vi "TrapControllers.vi"() -> ()   [LabVIEW 2017]
doc: "I. Description:\nThis example demonstrates how to continuously output a waveform using an internal sample clock. The automatic regeneration of data has been disabled, so new data has to be provided throughout the duration of the continuous Analog Output operation. This allows the generation of any arbitrary frequency as this VI computes new data for each iteration of the loop, maintaining phase continuity of the signal. The regeneration of data has also been adjusted so that the newest data is output as quickly as possible; thus reducing the lag between the changing of the data and the output of that data.\n\nII. Instructions for Running:\n1. Select the Physical Channel to correspond to where your signal is output on the DAQ device.\n2. Enter the Minimum and Maximum Voltage range.\n3. Specify the desired Sample Clock Rate of the output Waveform. Higher sample clock rates will produce a smoother waveform.\n4. Manually specify the Analog Output buffer size, in number of samples. A larger buffer would help non-regenerative operations avoid errors due to occasional high CPU load. \nNote: \nThe Analog Output buffer has to be at least as big as the amount of data being written to the board per iteration. The recommended buffer size would be at least twice the amount of data being written to the board per iteration.\n5. Enter the Waveform Information. See the documentation of the Basic Function Generator SubVI for information on each parameter.\n\nIII. Block Diagram Steps:\n1. Create an Analog Output Voltage channel.\n2. Configure the task to prohibit the automatic regeneration of data.\n2a. Set the transfer condition to Less than Full. Allows for more rapid updates of Output Buffer.\n3. Call the DAQmx (Sample Clock) VI to set the sample clock rate. Additionally, set the sample mode to Continuous.\n4. Read the actual sample clock rate (eventually coerced depending on the hardware used). \n5. Compute the desired waveform, using the buffer size and the actual update rate. This VI keeps track of the phase of the waveform to ensure that the generated signal is continuous.\n6. Write the waveform to the output buffer. \n7a. Call the Start VI. This is only needed when the loop is executed for the first time.\n7b. Do nothing.\n8. Loop continuously until user presses the Stop button. Every iteration computes and writes a new waveform to the buffer.\n9. Call the Clear Task VI to clear the Task.\n10. Use the popup dialog box to display an error or warning if any.\n\nIV. I/O Connections Overview:\nMake sure your signal output terminal matches the Physical Channel I/O Control. For further connection information, refer to your hardware reference manual."
uses:
  <vilib>/event_ctls.llb/eventvkey.ctl
  C:/Program Files/National Instruments/LabVIEW 2017/user.lib/Picomotor_8742/CmdLib.dll
  Program Files/National Instruments/LabVIEW 2017/user.lib/Picomotor_8742/CmdLib.dll
  <vilib>/DAQmx/write.llb/DAQmx Write (Analog DBL 1Chan 1Samp).vi
  <vilib>/DAQmx/write.llb/DAQmx Write (Digital 1D Bool NChan 1Samp 1Line).vi
  <vilib>/DAQmx/write.llb/DAQmx Write (Analog 1D DBL NChan 1Samp).vi
  <vilib>/DAQmx/create/channels.llb/DAQmx Create Channel (AO-Voltage-Basic).vi
  <vilib>/DAQmx/miscellaneous.llb/DAQmx Fill In Error Info.vi
  <vilib>/DAQmx/create/channels.llb/DAQmx Create Channel (DO-Digital Output).vi
  TrapSignal/Feedback.vi
  <vilib>/addons/control/pid/pid.llb/PID (DBL).vi
  PZT_PI/PZT_oscillation.vi
  <vilib>/addons/control/pid/NI_PID_pid.lvlib
  <vilib>/measure/NI_MABase.lvlib
panel:
  in  "Flu_Red_Run 2":bool caption="ON/OFF"
  out "LED_Power":dbl=3.0 caption="P (%)" min=0.0 max=100.0 step=1.0
  in  "LED_Power2":dbl=100.0 caption="P (%)" min=0.0 max=100.0 step=1.0
  in  "Trap_Power_Run 3":bool caption="Feedback"
  in  "MTAx_Feedback_dt 2":dbl=1.0 caption="Time (s)" format="%.1f"
  in  "?":cluster{dbl, dbl, dbl}={1.0, 0.01, 0.0} {"?" format="%.3f"; "?" format="%.3f"; "?" format="%.3f"}
  in  "Trap_Power_Run 2":bool caption="ON/Reset"
  in  "MTAy_Feedback_Reset":bool caption="Reset"
  in  "MTAy_Feedback_ON":bool caption="ON/Reset"
  in  "MTAy_Feedback_Min":dbl min=0.0 max=10.0 step=0.1 format="%#_2g"
  in  "MTAx_Feedback_Min":dbl caption="Min (pN)" min=0.0 max=10.0 step=0.1 format="%#_2g"
  in  "MTAy_Feedback_Max":dbl=0.01 min=0.0 max=10.0 step=0.1 format="%#_2g"
  in  "MTAx_Feedback_Reset":bool caption="Reset"
  in  "MTAx_Feedback_ON":bool caption="ON/Reset"
  in  "MTAy_Feedback_Force":dbl caption="Y" min=-10.0 max=10.0 step=0.1 format="%.1f"
  in  "?":cluster{dbl, dbl, dbl}={1.0, 5.0, 0.0} {"?" format="%.3f"; "?" format="%.3f"; "?" format="%.3f"}
  in  "MTAy_Feedback_dt":dbl=1.0 caption="Time (s)" format="%.1f"
  in  "MTAx_Feedback_Force":dbl caption="X" min=-10.0 max=10.0 step=0.1 format="%.1f"
  in  "?":cluster{dbl, dbl, dbl}={1.0, 5.0, 0.0} {"?" format="%.3f"; "?" format="%.3f"; "?" format="%.3f"}
  in  "MTAx_Feedback_dt":dbl=1.0 caption="Time (s)" format="%.1f"
  in  "MTAx_Feedback_Max":dbl=0.01 caption="Max (um)" min=0.0 max=10.0 step=0.1 format="%#_2g"
  in  "PM_Feedback":bool caption="ON/OFF"
  out "MTA_Limit":bool caption="Limit"
  out "MTA_Os_Num":i32
  in  "PZT_Speed 2":dbl=100.0 caption="Vel (%)" min=0.0 max=100.0 step=1.0
  in  "MTA_Select":bool caption="MTA1"
  out "MTA_Step":dbl=10.0 caption="Step (V)" min=0.0 max=1000.0 step=0.1 format="%.3f"
  in  "MTA_Step2":dbl=0.01 caption="Step2" min=0.0 max=1.0 step=0.001 format="%.3f"
  in  "MTA_Step_Select":bool=TRUE caption="(Y)"
  in  "MTA_Step1":dbl=0.1 caption="Step1" min=0.0 max=1.0 step=0.001 format="%.3f"
  in  "MTAY-":bool
  in  "MTAY+":bool
  in  "MTAX+":bool
  in  "MTAX-":bool
  out "MTA2Y":dbl caption="Pos (um)" format="%.3f"
  out "MTA2X":dbl caption="Pos (um)" format="%.3f"
  out "MTA1Y":dbl caption="Y" format="%.3f"
  out "MTA1X":dbl caption="X" format="%.3f"
  out "MTA_Manual_ON":bool caption="Manual"
  in  "MTA_Zero":bool
  in  "MTA_Home":bool
  in  "MTA_STOP":bool
  out "MTA_Man_Num":i32
  out "MTA_ON":bool
  in  "MTA_START":bool
  in  "STOP 2":bool
  in  "PZT_Zero":bool
  in  "LED_Power 2":dbl=10.0 caption="TIRF angle" min=0.0 max=100.0 step=1.0
  in  "LED_STOP":bool
  out "LED_Num":i32
  in  "LED_Run":bool caption="P (%)"
  out "LED_ON":bool
  in  "LED_Power1":dbl=10.0 caption="P (%)" min=0.0 max=100.0 step=1.0
  in  "LED_START":bool
  out "PZT_Manual_ON":bool caption="Manual"
  out "PZTZ_Step":dbl=10.0 caption="Step (nm)" min=0.0 max=1000.0 step=1.0
  in  "PZTZ_Step2":dbl=20.0 caption="Step (nm)" min=0.0 max=1000.0 step=1.0
  in  "PZTZ_Step1":dbl=100.0 caption="Step (nm)" min=0.0 max=1000.0 step=1.0
  out "PZTY_Step":dbl=10.0 caption="Step (nm)" min=0.0 max=1000.0 step=1.0
  in  "PZTY_Step2":dbl=20.0 caption="Step (nm)" min=0.0 max=1000.0 step=1.0
  in  "PZTY_Step1":dbl=100.0 caption="Step (nm)" min=0.0 max=1000.0 step=1.0
  out "PZTZ_Limit":bool caption="Limit"
  out "PZTY_Limit":bool caption="Limit"
  out "PZTX_Step":dbl=10.0 caption="Step (nm)" min=0.0 max=1000.0 step=1.0
  in  "PZTX_Step2":dbl=20.0 caption="Step (nm)" min=0.0 max=1000.0 step=1.0
  in  "PZT_Step_Select":bool=TRUE caption="(Del)"
  in  "Det_Select":bool caption="Det 1"
  out "Det_Step":dbl=10.0 caption="Step (um)" min=0.0 max=1000.0 step=0.1
  in  "Det2_Offset":bool
  in  "Det1_Offset":bool
  in  "Det2_Home":bool
  out "Detection2Y_Position":dbl caption="Pos (um)"
  out "Detection2X_Position":dbl caption="Pos (um)"
  out "Detection1Y_Position":dbl caption="Y"
  in  "Det_Step2":dbl=1.0 caption="Step2" min=0.0 max=100.0 step=1.0
  in  "Detection_Step_Select":bool=TRUE caption="(O)"
  in  "Det_Step1":dbl=10.0 caption="Step1" min=0.0 max=100.0 step=1.0
  in  "Det1_Home":bool
  out "Detection1X_Position":dbl caption="X"
  in  "Det_Position_STOP":bool
  out "Det_Position_Num":i32
  in  "Det_Position_START":bool
  out "Detection_Position_ON":bool caption="Picomotor"
  in  "DetY-":bool
  in  "DetY+":bool
  in  "DetX+":bool
  in  "DetX-":bool
  in  "Detection_Power":dbl=50.0 caption="Power (%)" min=0.0 max=100.0 step=1.0
  out "Controllers_ON":bool
  in  "Trap_Select":bool caption="Trap1"
  out "Trap_Step":dbl=10.0 caption="Step (um)" min=0.0 max=1000.0 step=0.1
  in  "Trap2_Offset":bool
  in  "Trap1_Offset":bool
  in  "Trap2_Home":bool
  out "PicomotorError":errorcluster
  out "PicomotorDevice2":string
  out "PicomotorCmdLib":refnum<k24>
  out "PicomotorDevice1":string
  out "Trap2Y_Position":dbl caption="Pos (um)"
  out "Trap2X_Position":dbl caption="Pos (um)"
  out "Trap1Y_Position":dbl caption="Y"
  in  "Trap_Step2":dbl=1.0 caption="Step2" min=0.0 max=100.0 step=1.0
  in  "Trap_Step_Select":bool=TRUE caption="(E)"
  in  "Trap_Step1":dbl=10.0 caption="Step1" min=0.0 max=100.0 step=1.0
  in  "Trap1_Home":bool
  out "Trap1X_Position":dbl caption="X"
  in  "Trap_Position_STOP":bool
  out "Trap_Position_Num":i32
  in  "Trap_Position_START":bool
  out "PZT_Man_Num":i32
  in  "PZTX_Step1":dbl=100.0 caption="Step (nm)" min=0.0 max=1000.0 step=1.0
  out "PZTZ_Position":dbl caption="Z"
  out "PZTY_Position":dbl caption="Y"
  out "PZTX_Position":dbl caption="X"
  out "PZTX_Limit":bool caption="Limit"
  in  "PZT_Speed":dbl=100.0 caption="Vel (%)" min=0.0 max=100.0 step=1.0
  in  "PZT_Home":bool
  in  "PZT_Z-":bool
  in  "PZT_Z+":bool
  in  "PZT_Y-":bool
  in  "PZT_Y+":bool
  in  "PZT_X+":bool
  in  "PZT_X-":bool
  in  "PZT_oscillation_Run":bool caption="Start (Shift)"
  out "PZT_Os_Num":i32
  in  "PZT_Amplitude":dbl=50.0 caption="Amp (nm)" min=0.0 max=100.0 step=1.0
  in  "PZT_Frequency":dbl=100.0 caption="Freq (Hz)" min=0.0 max=100.0 step=1.0
  in  "PZT_Waveform":enum16{"Sine", "Triangle", "Square", "Sawtooth"}(ring) caption="Waveform"
  in  "PZT_Axis":enum16{"X", "Y", "Z"}(ring) caption="Axis"
  out "PZT_ON":bool
  in  "PZT_START":bool
  in  "PZT_STOP":bool
  out "Trap_Position_ON":bool caption="Picomotor"
  in  "TrapY-":bool
  in  "TrapY+":bool
  in  "TrapX+":bool
  in  "TrapX-":bool
  in  "Trap_Power_Run":bool caption="ON/OFF"
  in  "Trap_Power_Input":dbl=20.0 caption="%" min=0.0 max=100.0 step=1.0
  in  "Trap_Power_STOP":bool
  out "Trap_Power_Num":i32
  in  "Trap_Power_START":bool
  out "Trap_Power_ON":bool caption="Power"
  in  "StageY_Home 2":bool
  in  "VISA_Close":bool caption="Close"
  in  "StageZ_Step2":dbl=1.0 caption="Step2" min=0.0 max=10.0 step=0.01 format="%.2f"
  in  "StageZ_Step1":dbl=2.0 caption="Step1" min=0.0 max=10.0 step=0.01 format="%.2f"
  out "StageZ_Step":dbl=10.0 caption="Step (um)" min=0.0 max=1000.0 step=0.1 format="%.2f"
  out "StageZ_ON":bool caption="Z"
  out "StageZ_Position":dbl caption="Position" format="%.2f"
  in  "VISA_Selection":refnum<visa-resource-name> caption="VISA"
  in  "StageZ_Start":bool
  in  "StageY_Start":bool
  out "StageY_ON":bool caption="Y"
  in  "StageY_Home":bool
  out "StageY_Position":dbl caption="Pos (um)" format="%.1f"
  in  "StageY_Step2":dbl=5.0 caption="Step2" min=0.0 max=1000.0 step=0.1 format="%.1f"
  in  "StageY_Step1":dbl=10.0 caption="Step1" min=0.0 max=1000.0 step=0.1 format="%.1f"
  out "StageY_Step":dbl=10.0 caption="Step (um)" min=0.0 max=1000.0 step=0.1 format="%.1f"
  out "StageX_Step":dbl=10.0 caption="Step (um)" min=0.0 max=1000.0 step=0.1 format="%.1f"
  in  "StageX_Step2":dbl=5.0 caption="Step2" min=0.0 max=1000.0 step=0.1 format="%.1f"
  in  "Stage_Step_Select":bool=TRUE caption="(5)"
  out "Numeric":i32
  out "StageX_ON":bool caption="X"
  in  "StageZ_Stop":bool
  in  "StageY_Stop":bool
  in  "StageX_Stop":bool
  in  "StageZ-":bool
  in  "StageZ+":bool
  in  "StageY-":bool
  in  "StageY+":bool
  in  "StageX+":bool
  in  "StageX-":bool
  out "StageY_Limit 2":bool caption="Limit"
  out "StageY_Limit":bool caption="Limit"
  out "StageX_Limit":bool caption="Limit"
  in  "StageX_Step1":dbl=10.0 caption="Step1" min=0.0 max=1000.0 step=0.1 format="%.1f"
  in  "StageX_Home":bool
  out "?":i32
  out "?":i32
  out "StageX_Position":dbl caption="Pos (um)" format="%.1f"
  in  "StageX_Start":bool
  out "VKey":T1
  out "Char":i16
  out "ScanCode":i16
  in  "Flu_Red_Run":bool caption="640"
  in  "Flu_Green_Run":bool caption="561"
  in  "Flu_Blue_Run":bool caption="488"
  in  "stop 6":bool
  out "Numeric 9":i32
  out "FluorescenceLaser_ON":bool
  in  "OK Button 6":bool
  in  "Detection_Power_Run":bool caption="ON/OFF"
  in  "Detection_Power_STOP":bool
  out "Det_Power_Num":i32
  in  "Detection_Power_START":bool
  out "Detection_Power_ON":bool caption="Power"
  in  "stop 5":bool
  out "Numeric 8":i32
  in  "OK Button 5":bool
  out "OK Button 9":bool
  in  "STOP":bool
  # "Trap"
  # "Trap Laser"
  # "Sample Stage"
  # "PM"
  # "Num Lock should be ON (default)"
  # "Force clamp"
  # "Trap1"
  # "Trap2"
  # "F (pN)"
  # "MTA1"
  # "Feedback"
  # "MTA2"
  # "Trap2"
  # "Range\nX/Y = +/- 2.5 mm\nZ = +/- 10 um"
  # "Kc"
  # "Kc"
  # "Ti (s)"
  # "MTA2"
  # "Ti (m)"
  # "Detection Laser"
  # "Piezo Stage"
  # "Illumination Light"
  # "Template"
  # "LED"
  # "RGB Lasers"
  # "Det 1"
  # "Oscillation"
  # "Feedback"
  # "Det 2"
  # "Pos (nm)"
  # "Position feedback"
  # "Force feedback"
  # "Det 2"
  # "P max = 200 mW"
  # "X/Y = +/- 5 um\nZ = +/- 3 um"
  # "Imax = 350 mA (5 V)"
  # "* Program START >> Wait for a few sec until ON >> Start sub-programs \n* Stop sub-programs first >> STOP PROGRAM\n* Serial ports: StageX (COM3), StageY (COM7), StageZ (COM8), OBIS (COM11)\n* If StageXY are reconnected (orange light), then run CONEX-CC to reinitialize. \n* Piezo Stage , MTA: Home (after start), Zero (before end)"
  # "Picomotors"
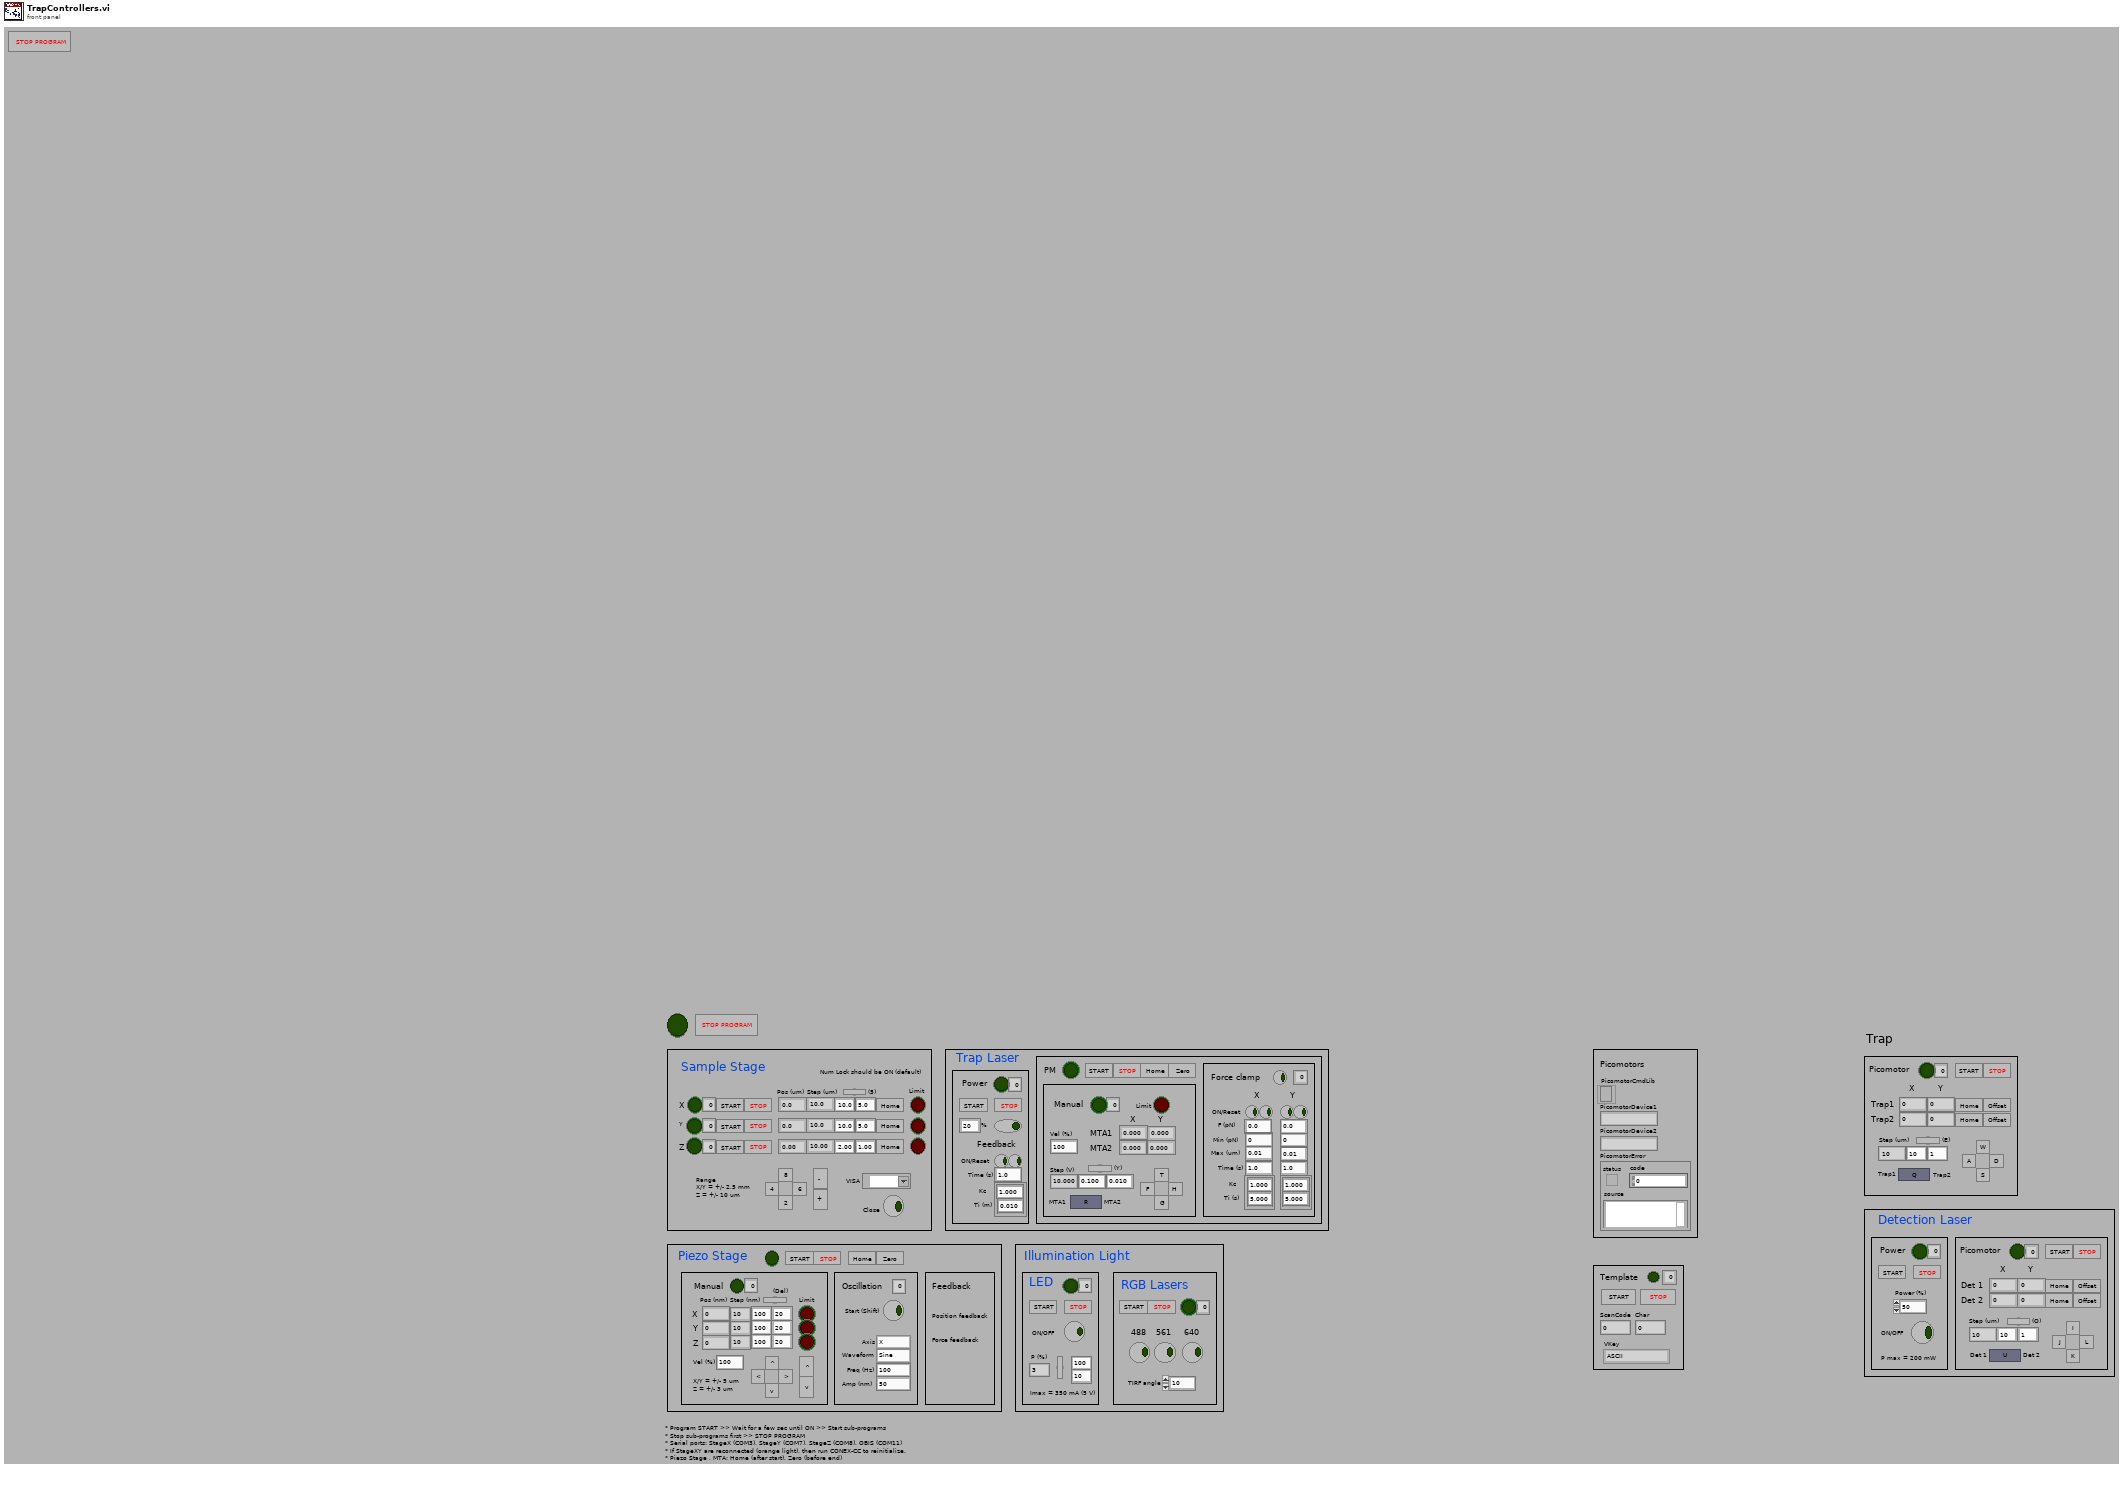
[diagram p1: front panel]
types:
  T1 = typedef "eventvkey.ctl" = enum16{"ASCII", "Enter", "Return", "Shift", "Ctrl", "Alt", "Cmd", "Opt", "Caps", "NumLock", "Clear", "Break", "Up", "Down", "Left", "Right", "Insert", "Delete", "Home", "End", "PageUp", "PageDown", "Escape", "Help", "Pause", "ScrollLock", "F1", "F2", "F3", "F4", "F5", "F6", "F7", "F8", "F9", "F10", "F11", "F12", "F13", "F14", "F15", "F16", "F17", "F18", "F19", "F20", "F21", "F22", "F23", "F24", "Play", "VolumeUp", "VolumeDown", "Mute", "Two Byte Char"}
  T2 = cluster{"MTA1X":dbl, "MTA1Y":dbl, "MTA2X":dbl, "MTA2Y":dbl}
  T3 = cluster{"VISA resource name":refnum<visa-resource-name>, "Device name":string, "Controller address":i32, "error":errorcluster}
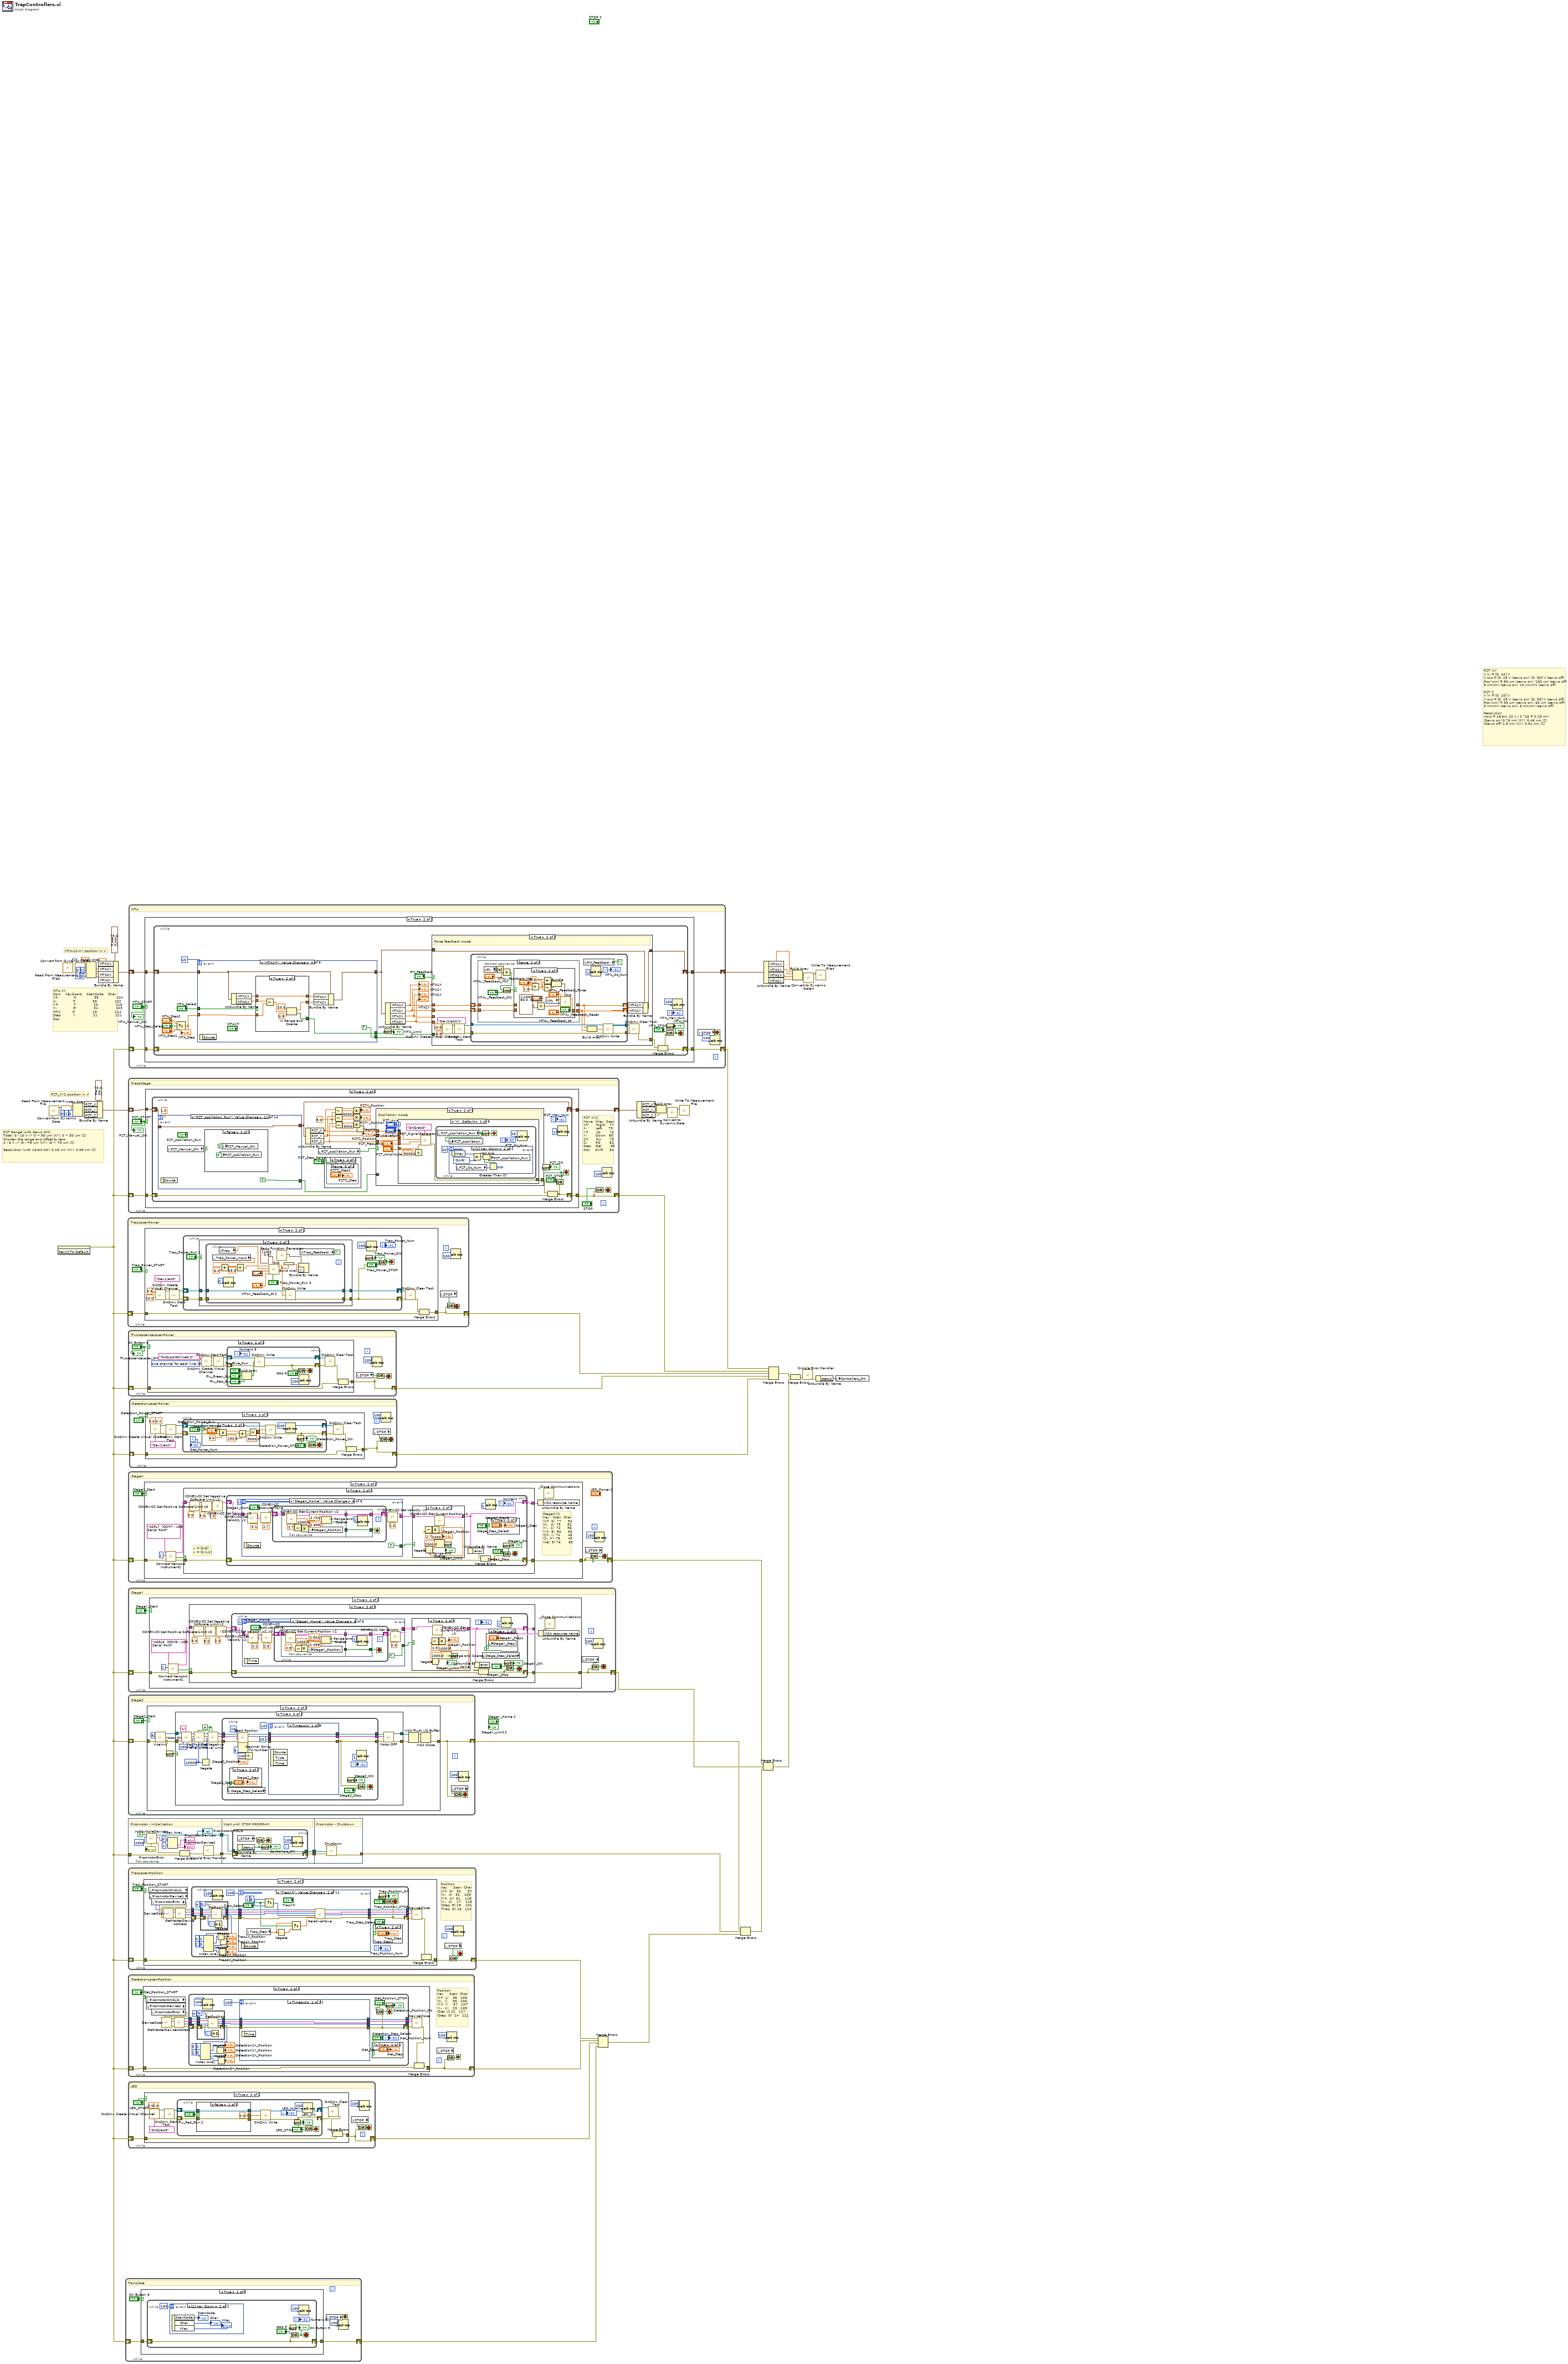
[diagram p0: block diagram]
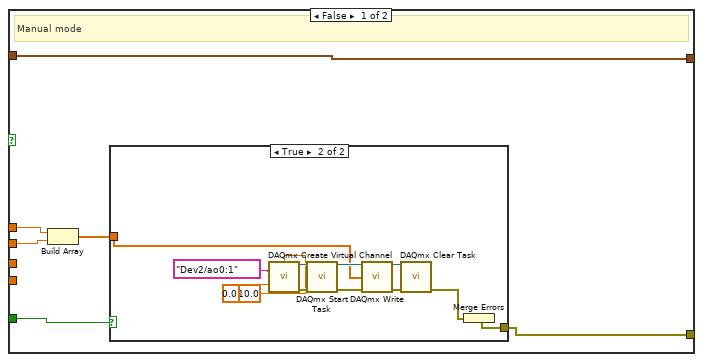
[diagram p3: hidden frame]
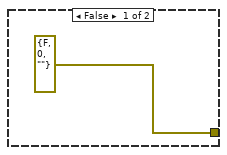
[diagram p4: hidden frame]
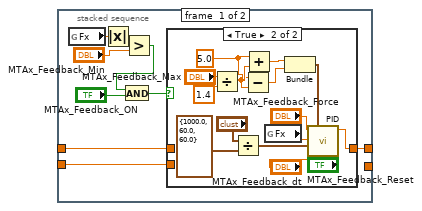
[diagram p5: hidden frame]
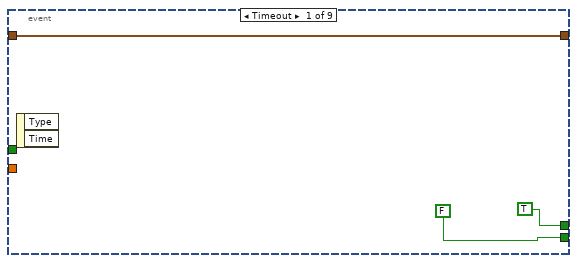
[diagram p8: hidden frame]
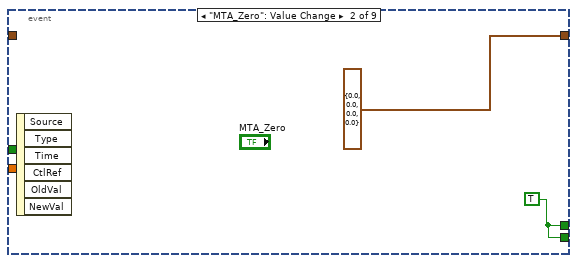
[diagram p9: hidden frame]
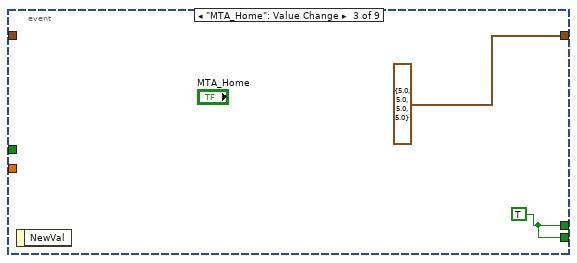
[diagram p10: hidden frame]
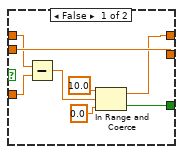
[diagram p11: hidden frame]
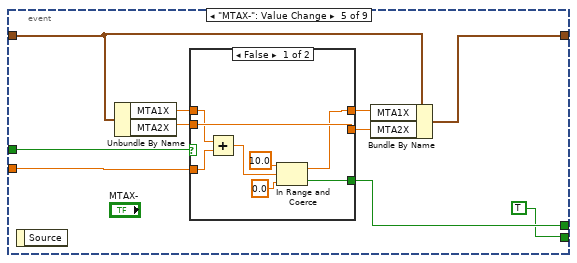
[diagram p12: hidden frame]
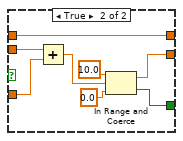
[diagram p13: hidden frame]
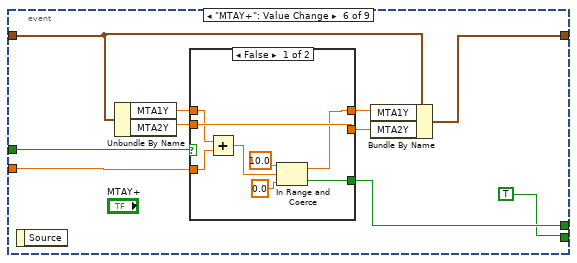
[diagram p14: hidden frame]
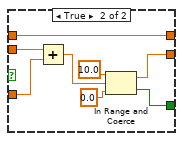
[diagram p15: hidden frame]
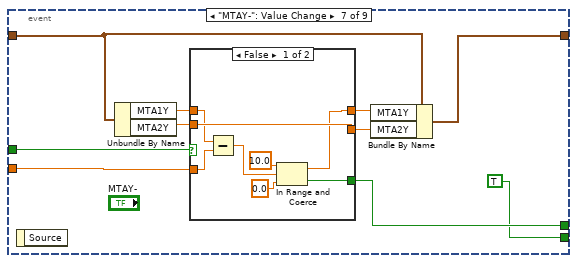
[diagram p16: hidden frame]
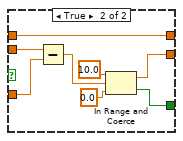
[diagram p17: hidden frame]
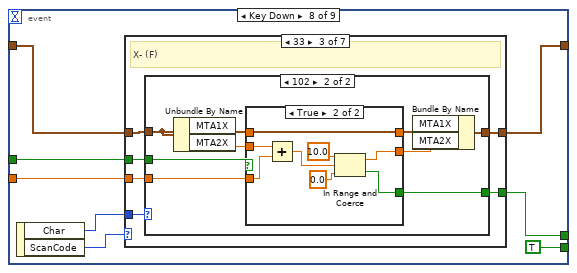
[diagram p18: hidden frame]
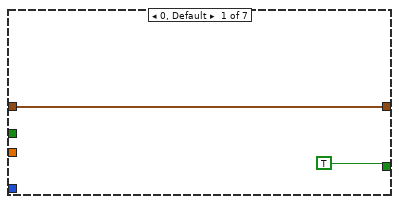
[diagram p19: hidden frame]
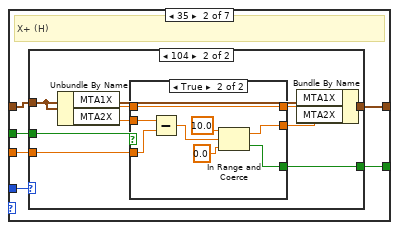
[diagram p20: hidden frame]
diagram:
  # "MTA XY\nCom    Keyboard    ScanCode    Char\nX+              H                35                104\nX-               F                33                102\nY+              T                20                116\nY-               G                34                103        \nMTA           R                19                114\nStep           Y                21                121\nOsc"
  # "MTA-12-XY position in V"
  # "PZT_XYZ position in V"
  # "PZT Range (with Servo ON):\nTotal: 0 - 10 V -> 0 ~ 50 um (XY), 0 ~ 30 um (Z)\nShorten the range and offset to zero: \n4 - 6 V -> -5 - +5 um (XY), -3 ~ +3 um (Z)\n\nResolution (with 16-bit AO): 0.15 nm (XY), 0.09 nm (Z)"
  # "PZT X/Y\nV in = [0, 10] V\nV out = [0, 25 V (servo on), [0, 50] V (servo off)\nPos (um) = 50 um (servo on), 100 um (servo off)\n5 nm/mV (servo on), 10 nm/mV (servo off)\n\nPZT Z\nV in = [0, 10] V\nV out = [0, 25 V (servo on), [0, 50] V (servo off)\nPos (um) = 30 um (servo on), 60 um (servo off)\n3 nm/mV (servo on), 6 nm/mV (servo off)\n\nResolution\nVout = 16-bit, 10 V / 2^16 = 0.15 mV\n(Servo on) 0.76 nm (XY), 0.46 nm (Z)\n(Servo off) 1.5 nm (XY), 0.91 nm (Z)"
  n1 = call "Read From Measurement File"() -> ("Signals"=w57:dynamicdata)  [unwired: 6 in, 5 out]
  n2 = invoke on="STOP" class="Bool (strict)" method="Reinit To Default"() -> (error out=w2:errorcluster)  [unwired: 3 in, 2 out]
  n3 = call "Convert from Dynamic Data"("Dynamic Data Type"=w57) -> ("Array"=w56:dbl[])  [unwired: 3 in]
  n4 = call "Read From Measurement File2"() -> ("Signals"=w16:dynamicdata)  [unwired: 6 in, 5 out]
  n5 = Index Array(array=w56, index #1=0 ("index"), index #2=1 ("index"), index #3=2 ("index")) -> (element #1=w52:dbl, element #2=w51:dbl, element #3=w50:dbl)
  n6 = call "Convert from Dynamic Data2"("Dynamic Data Type"=w16) -> ("Array"=w21:dbl[])  [unwired: 3 in]
  n7 = Bundle By Name(cluster=cluster{"PZT_X":dbl, "PZT_Y":dbl, "PZT_Z":dbl} {"PZT_X"=5.0, "PZT_Y"=5.0, "PZT_Z"=5.0} ("output cluster"), "PZT_X"=w52, "PZT_Y"=w51, "PZT_Z"=w50) -> (w43:cluster{"PZT_X":dbl, "PZT_Y":dbl, "PZT_Z":dbl})
  n8 = Index Array(array=w21, index #1=0 ("index"), index #2=1 ("index"), index #3=2 ("index"), index #4=3 ("index")) -> (element #1=w14:dbl, element #2=w13:dbl, element #3=w12:dbl, element #4=w11:dbl)
  n9 = Bundle By Name(cluster=T2 {"MTA1X"=5.0, "MTA1Y"=5.0, "MTA2X"=5.0, "MTA2Y"=5.0} ("output cluster"), "MTA1X"=w14, "MTA1Y"=w13, "MTA2X"=w12, "MTA2Y"=w11) -> (w10:T2)
  n10 = while {
    shift-right: [w61] -> w1
    shift-left: w2 -> [w62]
    stop <- w65 stop-if-true
    # "Template"
    n11 = case shown="True" "OK Button 5" {
      tunnel: w62 -> [w66 w68]
      tunnel: [w66 w67] -> w61
      frame False {
      }
      frame True {
        n12 = while "Event Handle Loop" {
          shift-right: [w69] -> w67
          shift-left: w68 -> [w69]
          i -> [w73]
          stop <- w71 stop-if-true
          # "Template"
          n13 = event shown="[1] Key Down" {
            selector: _ -> [_ _]
            dyn-events: _ -> [_ _]
            timeout: 100 -> [_ _]
            event Timeout {
              n14 = event-data() -> ()  [unwired: 1 in, 2 out]
            }
            event Key Down {
              n15 = event-data() -> ("ScanCode"=→"ScanCode":i16, "Char"=→"Char":i16, "VKey"=→"VKey":T1)  [unwired: 1 in]
            }
          }
          n16 = Or(x="stop 5", y=w69) -> (x .or. y?=w71:bool)
          n17 = Not(x=w71) -> (.not. x?=→"OK Button 9":bool)
          n18 = Wait (ms)(milliseconds to wait=u32 100) -> ()  [unwired: 1 out]
          "Numeric 8" <- w73
        }
      }
    }
    n19 = local read "STOP"() -> (w65:bool)
    n20 = Wait (ms)(milliseconds to wait=u32 100) -> ()  [unwired: 1 out]
  }
  n21 = while {
    shift-right: [w79] -> w59
    shift-left: w2 -> [w80]
    stop <- w82 stop-if-true
    # "TrapLaser-Power"
    n22 = case shown="True" "Trap_Power_START" {
      tunnel: [w85 w86] -> w79
      tunnel: w80 -> [w85 w87]
      frame False {
      }
      frame True {
        n23 = call-poly <vilib>:"DAQmx Create Virtual Channel.vi"("maximum value"=10.0, "minimum value"=0.0, "physical channels"=tag "Dev1/ao0") -> ("task out"=w93:refnum<k21>, "error out"=w97:errorcluster)  [unwired: 11 in]
        n24 = call <vilib>:"DAQmx Start Task.vi"("task/channels in"=w93, "error in"=w97) -> ("task out"=w92:refnum<k21>, "error out"=w91:errorcluster)  [unwired: 12 in]
        n25 = while "Event Handle Loop" {
          shift-right: [w99] -> w90
          shift-left: w92 -> [w100]
          shift-right: [w98] -> w89
          shift-left: w91 -> [w101]
          i -> [w106]
          stop <- w104 stop-if-true
          # "Trap Laser"
          n26 = case shown="True" "Trap_Power_Run 2" {
            tunnel: w101 -> [w112 w123]
            tunnel: w100 -> [w113 w122]
            tunnel: [w111 w121] -> w98
            tunnel: [w110 w120] -> w99
            frame False {
              n27 = case shown="True" "Trap_Power_Run" {
                tunnel: [0.0 ("Trap_control") w119] -> w108
                frame False {
                }
                frame True {
                  n28 = Add(x="Trap_Power_Input", y=6.4) -> (x+y=w116:dbl)
                  n29 = Divide(x=w116, y=11.0) -> (x/y=w119:dbl)
                }
              }
              n30 = call-poly <vilib>:"DAQmx Write.vi"("task/channels in"=w113, "data"=w108, "error in"=w112) -> ("task out"=w110:refnum<k21>, "error out"=w111:errorcluster)  [unwired: 10 in, 1 out]
            }
            frame True {
              n31 = while {
                tunnel: w123 -> [w139]
                tunnel: w122 -> [w138]
                tunnel: [w137] -> w120
                tunnel: [w136] -> w121
                stop <- w141 continue-if-true
                n32 = local read "Trap_Power_Input"() -> (w131:dbl)
                n33 = global read "Feedback.vi" "Trap"() -> (w142:dbl)
                n34 = Add(x=w131, y=6.4) -> (x+y=w133:dbl)
                n35 = Wait (ms)(milliseconds to wait=u32 1) -> ()  [unwired: 1 out]
                n36 = Divide(x=w133, y=25.0) -> (x/y=w130:dbl)
                n37 = call-poly <vilib>:"PID.vi"("reinitialize? (F)"="Trap_Power_Run 3", "output range"=cluster{"output high":dbl, "output low":dbl} {"output high"=10.0, "output low"=0.0}, "dt (s)"="MTAx_Feedback_dt 2", "PID gains"="?", "process variable"=w142, "setpoint"=w130) -> ("output"=w126:dbl)  [unwired: 4 in, 1 out]
                n38 = call <vilib>:"Basic Function Generator.vi"() -> ("signal out"=w124:waveform(dbl))  [unwired: 9 in, 2 out]
                n39 = Build Array(w126) -> (w125:dbl[])
                n40 = call-poly <vilib>:"DAQmx Write.vi"("task/channels in"=w138, "data"=w126, "error in"=w139) -> ("task out"=w137:refnum<k21>, "error out"=w136:errorcluster)  [unwired: 10 in, 1 out]
                n41 = Bundle By Name(cluster=w124, "Y"=w125) -> ()  [unwired: 1 out]
                n42 = global read "Feedback.vi" "Trap_Feedback"() -> (w141:bool)
              }
            }
          }
          n43 = Wait (ms)(milliseconds to wait=u32 100) -> ()  [unwired: 1 out]
          n44 = Or(x=w98, y="Trap_Power_STOP") -> (x .or. y?=w104:bool)
          n45 = Not(x=w104) -> (.not. x?=→"Trap_Power_ON":bool)
          "Trap_Power_Num" <- w106
        }
        n46 = call <vilib>:"DAQmx Clear Task.vi"("task in"=w90, "error in"=w89) -> ("error out"=w88:errorcluster)  [unwired: 13 in]
        n47 = Merge Errors(w88, w87) -> (w86:errorcluster)
      }
    }
    n48 = local read "STOP"() -> (w81:bool)
    n49 = Or(x=w81, y=w79) -> (x .or. y?=w82:bool)
    n50 = Wait (ms)(milliseconds to wait=u32 100) -> ()  [unwired: 1 out]
  }
  n51 = flat-sequence {
    tunnel: w2 -> [w154]
    tunnel: [w145] -> w29
    tunnel: [w147] -> w27
    tunnel: w29 -> [w158]
    tunnel: [w157] -> w28
    tunnel: w27 -> [w156]
    tunnel: [w155] -> w26
    tunnel: [w166] -> w33
    tunnel: w28 -> [w167]
    tunnel: w26 -> [w168]
    frame #0 {
      # "Picomotor - Initialization"
      n52 = call "InitMultipleDevices.vi"("msecDelayForDiscovery"=2000, "logging"=FALSE) -> ("error out"=w148:errorcluster, "DeviceKey List Out"=w151:string[], "CmdLib Out"=w147:refnum<k24>)  [unwired: 3 in]
      "PicomotorCmdLib" <- w147
      "PicomotorError" <- w148
      n53 = Index Array(array=w151, index #1=0 ("index"), index #2=1 ("index")) -> (element #1=→"PicomotorDevice1":string, element #2=→"PicomotorDevice2":string)
      n54 = Merge Errors(w148, w154) -> (w146:errorcluster)
      n55 = call <vilib>:"Simple Error Handler.vi"("error in (no error)"=w146) -> ("error out"=w145:errorcluster)  [unwired: 4 in, 4 out]
    }
    frame #1 {
      # "Wait until STOP PROGRAM"
      n56 = while {
        tunnel: w156 -> [w164]
        tunnel: [w164] -> w155
        shift-right: [w163] -> w157
        shift-left: w158 -> [w163]
        stop <- w161 stop-if-true
        n57 = Unbundle By Name(w163) -> ("status"=w160:bool)
        n58 = local read "STOP"() -> (w162:bool)
        n59 = Or(x=w162, y=w160) -> (x .or. y?=w161:bool)
        n60 = Not(x=w160) -> (.not. x?=→"Controllers_ON":bool)
        n61 = Wait (ms)(milliseconds to wait=u32 100) -> ()  [unwired: 1 out]
      }
    }
    frame #2 {
      # "Picomotor - Shutdown"
      n62 = call "Shutdown.vi"("error in (no error)"=w167, "CmdLib In"=w168) -> ("error out"=w166:errorcluster)  [unwired: 4 in, 1 out]
    }
  }
  n63 = while {
    shift-right: [w170] -> w23
    shift-left: w2 -> [w173]
    stop <- w172 stop-if-true
    # "LED"
    n64 = case shown="True" "LED_START" {
      tunnel: w173 -> [w175 w178]
      tunnel: [w175 w176] -> w170
      frame False {
      }
      frame True {
        n65 = call-poly <vilib>:"DAQmx Create Virtual Channel.vi"("maximum value"=5.0, "minimum value"=0.0, "physical channels"=tag "DAQ/ao3") -> ("task out"=w183:refnum<k21>, "error out"=w187:errorcluster)  [unwired: 11 in]
        n66 = call <vilib>:"DAQmx Start Task.vi"("task/channels in"=w183, "error in"=w187) -> ("task out"=w182:refnum<k21>, "error out"=w181:errorcluster)  [unwired: 12 in]
        n67 = while "Event Handle Loop" {
          shift-right: [w195] -> w180
          shift-left: w182 -> [w192]
          shift-right: [w193] -> w179
          shift-left: w181 -> [w191]
          i -> [w200]
          stop <- w198 stop-if-true
          # "Detection Laser"
          n68 = case shown="False" "Flu_Red_Run 2" {
            tunnel: [0.0 w208] -> w196
            tunnel: w192 -> [w203 w207]
            tunnel: w191 -> [w202 w206]
            tunnel: [w203 w205] -> w190
            tunnel: [w202 w204] -> w189
            frame False {
            }
            frame True {
              n69 = case shown="True" "LED_Run" {
                tunnel: [w213 w218] -> w208
                tunnel: w207 -> [w211 w216]
                tunnel: w206 -> [w210 w215]
                tunnel: [w211 w216] -> w205
                tunnel: [w210 w215] -> w204
                frame False {
                  n70 = local write "LED_Power"("LED_Power1") -> ()
                  n71 = Divide(x="LED_Power1", y=20.0) -> (x/y=w213:dbl)
                }
                frame True {
                  n72 = Divide(x="LED_Power2", y=20.0) -> (x/y=w218:dbl)
                  "LED_Power" <- "LED_Power2"
                }
              }
            }
          }
          n73 = call-poly <vilib>:"DAQmx Write.vi"("task/channels in"=w190, "data"=w196, "error in"=w189) -> ("task out"=w195:refnum<k21>, "error out"=w193:errorcluster)  [unwired: 10 in, 1 out]
          n74 = Wait (ms)(milliseconds to wait=u32 100) -> ()  [unwired: 1 out]
          n75 = Or(x=w193, y="LED_STOP") -> (x .or. y?=w198:bool)
          n76 = Not(x=w198) -> (.not. x?=→"LED_ON":bool)
          "LED_Num" <- w200
        }
        n77 = call <vilib>:"DAQmx Clear Task.vi"("task in"=w180, "error in"=w179) -> ("error out"=w177:errorcluster)  [unwired: 13 in]
        n78 = Merge Errors(w177, w178) -> (w176:errorcluster)
      }
    }
    n79 = local read "STOP"() -> (w171:bool)
    n80 = Or(x=w171, y=w170) -> (x .or. y?=w172:bool)
    n81 = Wait (ms)(milliseconds to wait=u32 100) -> ()  [unwired: 1 out]
  }
  n82 = while "PZT_Loop" {
    shift-right: [w226] -> w46
    shift-left: w43 -> [w227]
    shift-right: [w221] -> w60
    shift-left: w2 -> [w222]
    stop <- w224 stop-if-true
    # "PZT XYZ\nMove  VKey  Scan\nX+       Right    77\nX-        Left      75\nY+       Up        72\nY-        Down   80\nZ+       PU        73\nZ-        PD        81\nStep    Del        83\nOsc     Shift      54"
    # "PiezoStage"
    n83 = case shown="True" "PZT_START" {
      tunnel: w227 -> [w229 w233]
      tunnel: [w229 w232] -> w226
      tunnel: [w228 w231] -> w221
      tunnel: w222 -> [w228 w230]
      frame False {
      }
      frame True {
        n84 = while "Event Handle Loop" {
          shift-right: [w258] -> w232
          shift-left: w233 -> [w259]
          shift-right: [w252] -> w231
          shift-left: w230 -> [w248]
          i -> [w254]
          stop <- w256 stop-if-true
          w236 = 5000.0 ("y")
          w242 = 5.0 ("y")
          # "PZT"
          n85 = event shown="[10] \"PZT_oscillation_Run\": Value Change" {
            selector: _ -> [_ _ _ _ _ _ _ _ _ _ _ _ _ _]
            dyn-events: _ -> [_ _ _ _ _ _ _ _ _ _ _ _ _ _]
            timeout: 1.0 -> [_ _ _ _ _ _ _ _ _ _ _ _ _ _]
            tunnel: w259 -> [w348 w359 w372 w385 w398 w411 w424 w430 w434 w550 w650 w657 w664 w672]
            tunnel: [w348 w360 w373 w386 w399 w412 w425 w429 w433 w549 w650 w657 w664 w671] -> w258
            tunnel: [FALSE TRUE TRUE TRUE TRUE TRUE TRUE TRUE TRUE TRUE TRUE FALSE FALSE TRUE] -> w247
            event Timeout {
              n86 = event-data() -> ()  [unwired: 1 in, 1 out]
            }
            event "PZT_X+": Value Change {
              n87 = event-data() -> ()  [unwired: 1 in, 1 out]
              n88 = local read "PZTX_Step"() -> (w353:dbl)
              n89 = Unbundle By Name(w359) -> ("PZT_X"=w361:dbl)
              n90 = Divide(x=w353, y=5000.0) -> (x/y=w350:dbl)
              n91 = Subtract(x=w361, y=w350) -> (x-y=w356:dbl)
              n92 = In Range and Coerce(upper limit=9.0, x=w356, lower limit=1.0) -> (coerced(x)=w355:dbl, In Range?=w354:bool)
              n93 = Bundle By Name(cluster=w359, "PZT_X"=w355) -> (w360:cluster{"PZT_X":dbl, "PZT_Y":dbl, "PZT_Z":dbl})
              n94 = Not(x=w354) -> (.not. x?=w352:bool)
              n95 = local write "PZTX_Limit"(w352) -> ()
            }
            event "PZT_X-": Value Change {
              n96 = event-data() -> ()  [unwired: 1 in, 1 out]
              n97 = local read "PZTX_Step"() -> (w366:dbl)
              n98 = Unbundle By Name(w372) -> ("PZT_X"=w374:dbl)
              n99 = Divide(x=w366, y=5000.0) -> (x/y=w363:dbl)
              n100 = Add(x=w374, y=w363) -> (x+y=w369:dbl)
              n101 = In Range and Coerce(upper limit=9.0, x=w369, lower limit=1.0) -> (coerced(x)=w368:dbl, In Range?=w370:bool)
              n102 = Bundle By Name(cluster=w372, "PZT_X"=w368) -> (w373:cluster{"PZT_X":dbl, "PZT_Y":dbl, "PZT_Z":dbl})
              n103 = Not(x=w370) -> (.not. x?=w365:bool)
              n104 = local write "PZTX_Limit"(w365) -> ()
            }
            event "PZT_Y+": Value Change {
              n105 = event-data() -> ()  [unwired: 1 in, 1 out]
              n106 = local read "PZTY_Step"() -> (w379:dbl)
              n107 = Unbundle By Name(w385) -> ("PZT_Y"=w387:dbl)
              n108 = Divide(x=w379, y=5000.0) -> (x/y=w376:dbl)
              n109 = Add(x=w387, y=w376) -> (x+y=w382:dbl)
              n110 = In Range and Coerce(upper limit=9.0, x=w382, lower limit=ext 1.0) -> (coerced(x)=w381:ext, In Range?=w383:bool)
              n111 = Bundle By Name(cluster=w385, "PZT_Y"=w381) -> (w386:cluster{"PZT_X":dbl, "PZT_Y":dbl, "PZT_Z":dbl})
              n112 = Not(x=w383) -> (.not. x?=w378:bool)
              n113 = local write "PZTY_Limit"(w378) -> ()
            }
            event "PZT_Y-": Value Change {
              n114 = event-data() -> ()  [unwired: 1 in, 1 out]
              n115 = local read "PZTY_Step"() -> (w392:dbl)
              n116 = Unbundle By Name(w398) -> ("PZT_Y"=w400:dbl)
              n117 = Divide(x=w392, y=5000.0) -> (x/y=w389:dbl)
              n118 = Subtract(x=w400, y=w389) -> (x-y=w394:dbl)
              n119 = In Range and Coerce(upper limit=9.0, x=w394, lower limit=1.0) -> (coerced(x)=w393:dbl, In Range?=w396:bool)
              n120 = Bundle By Name(cluster=w398, "PZT_Y"=w393) -> (w399:cluster{"PZT_X":dbl, "PZT_Y":dbl, "PZT_Z":dbl})
              n121 = Not(x=w396) -> (.not. x?=w391:bool)
              n122 = local write "PZTY_Limit"(w391) -> ()
            }
            event "PZT_Z+": Value Change {
              n123 = event-data() -> ()  [unwired: 1 in, 1 out]
              n124 = local read "PZTZ_Step"() -> (w405:dbl)
              n125 = Unbundle By Name(w411) -> ("PZT_Z"=w413:dbl)
              n126 = Divide(x=w405, y=3000.0) -> (x/y=w402:dbl)
              n127 = Subtract(x=w413, y=w402) -> (x-y=w408:dbl)
              n128 = In Range and Coerce(upper limit=9.0, x=w408, lower limit=1.0) -> (coerced(x)=w406:dbl, In Range?=w409:bool)
              n129 = Bundle By Name(cluster=w411, "PZT_Z"=w406) -> (w412:cluster{"PZT_X":dbl, "PZT_Y":dbl, "PZT_Z":dbl})
              n130 = Not(x=w409) -> (.not. x?=w404:bool)
              n131 = local write "PZTZ_Limit"(w404) -> ()
            }
            event "PZT_Z-": Value Change {
              n132 = event-data() -> ()  [unwired: 1 in, 1 out]
              n133 = local read "PZTZ_Step"() -> (w415:dbl)
              n134 = Unbundle By Name(w424) -> ("PZT_Z"=w426:dbl)
              n135 = Divide(x=w415, y=3000.0) -> (x/y=w416:dbl)
              n136 = Add(x=w426, y=w416) -> (x+y=w421:dbl)
              n137 = In Range and Coerce(upper limit=9.0, x=w421, lower limit=1.0) -> (coerced(x)=w419:dbl, In Range?=w422:bool)
              n138 = Bundle By Name(cluster=w424, "PZT_Z"=w419) -> (w425:cluster{"PZT_X":dbl, "PZT_Y":dbl, "PZT_Z":dbl})
              n139 = Not(x=w422) -> (.not. x?=w418:bool)
              n140 = local write "PZTZ_Limit"(w418) -> ()
            }
            event "PZT_Home": Value Change {
              w427 = 5.0 ("PZT_X")
              n141 = event-data() -> ()  [unwired: 1 in, 1 out]
              n142 = Bundle By Name(cluster=w430, "PZT_X"=w427, "PZT_Y"=w427, "PZT_Z"=w427) -> (w429:cluster{"PZT_X":dbl, "PZT_Y":dbl, "PZT_Z":dbl})
            }
            event Key Down {
              n143 = event-data() -> ("ScanCode"=w432:i16, "VKey"=w435:T1)  [unwired: 1 in]
              n144 = case shown="Default" w435 {
                tunnel: w434 -> [w438 w454 w470 w486 w502 w518 w533 w537 w543]
                tunnel: [w437 w453 w469 w485 w501 w517 w533 w537 w543] -> w433
                tunnel: w432 -> [w436 w452 w468 w484 w500 w516 w532 w536 _]
                frame "Right" {
                  # "X+"
                  n145 = case shown="77" w436 {
                    tunnel: w438 -> [w439 w450]
                    tunnel: [w439 w449] -> w437
                    frame 0, Default {
                    }
                    frame 77 {
                      n146 = local read "PZTX_Step"() -> (w443:dbl)
                      n147 = Unbundle By Name(w450) -> ("PZT_X"=w451:dbl)
                      n148 = Divide(x=w443, y=5000.0) -> (x/y=w441:dbl)
                      n149 = Subtract(x=w451, y=w441) -> (x-y=w445:dbl)
                      n150 = In Range and Coerce(upper limit=9.0, x=w445, lower limit=1.0) -> (coerced(x)=w444:dbl, In Range?=w447:bool)
                      n151 = Bundle By Name(cluster=w450, "PZT_X"=w444) -> (w449:cluster{"PZT_X":dbl, "PZT_Y":dbl, "PZT_Z":dbl})
                      n152 = Not(x=w447) -> (.not. x?=w442:bool)
                      n153 = local write "PZTX_Limit"(w442) -> ()
                    }
                  }
                }
                frame "Left" {
                  # "X-"
                  n154 = case shown="75" w452 {
                    tunnel: w454 -> [w455 w466]
                    tunnel: [w455 w465] -> w453
                    frame 0, Default {
                    }
                    frame 75 {
                      n155 = local read "PZTX_Step"() -> (w459:dbl)
                      n156 = Unbundle By Name(w466) -> ("PZT_X"=w467:dbl)
                      n157 = Divide(x=w459, y=5000.0) -> (x/y=w457:dbl)
                      n158 = Add(x=w467, y=w457) -> (x+y=w461:dbl)
                      n159 = In Range and Coerce(upper limit=9.0, x=w461, lower limit=ext 1.0) -> (coerced(x)=w460:ext, In Range?=w463:bool)
                      n160 = Bundle By Name(cluster=w466, "PZT_X"=w460) -> (w465:cluster{"PZT_X":dbl, "PZT_Y":dbl, "PZT_Z":dbl})
                      n161 = Not(x=w463) -> (.not. x?=w458:bool)
                      n162 = local write "PZTX_Limit"(w458) -> ()
                    }
                  }
                }
                frame "Up" {
                  # "Y+"
                  n163 = case shown="72" w468 {
                    tunnel: w470 -> [w471 w482]
                    tunnel: [w471 w481] -> w469
                    frame 0, Default {
                    }
                    frame 72 {
                      n164 = local read "PZTY_Step"() -> (w475:dbl)
                      n165 = Unbundle By Name(w482) -> ("PZT_Y"=w483:dbl)
                      n166 = Divide(x=w475, y=5000.0) -> (x/y=w473:dbl)
                      n167 = Add(x=w483, y=w473) -> (x+y=w478:dbl)
                      n168 = In Range and Coerce(upper limit=9.0, x=w478, lower limit=1.0) -> (coerced(x)=w476:dbl, In Range?=w479:bool)
                      n169 = Bundle By Name(cluster=w482, "PZT_Y"=w476) -> (w481:cluster{"PZT_X":dbl, "PZT_Y":dbl, "PZT_Z":dbl})
                      n170 = Not(x=w479) -> (.not. x?=w474:bool)
                      n171 = local write "PZTY_Limit"(w474) -> ()
                    }
                  }
                }
                frame "Down" {
                  # "Y-"
                  n172 = case shown="80" w484 {
                    tunnel: w486 -> [w487 w498]
                    tunnel: [w487 w497] -> w485
                    frame 0, Default {
                    }
                    frame 80 {
                      n173 = local read "PZTY_Step"() -> (w491:dbl)
                      n174 = Unbundle By Name(w498) -> ("PZT_Y"=w499:dbl)
                      n175 = Divide(x=w491, y=5000.0) -> (x/y=w489:dbl)
                      n176 = Subtract(x=w499, y=w489) -> (x-y=w493:dbl)
                      n177 = In Range and Coerce(upper limit=9.0, x=w493, lower limit=1.0) -> (coerced(x)=w492:dbl, In Range?=w495:bool)
                      n178 = Bundle By Name(cluster=w498, "PZT_Y"=w492) -> (w497:cluster{"PZT_X":dbl, "PZT_Y":dbl, "PZT_Z":dbl})
                      n179 = Not(x=w495) -> (.not. x?=w490:bool)
                      n180 = local write "PZTY_Limit"(w490) -> ()
                    }
                  }
                }
                frame "PageUp" {
                  # "Z+"
                  n181 = case shown="73" w500 {
                    tunnel: w502 -> [w503 w514]
                    tunnel: [w503 w513] -> w501
                    frame 0, Default {
                    }
                    frame 73 {
                      n182 = local read "PZTZ_Step"() -> (w507:dbl)
                      n183 = Unbundle By Name(w514) -> ("PZT_Z"=w515:dbl)
                      n184 = Divide(x=w507, y=3000.0) -> (x/y=w505:dbl)
                      n185 = Subtract(x=w515, y=w505) -> (x-y=w509:dbl)
                      n186 = In Range and Coerce(upper limit=9.0, x=w509, lower limit=1.0) -> (coerced(x)=w508:dbl, In Range?=w511:bool)
                      n187 = Bundle By Name(cluster=w514, "PZT_Z"=w508) -> (w513:cluster{"PZT_X":dbl, "PZT_Y":dbl, "PZT_Z":dbl})
                      n188 = Not(x=w511) -> (.not. x?=w506:bool)
                      n189 = local write "PZTZ_Limit"(w506) -> ()
                    }
                  }
                }
                frame "PageDown" {
                  # "Z-"
                  n190 = case shown="81" w516 {
                    tunnel: w518 -> [w519 w530]
                    tunnel: [w519 w529] -> w517
                    frame 0, Default {
                    }
                    frame 81 {
                      n191 = local read "PZTZ_Step"() -> (w523:dbl)
                      n192 = Unbundle By Name(w530) -> ("PZT_Z"=w531:dbl)
                      n193 = Divide(x=w523, y=3000.0) -> (x/y=w521:dbl)
                      n194 = Add(x=w531, y=w521) -> (x+y=w525:dbl)
                      n195 = In Range and Coerce(upper limit=9.0, x=w525, lower limit=1.0) -> (coerced(x)=w524:dbl, In Range?=w527:bool)
                      n196 = Bundle By Name(cluster=w530, "PZT_Z"=w524) -> (w529:cluster{"PZT_X":dbl, "PZT_Y":dbl, "PZT_Z":dbl})
                      n197 = Not(x=w527) -> (.not. x?=w522:bool)
                      n198 = local write "PZTZ_Limit"(w522) -> ()
                    }
                  }
                }
                frame "Delete" {
                  # "Step size switch"
                  n199 = case shown="83" w532 {
                    frame 0, Default {
                    }
                    frame 83 {
                      n200 = local read "PZT_Step_Select"() -> (w535:bool)
                      n201 = Not(x=w535) -> (.not. x?=w534:bool)
                      n202 = local write "PZT_Step_Select"(w534) -> ()
                    }
                  }
                }
                frame "Shift" {
                  # "Switch btw manual - oscillation"
                  n203 = case shown="54" w536 {
                    frame 0, Default {
                    }
                    frame 54 {
                      n204 = local read "PZT_Manual_ON"() -> (w538:bool)
                      n205 = case shown="True" w538 {
                        frame True {
                          n206 = local write "PZT_oscillation_Run"(TRUE ("PZT_oscillation")) -> ()
                          n207 = local write "PZT_Manual_ON"(FALSE ("PZT_manual")) -> ()
                        }
                        frame False {
                          n208 = local write "PZT_oscillation_Run"(FALSE ("PZT_oscillation")) -> ()
                          n209 = local write "PZT_Manual_ON"(TRUE ("PZT_manual")) -> ()
                        }
                      }
                    }
                  }
                }
                frame Default {
                }
              }
            }
            event Key Repeat {
              n210 = event-data() -> ("ScanCode"=w545:i16, "VKey"=w551:T1)  [unwired: 1 in]
              n211 = Divide(x=1000.0, y="PZT_Speed") -> (x/y=w546:dbl)
              n212 = Wait (ms)(milliseconds to wait=w546) -> ()  [unwired: 1 out]
              n213 = case shown="\"Right\"" w551 {
                tunnel: w550 -> [w552 w555 w571 w587 w603 w619 w635]
                tunnel: [w552 w554 w570 w586 w602 w618 w634] -> w549
                tunnel: w545 -> [_ w553 w569 w585 w601 w617 w633]
                frame Default {
                }
                frame "Right" {
                  n214 = case shown="77" w553 {
                    tunnel: w555 -> [w556 w567]
                    tunnel: [w556 w566] -> w554
                    frame 0, Default {
                    }
                    frame 77 {
                      n215 = local read "PZTX_Step"() -> (w559:dbl)
                      n216 = Unbundle By Name(w567) -> ("PZT_X"=w568:dbl)
                      n217 = Divide(x=w559, y=5000.0) -> (x/y=w558:dbl)
                      n218 = Subtract(x=w568, y=w558) -> (x-y=w565:dbl)
                      n219 = In Range and Coerce(upper limit=9.0, x=w565, lower limit=1.0) -> (coerced(x)=w562:dbl, In Range?=w561:bool)
                      n220 = Bundle By Name(cluster=w567, "PZT_X"=w562) -> (w566:cluster{"PZT_X":dbl, "PZT_Y":dbl, "PZT_Z":dbl})
                      n221 = Not(x=w561) -> (.not. x?=w560:bool)
                      n222 = local write "PZTX_Limit"(w560) -> ()
                    }
                  }
                }
                frame "Left" {
                  n223 = case shown="75" w569 {
                    tunnel: w571 -> [w572 w583]
                    tunnel: [w572 w582] -> w570
                    frame 0, Default {
                    }
                    frame 75 {
                      n224 = local read "PZTX_Step"() -> (w575:dbl)
                      n225 = Unbundle By Name(w583) -> ("PZT_X"=w584:dbl)
                      n226 = Divide(x=w575, y=5000.0) -> (x/y=w574:dbl)
                      n227 = Add(x=w584, y=w574) -> (x+y=w581:dbl)
                      n228 = In Range and Coerce(upper limit=9.0, x=w581, lower limit=1.0) -> (coerced(x)=w578:dbl, In Range?=w577:bool)
                      n229 = Bundle By Name(cluster=w583, "PZT_X"=w578) -> (w582:cluster{"PZT_X":dbl, "PZT_Y":dbl, "PZT_Z":dbl})
                      n230 = Not(x=w577) -> (.not. x?=→"PZTX_Limit":bool)
                    }
                  }
                }
                frame "Up" {
                  n231 = case shown="72" w585 {
                    tunnel: w587 -> [w588 w599]
                    tunnel: [w588 w598] -> w586
                    frame 0, Default {
                    }
                    frame 72 {
                      n232 = local read "PZTY_Step"() -> (w591:dbl)
                      n233 = Unbundle By Name(w599) -> ("PZT_Y"=w600:dbl)
                      n234 = Divide(x=w591, y=5000.0) -> (x/y=w590:dbl)
                      n235 = Add(x=w600, y=w590) -> (x+y=w597:dbl)
                      n236 = In Range and Coerce(upper limit=9.0, x=w597, lower limit=1.0) -> (coerced(x)=w596:dbl, In Range?=w593:bool)
                      n237 = Bundle By Name(cluster=w599, "PZT_Y"=w596) -> (w598:cluster{"PZT_X":dbl, "PZT_Y":dbl, "PZT_Z":dbl})
                      n238 = Not(x=w593) -> (.not. x?=→"PZTY_Limit":bool)
                    }
                  }
                }
                frame "Down" {
                  n239 = case shown="80" w601 {
                    tunnel: w603 -> [w604 w615]
                    tunnel: [w604 w614] -> w602
                    frame 0, Default {
                    }
                    frame 80 {
                      n240 = local read "PZTY_Step"() -> (w607:dbl)
                      n241 = Unbundle By Name(w615) -> ("PZT_Y"=w616:dbl)
                      n242 = Divide(x=w607, y=5000.0) -> (x/y=w606:dbl)
                      n243 = Subtract(x=w616, y=w606) -> (x-y=w613:dbl)
                      n244 = In Range and Coerce(upper limit=9.0, x=w613, lower limit=1.0) -> (coerced(x)=w610:dbl, In Range?=w609:bool)
                      n245 = Bundle By Name(cluster=w615, "PZT_Y"=w610) -> (w614:cluster{"PZT_X":dbl, "PZT_Y":dbl, "PZT_Z":dbl})
                      n246 = Not(x=w609) -> (.not. x?=w608:bool)
                      n247 = local write "PZTY_Limit"(w608) -> ()
                    }
                  }
                }
                frame "PageUp" {
                  n248 = case shown="73" w617 {
                    tunnel: w619 -> [w620 w631]
                    tunnel: [w620 w630] -> w618
                    frame 0, Default {
                    }
                    frame 73 {
                      n249 = local read "PZTZ_Step"() -> (w623:dbl)
                      n250 = Unbundle By Name(w631) -> ("PZT_Z"=w632:dbl)
                      n251 = Divide(x=w623, y=3000.0) -> (x/y=w622:dbl)
                      n252 = Subtract(x=w632, y=w622) -> (x-y=w629:dbl)
                      n253 = In Range and Coerce(upper limit=9.0, x=w629, lower limit=1.0) -> (coerced(x)=w626:dbl, In Range?=w625:bool)
                      n254 = Bundle By Name(cluster=w631, "PZT_Z"=w626) -> (w630:cluster{"PZT_X":dbl, "PZT_Y":dbl, "PZT_Z":dbl})
                      n255 = Not(x=w625) -> (.not. x?=→"PZTZ_Limit":bool)
                    }
                  }
                }
                frame "PageDown" {
                  n256 = case shown="81" w633 {
                    tunnel: w635 -> [w636 w647]
                    tunnel: [w636 w646] -> w634
                    frame 0, Default {
                    }
                    frame 81 {
                      n257 = local read "PZTZ_Step"() -> (w639:dbl)
                      n258 = Unbundle By Name(w647) -> ("PZT_Z"=w648:dbl)
                      n259 = Divide(x=w639, y=3000.0) -> (x/y=w638:dbl)
                      n260 = Add(x=w648, y=w638) -> (x+y=w645:dbl)
                      n261 = In Range and Coerce(upper limit=9.0, x=w645, lower limit=1.0) -> (coerced(x)=w642:dbl, In Range?=w641:bool)
                      n262 = Bundle By Name(cluster=w647, "PZT_Z"=w642) -> (w646:cluster{"PZT_X":dbl, "PZT_Y":dbl, "PZT_Z":dbl})
                      n263 = Not(x=w641) -> (.not. x?=w640:bool)
                      n264 = local write "PZTZ_Limit"(w640) -> ()
                    }
                  }
                }
              }
            }
            event "PZT_oscillation_Run": Value Change {
              n265 = event-data() -> ()  [unwired: 1 in, 1 out]
              n266 = local read "PZT_Manual_ON"() -> (w651:bool)
              n267 = case shown="False" w651 {
                frame True {
                  n268 = local write "PZT_oscillation_Run"(TRUE ("PZT_oscillation")) -> ()
                  n269 = local write "PZT_Manual_ON"(FALSE ("PZT_manual")) -> ()
                }
                frame False {
                  n270 = local write "PZT_oscillation_Run"(FALSE ("PZT_oscillation")) -> ()
                  n271 = local write "PZT_Manual_ON"(TRUE ("PZT_manual")) -> ()
                }
              }
            }
            event Panel Close {
              n272 = event-data() -> ()  [unwired: 1 in, 1 out]
              n273 = Unbundle By Name(w657) -> ("PZT_X"=w661:dbl, "PZT_Y"=w660:dbl, "PZT_Z"=w659:dbl)
              n274 = Build Array(w661, w660, w659) -> (w658:dbl[])
              n275 = call "Convert to Dynamic Data2"("Array"=w658) -> ("Dynamic Data Type"=w662:dynamicdata)  [unwired: 3 in]
              n276 = call "Write To Measurement File2"("Signals"=w662) -> ()  [unwired: 16 in, 3 out]
            }
            event Application Instance Close {
              n277 = event-data() -> ()  [unwired: 1 in, 1 out]
              n278 = Unbundle By Name(w664) -> ("PZT_X"=w668:dbl, "PZT_Y"=w667:dbl, "PZT_Z"=w666:dbl)
              n279 = Build Array(w668, w667, w666) -> (w665:dbl[])
              n280 = call "Convert to Dynamic Data3"("Array"=w665) -> ("Dynamic Data Type"=w669:dynamicdata)  [unwired: 3 in]
              n281 = call "Write To Measurement File3"("Signals"=w669) -> ()  [unwired: 16 in, 3 out]
            }
            event "PZT_Zero": Value Change {
              w670 = 0.0 ("PZT_X")
              n282 = event-data() -> ()  [unwired: 1 in, 1 out]
              n283 = Bundle By Name(cluster=w672, "PZT_X"=w670, "PZT_Y"=w670, "PZT_Z"=w670) -> (w671:cluster{"PZT_X":dbl, "PZT_Y":dbl, "PZT_Z":dbl})
            }
          }
          n284 = Unbundle By Name(w258) -> ("PZT_X"=w246:dbl, "PZT_Y"=w245:dbl, "PZT_Z"=w243:dbl)
          n285 = local read "PZT_oscillation_Run"() -> (w250:bool)
          n286 = case shown="True" "PZT_Step_Select" {
            frame False {
              n287 = stacked-sequence {
                frame #0 {
                  n288 = local write "PZTX_Step"("PZTX_Step1") -> ()
                }
                frame #1 {
                  n289 = local write "PZTY_Step"("PZTY_Step1") -> ()
                }
                frame #2 {
                  n290 = local write "PZTZ_Step"("PZTZ_Step1") -> ()
                }
              }
            }
            frame True {
              n291 = stacked-sequence {
                frame #0 {
                  "PZTX_Step" <- "PZTX_Step2"
                }
                frame #1 {
                  "PZTY_Step" <- "PZTY_Step2"
                }
                frame #2 {
                  "PZTZ_Step" <- "PZTZ_Step2"
                }
              }
            }
          }
          n292 = Subtract(x=w246, y=w242) -> (x-y=w238:dbl)
          n293 = Subtract(x=w245, y=w242) -> (x-y=w237:dbl)
          n294 = Subtract(x=w243, y=w242) -> (x-y=w244:dbl)
          n295 = Multiply(x=w238, y=w236) -> (x*y=→"PZTX_Position":dbl)
          n296 = Multiply(x=w236, y=w237) -> (x*y=→"PZTY_Position":dbl)
          n297 = Multiply(x=w244, y=3000.0) -> (x*y=w239:dbl)
          n298 = Negate(x=w239) -> (-x=→"PZTZ_Position":dbl)
          n299 = case shown="True" w250 {
            tunnel: [w262 w285] -> w253
            tunnel: w246 -> [w266 w281]
            tunnel: w245 -> [w265 w280]
            tunnel: w243 -> [w264 w279]
            tunnel: w247 -> [w261 _]
            frame False {
              # "Manual mode"
              n300 = Build Array(w266, w265, w264) -> (w263:dbl[])
              n301 = case shown="True" w261 {
                tunnel: w263 -> [_ w271]
                tunnel: [errorcluster {"status"=FALSE, "code"=0, "source"=""} ("error out") w268] -> w262
                frame False {
                }
                frame True {
                  n302 = call-poly <vilib>:"DAQmx Create Virtual Channel.vi"("maximum value"=10.0, "minimum value"=0.0, "physical channels"=tag "DAQ/ao0:2") -> ("task out"=w275:refnum<k21>, "error out"=w274:errorcluster)  [unwired: 11 in]
                  n303 = call <vilib>:"DAQmx Start Task.vi"("task/channels in"=w275, "error in"=w274) -> ("task out"=w273:refnum<k21>, "error out"=w272:errorcluster)  [unwired: 12 in]
                  n304 = call-poly <vilib>:"DAQmx Write.vi"("task/channels in"=w273, "data"=w271, "error in"=w272) -> ("task out"=w270:refnum<k21>, "error out"=w269:errorcluster)  [unwired: 10 in, 1 out]
                  n305 = call <vilib>:"DAQmx Clear Task.vi"("task in"=w270, "error in"=w269) -> ("error out"=w268:errorcluster)  [unwired: 13 in]
                }
              }
            }
            frame True {
              # "Oscillation mode"
              n306 = case shown="\"X\", Default" "PZT_Axis" {
                tunnel: [w292 w306 w328] -> w285
                tunnel: "PZT_Waveform" -> [_ _ _]
                tunnel: "PZT_Frequency" -> [w291 w310 w327]
                tunnel: "PZT_Amplitude" -> [w290 w307 w325]
                tunnel: w281 -> [w287 _ _]
                tunnel: w280 -> [_ w305 _]
                tunnel: w279 -> [_ _ w323]
                frame "X", Default {
                  n307 = Divide(x=w290, y=5000.0) -> (x/y=w289:dbl)
                  n308 = call "PZT_SignalGenerator.vi"("Physical Channels"=tag "DAQ/ao0", "Offset"=w287, "Frequency"=w291, "Amplitude"=w289) -> ("error out"=w292:errorcluster)  [unwired: 3 in, 1 out]
                  n309 = while {
                    i -> [w297]
                    stop <- w296 stop-if-true
                    n310 = local read "PZT_oscillation_Run"() -> (w295:bool)
                    n311 = global write "PZT_oscillation.vi" "PZT_oscillation"(w295) -> ()
                    n312 = event shown="[1] Key Down" {
                      selector: _ -> [_ _]
                      dyn-events: _ -> [_ _]
                      timeout: 10 -> [_ _]
                      event Timeout {
                        n313 = event-data() -> ()  [unwired: 1 in, 1 out]
                      }
                      event Key Down {
                        n314 = event-data() -> ("VKey"=w304:T1)  [unwired: 1 in]
                        n315 = local read "PZT_Os_Num"() -> (w300:i32)
                        n316 = Equal?(x=w304, y=eventvkey."Shift") -> (x = y?=w302:bool)
                        n317 = Greater Than 0?(x=w300) -> (x > 0?=w301:bool)
                        n318 = Not And(1:w301, 2:w302) -> (0:w299:bool)
                        n319 = local write "PZT_oscillation_Run"(w299) -> ()
                      }
                    }
                    n320 = Not(x=w295) -> (.not. x?=w296:bool)
                    n321 = Wait (ms)(milliseconds to wait=u32 10) -> ()  [unwired: 1 out]
                    "PZT_Os_Num" <- w297
                  }
                }
                frame "Y" {
                  n322 = Divide(x=w307, y=5000.0) -> (x/y=w308:dbl)
                  n323 = call "PZT_SignalGenerator.vi"("Physical Channels"=tag "DAQ/ao1", "Offset"=w305, "Frequency"=w310, "Amplitude"=w308) -> ("error out"=w306:errorcluster)  [unwired: 3 in, 1 out]
                  n324 = while {
                    i -> [w315]
                    stop <- w314 stop-if-true
                    n325 = local read "PZT_oscillation_Run"() -> (w313:bool)
                    n326 = global write "PZT_oscillation.vi" "PZT_oscillation"(w313) -> ()
                    n327 = event shown="[1] Key Down" {
                      selector: _ -> [_ _]
                      dyn-events: _ -> [_ _]
                      timeout: 10 -> [_ _]
                      event Timeout {
                        n328 = event-data() -> ()  [unwired: 1 in, 1 out]
                      }
                      event Key Down {
                        n329 = event-data() -> ("VKey"=w322:T1)  [unwired: 1 in]
                        n330 = local read "PZT_Os_Num"() -> (w318:i32)
                        n331 = Equal?(x=w322, y=eventvkey."Shift") -> (x = y?=w320:bool)
                        n332 = Greater Than 0?(x=w318) -> (x > 0?=w319:bool)
                        n333 = Not And(1:w319, 2:w320) -> (0:w317:bool)
                        n334 = local write "PZT_oscillation_Run"(w317) -> ()
                      }
                    }
                    n335 = Not(x=w313) -> (.not. x?=w314:bool)
                    n336 = local write "PZT_Os_Num"(w315) -> ()
                    n337 = Wait (ms)(milliseconds to wait=u32 10) -> ()  [unwired: 1 out]
                  }
                }
                frame "Z" {
                  n338 = Divide(x=w325, y=3000.0) -> (x/y=w324:dbl)
                  n339 = call "PZT_SignalGenerator.vi"("Physical Channels"=tag "DAQ/ao2", "Offset"=w323, "Frequency"=w327, "Amplitude"=w324) -> ("error out"=w328:errorcluster)  [unwired: 3 in, 1 out]
                  n340 = while {
                    i -> [w330]
                    stop <- w333 stop-if-true
                    n341 = local read "PZT_oscillation_Run"() -> (w332:bool)
                    n342 = global write "PZT_oscillation.vi" "PZT_oscillation"(w332) -> ()
                    n343 = event shown="[1] Key Down" {
                      selector: _ -> [_ _]
                      dyn-events: _ -> [_ _]
                      timeout: 10 -> [_ _]
                      event Timeout {
                        n344 = event-data() -> ()  [unwired: 1 in, 1 out]
                      }
                      event Key Down {
                        n345 = event-data() -> ("VKey"=w340:T1)  [unwired: 1 in]
                        n346 = local read "PZT_Os_Num"() -> (w336:i32)
                        n347 = Equal?(x=w340, y=eventvkey."Shift") -> (x = y?=w338:bool)
                        n348 = Greater Than 0?(x=w336) -> (x > 0?=w337:bool)
                        n349 = Not And(1:w337, 2:w338) -> (0:w335:bool)
                        n350 = local write "PZT_oscillation_Run"(w335) -> ()
                      }
                    }
                    n351 = Not(x=w332) -> (.not. x?=w333:bool)
                    n352 = local write "PZT_Os_Num"(w330) -> ()
                    n353 = Wait (ms)(milliseconds to wait=u32 10) -> ()  [unwired: 1 out]
                  }
                }
              }
            }
          }
          n354 = Merge Errors(w253, w248) -> (w252:errorcluster)
          n355 = Or(x="PZT_STOP", y=w252) -> (x .or. y?=w256:bool)
          n356 = Not(x=w256) -> (.not. x?=→"PZT_ON":bool)
          n357 = Wait (ms)(milliseconds to wait=u32 1) -> ()  [unwired: 1 out]
          "PZT_Man_Num" <- w254
        }
      }
    }
    n358 = Or(x="STOP", y=w221) -> (x .or. y?=w224:bool)
    n359 = Wait (ms)(milliseconds to wait=u32 100) -> ()  [unwired: 1 out]
    "PZT_Manual_ON" <- "PZT_START"
  }
  n360 = while {
    shift-right: [w674] -> w41
    shift-left: w2 -> [w675]
    stop <- w676 stop-if-true
    # "FluorescenceLaser-Power"
    n361 = case shown="True" "OK Button 6" {
      tunnel: [errorcluster {"status"=FALSE, "code"=0, "source"=""} ("error out") w681] -> w674
      tunnel: w675 -> [_ w683]
      frame False {
      }
      frame True {
        w688 = 0 items=["one channel for each line", "one channel for all lines"] ("line grouping")
        n362 = call-poly <vilib>:"DAQmx Create Virtual Channel.vi"("lines"=tag "DAQ/port0/line0:2", "line grouping"=w688) -> ("task out"=w691:refnum<k21>, "error out"=w690:errorcluster)  [unwired: 12 in]
        n363 = call <vilib>:"DAQmx Start Task.vi"("task/channels in"=w691, "error in"=w690) -> ("task out"=w687:refnum<k21>, "error out"=w686:errorcluster)  [unwired: 12 in]
        n364 = while "Event Handle Loop" {
          shift-right: [w693] -> w685
          shift-left: w687 -> [w695]
          shift-right: [w692] -> w684
          shift-left: w686 -> [w694]
          i -> [w703]
          stop <- w700 stop-if-true
          # "Fluorescence Laser"
          n365 = Build Array("Flu_Blue_Run", "Flu_Green_Run", "Flu_Red_Run") -> (w696:bool[])
          n366 = call-poly <vilib>:"DAQmx Write.vi"("task/channels in"=w695, "data"=w696, "error in"=w694) -> ("task out"=w693:refnum<k21>, "error out"=w692:errorcluster)  [unwired: 10 in, 1 out]
          n367 = Or(x=w692, y="stop 6") -> (x .or. y?=w700:bool)
          n368 = Wait (ms)(milliseconds to wait=u32 100) -> ()  [unwired: 1 out]
          "Numeric 9" <- w703
        }
        n369 = call <vilib>:"DAQmx Clear Task.vi"("task in"=w685, "error in"=w684) -> ("error out"=w682:errorcluster)  [unwired: 13 in]
        n370 = Merge Errors(w682, w683) -> (w681:errorcluster)
      }
    }
    n371 = local read "STOP"() -> (w677:bool)
    n372 = Wait (ms)(milliseconds to wait=u32 100) -> ()  [unwired: 1 out]
    n373 = Or(x=w677, y=w674) -> (x .or. y?=w676:bool)
    "FluorescenceLaser_ON" <- "OK Button 6"
  }
  n374 = while {
    shift-right: [w705] -> w42
    shift-left: w2 -> [w704]
    stop <- w707 stop-if-true
    # "StageX"
    n375 = case shown="True" "StageX_Start" {
      tunnel: [w710 w715] -> w705
      tunnel: w704 -> [w710 w711]
      frame False {
      }
      frame True {
        # "StageXYZ\nKey   Scan  Char\n(X+, 6)  77      54\n(X-,  4)  75      52\n(Y-,  2)  72      56\n(Y+, 8)  80      50\n(Z+, -)  74       45\n(Z-, +)  78       43\n(Vel, 5) 76       53"
        n376 = call <userlib>:"Connect Newport Instrument1.vi"("error in (no error)"=w711, "Controller address"=1, "Selected device"="ASRL7  (COM7 - USB Serial Port)" ("String")) -> ("error (duplicate)"=w712:errorcluster, "Connected"=w718:bool, "Device Connection Cluster"=w719:T3)  [unwired: 4 in, 2 out]
        n377 = case shown="True" w718 {
          tunnel: w719 -> [w722 w726]
          tunnel: [w722 w728] -> w717
          tunnel: [w720 w727] -> w715
          tunnel: w712 -> [w721 w723]
          frame False {
            n378 = call <vilib>:"Simple Error Handler.vi"("error in (no error)"=w721) -> ("error out"=w720:errorcluster)  [unwired: 4 in, 4 out]
          }
          frame True {
            # "x = [0-5]\nv = [0.1-2]"
            n379 = call <userlib>:"CONEX-CC Set Negative Software Limit v2.vi"("Negative limit (left)"=0.0, "Connection Cluster in"=w726) -> ("Connection Cluster out"=w732:T3)  [unwired: 9 in]
            n380 = call <userlib>:"CONEX-CC Set Positive Software Limit v2.vi"("Positive limit (right)"=5.0, "Connection Cluster in"=w732) -> ("Connection Cluster out"=w731:T3)  [unwired: 9 in]
            n381 = call <userlib>:"CONEX-CC Set Velocity v2.vi"("Velocity"=2.0, "Connection Cluster in"=w731) -> ("Connection Cluster out"=w725:T3)  [unwired: 9 in]
            n382 = while {
              shift-right: [w739] -> w727
              shift-left: w723 -> [w742]
              shift-right: [w736] -> w728
              shift-left: w725 -> [w738]
              i -> [w745]
              stop <- w743 stop-if-true
              n383 = event shown="[5] \"StageX_Home\": Value Change" {
                selector: _ -> [_ _ _ _ _ _]
                dyn-events: _ -> [_ _ _ _ _ _]
                timeout: 1 -> [_ _ _ _ _ _]
                tunnel: w738 -> [w762 w764 w775 w783 w821 w855]
                tunnel: [w762 w768 w772 w782 w820 w848] -> w737
                tunnel: [FALSE TRUE TRUE w776 w814 TRUE] -> w733
                event Timeout {
                  n384 = event-data() -> ()  [unwired: 1 in, 1 out]
                }
                event "StageX+": Value Change {
                  n385 = event-data() -> ()  [unwired: 1 in, 1 out]
                  n386 = local read "StageX_Step"() -> (w765:dbl)
                  n387 = Divide(x=w765, y=1000.0) -> (x/y=w767:dbl)
                  n388 = call <userlib>:"CONEX-CC Relative Move v2.vi"("Relative displacement"=w767, "Connection Cluster in"=w764) -> ("Connection Cluster out"=w768:T3)  [unwired: 9 in]
                }
                event "StageX-": Value Change {
                  n389 = event-data() -> ()  [unwired: 1 in, 1 out]
                  n390 = local read "StageX_Step"() -> (w774:dbl)
                  n391 = Negate(x=w774) -> (-x=w773:dbl)
                  n392 = Divide(x=w773, y=1000.0) -> (x/y=w771:dbl)
                  n393 = call <userlib>:"CONEX-CC Relative Move v2.vi"("Relative displacement"=w771, "Connection Cluster in"=w775) -> ("Connection Cluster out"=w772:T3)  [unwired: 9 in]
                }
                event Key Down {
                  n394 = event-data() -> ("Char"=w778:i16, "ScanCode"=w777:i16)  [unwired: 1 in]
                  n395 = local read "StageX_Step"() -> (w780:dbl)
                  n396 = Divide(x=w780, y=1000.0) -> (x/y=w779:dbl)
                  n397 = case shown="0, Default" w778 {
                    tunnel: w783 -> [w785 w790 w802 w811]
                    tunnel: [w785 w789 w801 w811] -> w782
                    tunnel: w779 -> [_ w788 w800 _]
                    tunnel: w777 -> [_ w787 w799 w810]
                    tunnel: [FALSE w786 w798 FALSE] -> w776
                    frame 0, Default {
                    }
                    frame 52 {
                      n398 = case shown="75" w787 {
                        tunnel: w790 -> [w792 w797]
                        tunnel: [w792 w796] -> w789
                        tunnel: w788 -> [_ w795]
                        tunnel: [FALSE TRUE] -> w786
                        frame 0, Default {
                        }
                        frame 75 {
                          n399 = Negate(x=w795) -> (-x=w794:dbl)
                          n400 = call <userlib>:"CONEX-CC Relative Move v2.vi"("Relative displacement"=w794, "Connection Cluster in"=w797) -> ("Connection Cluster out"=w796:T3)  [unwired: 9 in]
                        }
                      }
                    }
                    frame 54 {
                      n401 = case shown="77" w799 {
                        tunnel: w802 -> [w804 w808]
                        tunnel: [w804 w807] -> w801
                        tunnel: w800 -> [_ w806]
                        tunnel: [FALSE TRUE] -> w798
                        frame 0, Default {
                        }
                        frame 77 {
                          n402 = call <userlib>:"CONEX-CC Relative Move v2.vi"("Relative displacement"=w806, "Connection Cluster in"=w808) -> ("Connection Cluster out"=w807:T3)  [unwired: 9 in]
                        }
                      }
                    }
                    frame 53 {
                      n403 = case shown="76" w810 {
                        frame 0, Default {
                        }
                        frame 76 {
                          n404 = local read "Stage_Step_Select"() -> (w812:bool)
                          n405 = Not(x=w812) -> (.not. x?=w813:bool)
                          n406 = local write "Stage_Step_Select"(w813) -> ()
                        }
                      }
                    }
                  }
                }
                event Key Repeat {
                  n407 = event-data() -> ("Char"=w819:i16, "ScanCode"=w815:i16)  [unwired: 1 in]
                  n408 = local read "StageX_Step"() -> (w817:dbl)
                  n409 = Divide(x=w817, y=1000.0) -> (x/y=w816:dbl)
                  n410 = case shown="0, Default" w819 {
                    tunnel: w821 -> [w823 w828 w840]
                    tunnel: [w823 w827 w839] -> w820
                    tunnel: w816 -> [_ w826 w838]
                    tunnel: w815 -> [_ w825 w837]
                    tunnel: [FALSE w824 w836] -> w814
                    frame 0, Default {
                    }
                    frame 52 {
                      n411 = case shown="75" w825 {
                        tunnel: w828 -> [w830 w835]
                        tunnel: [w830 w834] -> w827
                        tunnel: w826 -> [_ w833]
                        tunnel: [FALSE TRUE] -> w824
                        frame 0, Default {
                        }
                        frame 75 {
                          n412 = Negate(x=w833) -> (-x=w832:dbl)
                          n413 = call <userlib>:"CONEX-CC Relative Move v2.vi"("Relative displacement"=w832, "Connection Cluster in"=w835) -> ("Connection Cluster out"=w834:T3)  [unwired: 9 in]
                        }
                      }
                    }
                    frame 54 {
                      n414 = case shown="77" w837 {
                        tunnel: w840 -> [w842 w846]
                        tunnel: [w842 w845] -> w839
                        tunnel: w838 -> [_ w844]
                        tunnel: [FALSE TRUE] -> w836
                        frame 0, Default {
                        }
                        frame 77 {
                          n415 = call <userlib>:"CONEX-CC Relative Move v2.vi"("Relative displacement"=w844, "Connection Cluster in"=w846) -> ("Connection Cluster out"=w845:T3)  [unwired: 9 in]
                        }
                      }
                    }
                  }
                }
                event "StageX_Home": Value Change {
                  n416 = event-data() -> ()  [unwired: 1 in, 1 out]
                  n417 = call <userlib>:"CONEX-CC Set Velocity v2.vi"("Velocity"=0.1, "Connection Cluster in"=w855) -> ("Connection Cluster out"=w854:T3)  [unwired: 9 in]
                  n418 = call <userlib>:"CONEX-CC Absolute Move v2.vi"("Target position"=2.7, "Connection Cluster in"=w854) -> ("Connection Cluster out"=w851:T3)  [unwired: 5 in, 2 out]
                  n419 = while {
                    shift-right: [w856] -> w849
                    shift-left: w851 -> [w860]
                    stop <- w858 stop-if-true
                    n420 = flat-sequence {
                      tunnel: w860 -> [w868]
                      tunnel: [w867] -> w859
                      tunnel: [w866] -> w857
                      tunnel: w859 -> [w872]
                      tunnel: [w872] -> w858
                      tunnel: w857 -> [w871]
                      tunnel: [w871] -> w856
                      frame #0 {
                        n421 = call <userlib>:"CONEX-CC Get Current Position v2.vi"("Connection Cluster in"=w868) -> ("Current position"=w865:dbl, "Connection Cluster out"=w866:T3)  [unwired: 8 in, 1 out]
                        n422 = Subtract(x=w865, y=2.7) -> (x-y=w864:dbl)
                        n423 = Multiply(x=1000.0, y=w864) -> (x*y=w862:dbl)
                        n424 = local write "StageX_Position"(w862) -> ()
                        n425 = In Range and Coerce(upper limit=2.701 ("x"), x=w865, lower limit=2.699 ("x")) -> (In Range?=w867:bool)  [unwired: 1 out]
                      }
                      frame #1 {
                        n426 = Wait (ms)(milliseconds to wait=u32 1) -> ()  [unwired: 1 out]
                      }
                    }
                  }
                  n427 = call <userlib>:"CONEX-CC Set Velocity v2.vi"("Velocity"=2.0, "Connection Cluster in"=w849) -> ("Connection Cluster out"=w848:T3)  [unwired: 9 in]
                }
              }
              n428 = case shown="True" w733 {
                tunnel: w737 -> [w749 w751]
                tunnel: [w749 w750] -> w736
                frame False {
                }
                frame True {
                  w754 = 2000.0 ("upper limit")
                  n429 = Negate(x=w754) -> (-x=w759:dbl)
                  n430 = call <userlib>:"CONEX-CC Get Current Position v2.vi"("Connection Cluster in"=w751) -> ("Current position"=w755:dbl, "Connection Cluster out"=w750:T3)  [unwired: 8 in, 1 out]
                  n431 = Subtract(x=w755, y=2.7) -> (x-y=w756:dbl)
                  n432 = Multiply(x=w756, y=1000.0) -> (x*y=w758:dbl)
                  "StageX_Position" <- w758
                  n433 = In Range and Coerce(upper limit=w754, x=w758, lower limit=w759) -> (In Range?=w757:bool)  [unwired: 1 out]
                  n434 = Not(x=w757) -> (.not. x?=→"StageX_Limit":bool)
                }
              }
              n435 = Unbundle By Name(w736) -> ("error"=w741:errorcluster)
              n436 = Merge Errors(w741, w742) -> (w739:errorcluster)
              n437 = Wait (ms)(milliseconds to wait=u32 1) -> ()  [unwired: 1 out]
              n438 = case shown="True" "Stage_Step_Select" {
                frame False {
                  n439 = local write "StageX_Step"("StageX_Step1") -> ()
                }
                frame True {
                  "StageX_Step" <- "StageX_Step2"
                }
              }
              n440 = Or(x="StageX_Stop", y=w739) -> (x .or. y?=w743:bool)
              n441 = Not(x=w743) -> (.not. x?=→"StageX_ON":bool)
              "Numeric" <- w745
            }
          }
        }
        n442 = Unbundle By Name(w717) -> ("VISA resource name"=w716:refnum<visa-resource-name>)
        n443 = call <userlib>:"_Close Communications.vi"("Instrument Channel"=w716) -> ()  [unwired: 14 in, 1 out]
      }
    }
    n444 = local read "STOP"() -> (w706:bool)
    n445 = Or(x=w706, y=w705) -> (x .or. y?=w707:bool)
    n446 = Wait (ms)(milliseconds to wait=u32 100) -> ()  [unwired: 1 out]
  }
  n447 = while {
    shift-right: [w875] -> w40
    shift-left: w2 -> [w874]
    stop <- w877 stop-if-true
    # "StageY"
    n448 = case shown="True" "StageY_Start" {
      tunnel: [w880 w884] -> w875
      tunnel: w874 -> [w880 w881]
      frame False {
      }
      frame True {
        n449 = call <userlib>:"Connect Newport Instrument1.vi"("error in (no error)"=w881, "Controller address"=1, "Selected device"="ASRL3  (COM3 - USB Serial Port)" ("String")) -> ("error (duplicate)"=w882:errorcluster, "Connected"=w888:bool, "Device Connection Cluster"=w887:T3)  [unwired: 4 in, 2 out]
        n450 = case shown="True" w888 {
          tunnel: w887 -> [w892 w897]
          tunnel: [w892 w896] -> w885
          tunnel: [w890 w893] -> w884
          tunnel: w882 -> [w891 w894]
          frame False {
            n451 = call <vilib>:"Simple Error Handler.vi"("error in (no error)"=w891) -> ("error out"=w890:errorcluster)  [unwired: 4 in, 4 out]
          }
          frame True {
            n452 = call <userlib>:"CONEX-CC Set Negative Software Limit v2.vi"("Negative limit (left)"=0.0, "Connection Cluster in"=w897) -> ("Connection Cluster out"=w902:T3)  [unwired: 9 in]
            n453 = call <userlib>:"CONEX-CC Set Positive Software Limit v2.vi"("Positive limit (right)"=5.0, "Connection Cluster in"=w902) -> ("Connection Cluster out"=w901:T3)  [unwired: 9 in]
            n454 = call <userlib>:"CONEX-CC Set Velocity v2.vi"("Velocity"=2.0, "Connection Cluster in"=w901) -> ("Connection Cluster out"=w895:T3)  [unwired: 9 in]
            n455 = while "Event Handle Loop" {
              shift-right: [w909] -> w893
              shift-left: w894 -> [w911]
              shift-right: [w905] -> w896
              shift-left: w895 -> [w907]
              i -> [w915]
              stop <- w913 stop-if-true
              # "Stage-Y"
              n456 = event shown="[5] \"StageY_Home\": Value Change" {
                selector: _ -> [_ _ _ _ _ _]
                dyn-events: _ -> [_ _ _ _ _ _]
                timeout: 1 -> [_ _ _ _ _ _]
                tunnel: w907 -> [w932 w935 w945 w953 w986 w1020]
                tunnel: [w932 w939 w943 w952 w985 w1013] -> w904
                tunnel: [FALSE TRUE TRUE w946 w979 TRUE] -> w903
                event Timeout {
                  n457 = event-data() -> ()  [unwired: 1 in, 1 out]
                }
                event "StageY+": Value Change {
                  n458 = event-data() -> ()  [unwired: 1 in, 1 out]
                  n459 = local read "StageY_Step"() -> (w936:dbl)
                  n460 = Divide(x=w936, y=1000.0) -> (x/y=w938:dbl)
                  n461 = Negate(x=w938) -> (-x=w934:dbl)
                  n462 = call <userlib>:"CONEX-CC Relative Move v2.vi"("Relative displacement"=w934, "Connection Cluster in"=w935) -> ("Connection Cluster out"=w939:T3)  [unwired: 9 in]
                }
                event "StageY-": Value Change {
                  n463 = event-data() -> ()  [unwired: 1 in, 1 out]
                  n464 = local read "StageY_Step"() -> (w944:dbl)
                  n465 = Divide(x=w944, y=1000.0) -> (x/y=w942:dbl)
                  n466 = call <userlib>:"CONEX-CC Relative Move v2.vi"("Relative displacement"=w942, "Connection Cluster in"=w945) -> ("Connection Cluster out"=w943:T3)  [unwired: 9 in]
                }
                event Key Down {
                  n467 = event-data() -> ("Char"=w948:i16, "ScanCode"=w947:i16)  [unwired: 1 in]
                  n468 = local read "StageY_Step"() -> (w950:dbl)
                  n469 = Divide(x=w950, y=1000.0) -> (x/y=w949:dbl)
                  n470 = case shown="50" w948 {
                    tunnel: w953 -> [w955 w960 w971]
                    tunnel: [w955 w959 w970] -> w952
                    tunnel: w949 -> [_ w958 w969]
                    tunnel: w947 -> [_ w957 w968]
                    tunnel: [FALSE w956 w967] -> w946
                    frame 0, Default {
                    }
                    frame 50 {
                      n471 = case shown="80" w957 {
                        tunnel: w960 -> [w962 w966]
                        tunnel: [w962 w965] -> w959
                        tunnel: w958 -> [_ w964]
                        tunnel: [FALSE TRUE] -> w956
                        frame 0, Default {
                        }
                        frame 80 {
                          n472 = call <userlib>:"CONEX-CC Relative Move v2.vi"("Relative displacement"=w964, "Connection Cluster in"=w966) -> ("Connection Cluster out"=w965:T3)  [unwired: 9 in]
                        }
                      }
                    }
                    frame 56 {
                      n473 = case shown="72" w968 {
                        tunnel: w971 -> [w973 w978]
                        tunnel: [w973 w977] -> w970
                        tunnel: w969 -> [_ w976]
                        tunnel: [FALSE TRUE] -> w967
                        frame 0, Default {
                        }
                        frame 72 {
                          n474 = Negate(x=w976) -> (-x=w975:dbl)
                          n475 = call <userlib>:"CONEX-CC Relative Move v2.vi"("Relative displacement"=w975, "Connection Cluster in"=w978) -> ("Connection Cluster out"=w977:T3)  [unwired: 9 in]
                        }
                      }
                    }
                  }
                }
                event Key Repeat {
                  n476 = event-data() -> ("Char"=w984:i16, "ScanCode"=w980:i16)  [unwired: 1 in]
                  n477 = local read "StageY_Step"() -> (w982:dbl)
                  n478 = Divide(x=w982, y=1000.0) -> (x/y=w981:dbl)
                  n479 = case shown="50" w984 {
                    tunnel: w986 -> [w988 w993 w1004]
                    tunnel: [w988 w992 w1003] -> w985
                    tunnel: w981 -> [_ w991 w1002]
                    tunnel: w980 -> [_ w990 w1001]
                    tunnel: [FALSE w989 w1000] -> w979
                    frame 0, Default {
                    }
                    frame 50 {
                      n480 = case shown="80" w990 {
                        tunnel: w993 -> [w995 w999]
                        tunnel: [w995 w998] -> w992
                        tunnel: w991 -> [_ w997]
                        tunnel: [FALSE TRUE] -> w989
                        frame 0, Default {
                        }
                        frame 80 {
                          n481 = call <userlib>:"CONEX-CC Relative Move v2.vi"("Relative displacement"=w997, "Connection Cluster in"=w999) -> ("Connection Cluster out"=w998:T3)  [unwired: 9 in]
                        }
                      }
                    }
                    frame 56 {
                      n482 = case shown="72" w1001 {
                        tunnel: w1004 -> [w1006 w1011]
                        tunnel: [w1006 w1010] -> w1003
                        tunnel: w1002 -> [_ w1009]
                        tunnel: [FALSE TRUE] -> w1000
                        frame 0, Default {
                        }
                        frame 72 {
                          n483 = Negate(x=w1009) -> (-x=w1008:dbl)
                          n484 = call <userlib>:"CONEX-CC Relative Move v2.vi"("Relative displacement"=w1008, "Connection Cluster in"=w1011) -> ("Connection Cluster out"=w1010:T3)  [unwired: 9 in]
                        }
                      }
                    }
                  }
                }
                event "StageY_Home": Value Change {
                  n485 = event-data() -> ()  [unwired: 1 in, 1 out]
                  n486 = call <userlib>:"CONEX-CC Set Velocity v2.vi"("Velocity"=0.1, "Connection Cluster in"=w1020) -> ("Connection Cluster out"=w1019:T3)  [unwired: 9 in]
                  n487 = call <userlib>:"CONEX-CC Absolute Move v2.vi"("Target position"=2.5, "Connection Cluster in"=w1019) -> ("Connection Cluster out"=w1016:T3)  [unwired: 5 in, 2 out]
                  n488 = while {
                    shift-right: [w1021] -> w1014
                    shift-left: w1016 -> [w1025]
                    stop <- w1023 stop-if-true
                    n489 = flat-sequence {
                      tunnel: w1025 -> [w1033]
                      tunnel: [w1032] -> w1024
                      tunnel: [w1031] -> w1022
                      tunnel: w1024 -> [w1037]
                      tunnel: [w1037] -> w1023
                      tunnel: w1022 -> [w1036]
                      tunnel: [w1036] -> w1021
                      frame #0 {
                        n490 = call <userlib>:"CONEX-CC Get Current Position v2.vi"("Connection Cluster in"=w1033) -> ("Current position"=w1030:dbl, "Connection Cluster out"=w1031:T3)  [unwired: 8 in, 1 out]
                        n491 = Subtract(x=w1030, y=2.5) -> (x-y=w1029:dbl)
                        n492 = Multiply(x=1000.0, y=w1029) -> (x*y=w1027:dbl)
                        n493 = local write "StageY_Position"(w1027) -> ()
                        n494 = In Range and Coerce(upper limit=2.501 ("x"), x=w1030, lower limit=2.499 ("x")) -> (In Range?=w1032:bool)  [unwired: 1 out]
                      }
                      frame #1 {
                        n495 = Wait (ms)(milliseconds to wait=u32 1) -> ()  [unwired: 1 out]
                      }
                    }
                  }
                  n496 = call <userlib>:"CONEX-CC Set Velocity v2.vi"("Velocity"=2.0, "Connection Cluster in"=w1014) -> ("Connection Cluster out"=w1013:T3)  [unwired: 9 in]
                }
              }
              n497 = case shown="True" w903 {
                tunnel: [w917 w918] -> w905
                tunnel: w904 -> [w917 w919]
                frame False {
                }
                frame True {
                  w922 = 2000.0 ("upper limit")
                  n498 = Negate(x=w922) -> (-x=w928:dbl)
                  n499 = call <userlib>:"CONEX-CC Get Current Position v2.vi"("Connection Cluster in"=w919) -> ("Current position"=w925:dbl, "Connection Cluster out"=w918:T3)  [unwired: 8 in, 1 out]
                  n500 = Subtract(x=w925, y=2.5) -> (x-y=w926:dbl)
                  n501 = Multiply(x=w926, y=1000.0) -> (x*y=w923:dbl)
                  "StageY_Position" <- w923
                  n502 = In Range and Coerce(upper limit=w922, x=w923, lower limit=w928) -> (In Range?=w927:bool)  [unwired: 1 out]
                  n503 = Not(x=w927) -> (.not. x?=→"StageY_Limit":bool)
                }
              }
              n504 = Unbundle By Name(w905) -> ("error"=w910:errorcluster)
              n505 = Merge Errors(w910, w911) -> (w909:errorcluster)
              n506 = local read "Stage_Step_Select"() -> (w906:bool)
              n507 = case shown="False" w906 {
                frame False {
                  n508 = local write "StageY_Step"("StageY_Step1") -> ()
                }
                frame True {
                  "StageY_Step" <- "StageY_Step2"
                }
              }
              n509 = Wait (ms)(milliseconds to wait=u32 1) -> ()  [unwired: 1 out]
              n510 = Or(x="StageY_Stop", y=w909) -> (x .or. y?=w913:bool)
              n511 = Not(x=w913) -> (.not. x?=→"StageY_ON":bool)
              "?" <- w915
            }
          }
        }
        n512 = Unbundle By Name(w885) -> ("VISA resource name"=w886:refnum<visa-resource-name>)
        n513 = call <userlib>:"_Close Communications.vi"("Instrument Channel"=w886) -> ()  [unwired: 14 in, 1 out]
      }
    }
    n514 = local read "STOP"() -> (w878:bool)
    n515 = Or(x=w878, y=w875) -> (x .or. y?=w877:bool)
    n516 = Wait (ms)(milliseconds to wait=u32 100) -> ()  [unwired: 1 out]
  }
  n517 = while {
    shift-right: [w1043] -> w34
    shift-left: w2 -> [w1039]
    stop <- w1042 stop-if-true
    # "StageZ"
    n518 = case shown="True" "StageZ_Start" {
      tunnel: [w1047 w1057] -> w1043
      tunnel: w1039 -> [w1045 w1052]
      frame False {
        n519 = case shown="False" "VISA_Close" {
          tunnel: [errorcluster {"status"=FALSE, "code"=0, "source"=""} ("error out") w1050] -> w1046
          frame False {
          }
          frame True {
            n520 = VISA Close(VISA resource name="VISA_Selection") -> (error out=w1050:errorcluster)  [unwired: 1 in]
          }
        }
        n521 = Merge Errors(w1046, w1045) -> (w1047:errorcluster)
      }
      frame True {
        n522 = call <userlib>:"VisaInit.vi"("error in (no error)"=w1052, "SerialPort"=u8 8) -> ("error out"=w1055:errorcluster, "Visa Handle"=w1056:refnum<visa-resource-name>)  [unwired: 5 in]
        n523 = Not(x=w1055) -> (.not. x?=w1060:bool)
        n524 = case shown="True" w1060 {
          tunnel: [w1062 w1078] -> w1054
          tunnel: [w1064 w1079] -> w1053
          tunnel: w1056 -> [w1064 w1084]
          tunnel: w1055 -> [w1063 w1083]
          frame False {
            n525 = call <vilib>:"Simple Error Handler.vi"("error in (no error)"=w1063) -> ("error out"=w1062:errorcluster)  [unwired: 4 in, 4 out]
          }
          frame True {
            w1066 = 10000 ("Value")
            w1067 = FALSE ("Query?")
            w1071 = u32 200 ("Delay (ms)")
            n526 = call <userlib>:"Motor ON.vi"("error in (no error)"=w1083, "Delay (ms)"=w1071, "Controller #"="1", "VISA Handle"=w1084) -> ("error out"=w1075:errorcluster, "Dup Controller #"=w1076:string, "Dup VISA Handle"=w1077:refnum<visa-resource-name>)  [unwired: 1 in, 2 out]
            n527 = call <userlib>:"Set Positive Travel Limit.vi"("Value"=w1066, "Query?"=w1067, "error in (no error)"=w1075, "Delay (ms)"=w1071, "Controller #"=w1076, "VISA Handle"=w1077) -> ("error out"=w1072:errorcluster, "Dup Controller #"=w1073:string, "Dup VISA Handle"=w1074:refnum<visa-resource-name>)  [unwired: 2 out]
            n528 = Negate(x=w1066) -> (-x=w1065:i32)
            n529 = call <userlib>:"Set Negative Travel Limit.vi"("Value"=w1065, "Query?"=w1067, "error in (no error)"=w1072, "Delay (ms)"=w1071, "Controller #"=w1073, "VISA Handle"=w1074) -> ("error out"=w1068:errorcluster, "Dup Controller #"=w1069:string, "Dup VISA Handle"=w1070:refnum<visa-resource-name>)  [unwired: 2 out]
            n530 = while "Event Handle Loop" {
              tunnel: w1070 -> [w1106]
              tunnel: [w1098] -> w1080
              tunnel: w1069 -> [w1105]
              tunnel: [w1099] -> w1081
              tunnel: w1068 -> [w1104]
              tunnel: [w1100] -> w1082
              i -> [w1107]
              stop <- w1102 stop-if-true
              # "Stage-Z"
              n531 = local read "Stage_Step_Select"() -> (w1097:bool)
              n532 = case shown="True" w1097 {
                frame False {
                  n533 = local write "StageZ_Step"("StageZ_Step1") -> ()
                }
                frame True {
                  "StageZ_Step" <- "StageZ_Step2"
                }
              }
              n534 = call <userlib>:"Read Position.vi"("error in (no error)"=w1104, "Delay (ms)"=u32 10, "Controller #"=w1105, "VISA Handle"=w1106) -> ("error out"=w1087:errorcluster, "Response"=w1096:string, "Dup Controller #"=w1088:string, "Dup VISA Handle"=w1089:refnum<visa-resource-name>)  [unwired: 1 in, 1 out]
              n535 = Decimal String To Number(string=w1096, offset=5 ("offset (0)")) -> (number=w1094:i32)  [unwired: 1 in, 1 out]
              n536 = Divide(x=w1094, y=100) -> (x/y=→"StageZ_Position":dbl)
              n537 = event shown="[0] Timeout" {
                selector: _ -> [_ _ _ _ _]
                dyn-events: _ -> [_ _ _ _ _]
                timeout: 10 -> [_ _ _ _ _]
                tunnel: w1089 -> [w1113 w1126 w1138 w1145 w1202]
                tunnel: w1088 -> [w1112 w1125 w1137 w1144 w1201]
                tunnel: w1087 -> [w1111 w1124 w1136 w1142 w1199]
                tunnel: [w1113 w1121 w1135 w1141 w1198] -> w1098
                tunnel: [w1112 w1120 w1134 w1140 w1197] -> w1099
                tunnel: [w1111 w1119 w1133 w1139 w1196] -> w1100
                tunnel: 10 -> [_ w1122 w1131 w1143 w1200]
                event Timeout {
                  n538 = event-data() -> ()  [unwired: 1 in, 3 out]
                }
                event "StageZ-": Value Change {
                  n539 = event-data() -> ()  [unwired: 1 in, 1 out]
                  n540 = local read "StageZ_Step"() -> (w1118:dbl)
                  n541 = Multiply(x=100.0 ("y"), y=w1118) -> (x*y=w1116:dbl)
                  n542 = Negate(x=w1116) -> (-x=w1115:dbl)
                  n543 = call <userlib>:"Motion, Relative.vi"("Value"=w1115, "Query?"=FALSE, "error in (no error)"=w1124, "Delay (ms)"=w1122, "Controller #"=w1125, "VISA Handle"=w1126) -> ("error out"=w1119:errorcluster, "Dup Controller #"=w1120:string, "Dup VISA Handle"=w1121:refnum<visa-resource-name>)  [unwired: 2 out]
                  n544 = Wait (ms)(milliseconds to wait=u32 10) -> ()  [unwired: 1 out]
                }
                event "StageZ+": Value Change {
                  n545 = event-data() -> ()  [unwired: 1 in, 1 out]
                  n546 = local read "StageZ_Step"() -> (w1129:dbl)
                  n547 = Multiply(x=100.0 ("y"), y=w1129) -> (x*y=w1130:dbl)
                  n548 = call <userlib>:"Motion, Relative.vi"("Value"=w1130, "Query?"=FALSE, "error in (no error)"=w1136, "Delay (ms)"=w1131, "Controller #"=w1137, "VISA Handle"=w1138) -> ("error out"=w1133:errorcluster, "Dup Controller #"=w1134:string, "Dup VISA Handle"=w1135:refnum<visa-resource-name>)  [unwired: 2 out]
                  n549 = Wait (ms)(milliseconds to wait=u32 10) -> ()  [unwired: 1 out]
                }
                event Key Down {
                  n550 = event-data() -> ("Char"=w1147:i16, "ScanCode"=w1146:i16)  [unwired: 1 in]
                  n551 = case shown="0, Default" w1147 {
                    tunnel: w1146 -> [_ w1158 w1181]
                    tunnel: w1145 -> [w1150 w1157 w1180]
                    tunnel: w1144 -> [w1149 w1156 w1179]
                    tunnel: w1143 -> [_ w1155 w1178]
                    tunnel: w1142 -> [w1148 w1154 w1177]
                    tunnel: [w1148 w1153 w1176] -> w1139
                    tunnel: [w1149 w1152 w1175] -> w1140
                    tunnel: [w1150 w1151 w1174] -> w1141
                    frame 0, Default {
                    }
                    frame 43 {
                      n552 = case shown="78" w1158 {
                        tunnel: w1157 -> [w1161 w1173]
                        tunnel: w1156 -> [w1160 w1172]
                        tunnel: w1155 -> [_ w1171]
                        tunnel: w1154 -> [w1159 w1170]
                        tunnel: [w1161 w1164] -> w1151
                        tunnel: [w1160 w1163] -> w1152
                        tunnel: [w1159 w1162] -> w1153
                        frame 0, Default {
                        }
                        frame 78 {
                          n553 = local read "StageZ_Step"() -> (w1169:dbl)
                          n554 = Multiply(x=100.0 ("y"), y=w1169) -> (x*y=w1167:dbl)
                          n555 = Negate(x=w1167) -> (-x=w1166:dbl)
                          n556 = call <userlib>:"Motion, Relative.vi"("Value"=w1166, "Query?"=FALSE, "error in (no error)"=w1170, "Delay (ms)"=w1171, "Controller #"=w1172, "VISA Handle"=w1173) -> ("error out"=w1162:errorcluster, "Dup Controller #"=w1163:string, "Dup VISA Handle"=w1164:refnum<visa-resource-name>)  [unwired: 2 out]
                        }
                      }
                    }
                    frame 45 {
                      n557 = case shown="74" w1181 {
                        tunnel: w1180 -> [w1184 w1195]
                        tunnel: w1179 -> [w1183 w1194]
                        tunnel: w1178 -> [_ w1193]
                        tunnel: w1177 -> [w1182 w1192]
                        tunnel: [w1184 w1187] -> w1174
                        tunnel: [w1183 w1186] -> w1175
                        tunnel: [w1182 w1185] -> w1176
                        frame 0, Default {
                        }
                        frame 74 {
                          n558 = local read "StageZ_Step"() -> (w1191:dbl)
                          n559 = Multiply(x=100.0 ("y"), y=w1191) -> (x*y=w1189:dbl)
                          n560 = call <userlib>:"Motion, Relative.vi"("Value"=w1189, "Query?"=FALSE, "error in (no error)"=w1192, "Delay (ms)"=w1193, "Controller #"=w1194, "VISA Handle"=w1195) -> ("error out"=w1185:errorcluster, "Dup Controller #"=w1186:string, "Dup VISA Handle"=w1187:refnum<visa-resource-name>)  [unwired: 2 out]
                        }
                      }
                    }
                  }
                }
                event Key Repeat {
                  n561 = event-data() -> ("Char"=w1204:i16, "ScanCode"=w1203:i16)  [unwired: 1 in]
                  n562 = case shown="0, Default" w1204 {
                    tunnel: w1203 -> [_ w1215 w1238]
                    tunnel: w1202 -> [w1207 w1214 w1237]
                    tunnel: w1201 -> [w1206 w1213 w1236]
                    tunnel: w1200 -> [_ w1212 w1235]
                    tunnel: w1199 -> [w1205 w1211 w1234]
                    tunnel: [w1205 w1210 w1233] -> w1196
                    tunnel: [w1206 w1209 w1232] -> w1197
                    tunnel: [w1207 w1208 w1231] -> w1198
                    frame 0, Default {
                    }
                    frame 43 {
                      n563 = case shown="78" w1215 {
                        tunnel: w1214 -> [w1218 w1230]
                        tunnel: w1213 -> [w1217 w1229]
                        tunnel: w1212 -> [_ w1228]
                        tunnel: w1211 -> [w1216 w1227]
                        tunnel: [w1218 w1221] -> w1208
                        tunnel: [w1217 w1220] -> w1209
                        tunnel: [w1216 w1219] -> w1210
                        frame 0, Default {
                        }
                        frame 78 {
                          n564 = local read "StageZ_Step"() -> (w1226:dbl)
                          n565 = Multiply(x=100.0 ("y"), y=w1226) -> (x*y=w1224:dbl)
                          n566 = Negate(x=w1224) -> (-x=w1223:dbl)
                          n567 = call <userlib>:"Motion, Relative.vi"("Value"=w1223, "Query?"=FALSE, "error in (no error)"=w1227, "Delay (ms)"=w1228, "Controller #"=w1229, "VISA Handle"=w1230) -> ("error out"=w1219:errorcluster, "Dup Controller #"=w1220:string, "Dup VISA Handle"=w1221:refnum<visa-resource-name>)  [unwired: 2 out]
                        }
                      }
                    }
                    frame 45 {
                      n568 = case shown="74" w1238 {
                        tunnel: w1237 -> [w1241 w1252]
                        tunnel: w1236 -> [w1240 w1251]
                        tunnel: w1235 -> [_ w1250]
                        tunnel: w1234 -> [w1239 w1249]
                        tunnel: [w1241 w1244] -> w1231
                        tunnel: [w1240 w1243] -> w1232
                        tunnel: [w1239 w1242] -> w1233
                        frame 0, Default {
                        }
                        frame 74 {
                          n569 = local read "StageZ_Step"() -> (w1248:dbl)
                          n570 = Multiply(x=100.0 ("y"), y=w1248) -> (x*y=w1246:dbl)
                          n571 = call <userlib>:"Motion, Relative.vi"("Value"=w1246, "Query?"=FALSE, "error in (no error)"=w1249, "Delay (ms)"=w1250, "Controller #"=w1251, "VISA Handle"=w1252) -> ("error out"=w1242:errorcluster, "Dup Controller #"=w1243:string, "Dup VISA Handle"=w1244:refnum<visa-resource-name>)  [unwired: 2 out]
                        }
                      }
                    }
                  }
                }
              }
              n572 = Or(x=w1100, y="StageZ_Stop") -> (x .or. y?=w1102:bool)
              n573 = Not(x=w1102) -> (.not. x?=→"StageZ_ON":bool)
              n574 = Wait (ms)(milliseconds to wait=u32 1) -> ()  [unwired: 1 out]
              "?" <- w1107
            }
            n575 = call <userlib>:"Motor OFF.vi"("error in (no error)"=w1082, "Controller #"=w1081, "VISA Handle"=w1080) -> ("error out"=w1078:errorcluster, "Dup VISA Handle"=w1079:refnum<visa-resource-name>)  [unwired: 2 in, 3 out]
          }
        }
        n576 = VISA Flush I/O Buffer(VISA resource name=w1053, error in (no error)=w1054) -> (VISA resource name out=w1059:refnum<visa-resource-name>, error out=w1058:errorcluster)  [unwired: 1 in]
        n577 = VISA Close(VISA resource name=w1059, error in (no error)=w1058) -> (error out=w1057:errorcluster)
      }
    }
    n578 = local read "STOP"() -> (w1041:bool)
    n579 = Or(x=w1041, y=w1043) -> (x .or. y?=w1042:bool)
    n580 = Wait (ms)(milliseconds to wait=u32 100) -> ()  [unwired: 1 out]
  }
  n581 = while {
    shift-right: [w1256] -> w32
    shift-left: w2 -> [w1253]
    stop <- w1255 stop-if-true
    # "Position\nKey     Scan  Char\n(X+, D)   30      97\n(X-,  A)   32    100\n(Y+, W)  31    115\n(Y-,  S)    17    119\n(Step, E) 18    101\n(Trap, Q) 16   113"
    # "TrapLaser-Position"
    n582 = case shown="True" "Trap_Position_START" {
      tunnel: [w1259 w1260] -> w1256
      tunnel: w1253 -> [w1259 w1265]
      frame False {
      }
      frame True {
        n583 = local read "PicomotorCmdLib"() -> (w1275:refnum<k24>)
        n584 = local read "PicomotorDevice1"() -> (w1274:string)
        n585 = local read "PicomotorError"() -> (w1266:errorcluster)
        n586 = call "DeviceOpen.vi"("error in (no error)"=w1266, "DeviceKey In"=w1274, "CmdLib In"=w1275) -> ("error out"=w1271:errorcluster, "DeviceKey Out"=w1272:string, "CmdLib Out"=w1273:refnum<k24>)  [unwired: 2 in]
        n587 = call "GetMasterDeviceAddress.vi"("error in (no error)"=w1271, "DeviceKey In"=w1272, "CmdLib In"=w1273) -> ("error out"=w1262:errorcluster, "Device Address"=w1268:i32, "DeviceKey Out"=w1269:string, "CmdLib Out"=w1270:refnum<k24>)  [unwired: 1 in]
        n588 = while "Event Handle Loop" {
          shift-right: [w1282] -> w1267
          shift-left: w1262 -> [w1299]
          tunnel: w1270 -> [w1302]
          tunnel: [w1287] -> w1264
          tunnel: w1269 -> [w1301]
          tunnel: [w1285] -> w1263
          tunnel: w1268 -> [w1300]
          tunnel: [w1280] -> _
          i -> [w1305]
          stop <- w1304 stop-if-true
          # "Template"
          n589 = for {
            N: 4 -> [_]
            tunnel: w1302 -> [w1725]
            tunnel: w1301 -> [w1724]
            tunnel: w1300 -> [w1723]
            shift-right: [w1719] -> w1283
            shift-left: w1299 -> [w1722]
            tunnel: [w1718] -> w1288
            tunnel: [w1717] -> w1286
            tunnel: [w1716] -> w1284
            tunnel: [w1715] -> w1297 mode=indexing
            i -> [w1721]
            n590 = Increment(x=w1721) -> (x+1=w1720:i32)
            n591 = call "GetPosition.vi"("CmdLib In"=w1725, "DeviceKey In"=w1724, "Device Address In"=w1723, "Motor"=w1720, "error in (no error)"=w1722) -> ("CmdLib Out"=w1718:refnum<k24>, "DeviceKey Out"=w1717:string, "Device Address Out"=w1716:i32, "Position"=w1715:i32, "error out"=w1719:errorcluster)  [unwired: 6 in]
          }
          n592 = Index Array(array=w1297, index #1=0 ("index"), index #2=1 ("index"), index #3=2 ("index"), index #4=3 ("index")) -> (element #1=w1292:i32, element #2=w1291:i32, element #3=→"Trap2X_Position":i32, element #4=w1289:i32)
          n593 = Wait (ms)(milliseconds to wait=u32 100) -> ()  [unwired: 1 out]
          n594 = Negate(x=w1292) -> (-x=→"Trap1X_Position":i32)
          n595 = Negate(x=w1289) -> (-x=→"Trap2Y_Position":i32)
          n596 = Negate(x=w1291) -> (-x=→"Trap1Y_Position":i32)
          n597 = event shown="[1] \"TrapX+\": Value Change" {
            selector: _ -> [_ _ _ _ _ _ _ _ _ _ _]
            dyn-events: _ -> [_ _ _ _ _ _ _ _ _ _ _]
            timeout: 100 -> [_ _ _ _ _ _ _ _ _ _ _]
            tunnel: w1288 -> [w1313 w1328 w1343 w1357 w1370 w1382 w1398 w1416 w1430 w1438 w1599]
            tunnel: [w1313 w1321 w1336 w1349 w1362 w1374 w1390 w1408 w1422 w1434 w1595] -> w1287
            tunnel: w1286 -> [w1312 w1327 w1342 w1356 w1369 w1381 w1397 w1415 w1429 w1437 w1598]
            tunnel: [w1312 w1320 w1335 w1348 w1361 w1373 w1389 w1407 w1421 w1433 w1594] -> w1285
            tunnel: w1284 -> [w1311 w1326 w1341 w1355 w1368 w1380 w1396 w1414 w1428 w1436 w1597]
            tunnel: [w1311 w1319 w1334 w1347 w1360 w1372 w1388 w1406 w1420 w1432 w1593] -> w1280
            tunnel: w1283 -> [w1310 w1318 w1333 w1345 w1358 w1379 w1395 w1413 w1427 w1435 w1596]
            tunnel: [w1310 w1322 w1337 w1350 w1363 w1371 w1387 w1405 w1419 w1431 w1592] -> w1282
            event Timeout {
              n598 = event-data() -> ()  [unwired: 1 in, 1 out]
            }
            event "TrapX+": Value Change {
              n599 = event-data() -> ()  [unwired: 1 in, 1 out]
              n600 = local read "Trap_Step"() -> (w1315:dbl)
              n601 = Select(t=u8 3, s="Trap_Select", f=u8 1) -> (s? t:f=w1323:u8)
              n602 = Negate(x=w1315) -> (-x=w1316:dbl)
              n603 = Select(t=w1315, s="Trap_Select", f=w1316) -> (s? t:f=w1314:dbl)
              n604 = call "RelativeMove.vi"("CmdLib In"=w1328, "DeviceKey In"=w1327, "Device Address In"=w1326, "Motor"=w1323, "Relative Steps"=w1314, "error in (no error)"=w1318) -> ("CmdLib Out"=w1321:refnum<k24>, "DeviceKey Out"=w1320:string, "Device Address Out"=w1319:i32, "error out"=w1322:errorcluster)  [unwired: 10 in]
            }
            event "TrapX-": Value Change {
              n605 = event-data() -> ()  [unwired: 1 in, 1 out]
              n606 = local read "Trap_Select"() -> (w1332:bool)
              n607 = local read "Trap_Step"() -> (w1329:dbl)
              n608 = Select(t=u8 3, s=w1332, f=u8 1) -> (s? t:f=w1338:u8)
              n609 = Negate(x=w1329) -> (-x=w1330:dbl)
              n610 = Select(t=w1330, s=w1332, f=w1329) -> (s? t:f=w1331:dbl)
              n611 = call "RelativeMove.vi"("CmdLib In"=w1343, "DeviceKey In"=w1342, "Device Address In"=w1341, "Motor"=w1338, "Relative Steps"=w1331, "error in (no error)"=w1333) -> ("CmdLib Out"=w1336:refnum<k24>, "DeviceKey Out"=w1335:string, "Device Address Out"=w1334:i32, "error out"=w1337:errorcluster)  [unwired: 10 in]
            }
            event "TrapY+": Value Change {
              n612 = event-data() -> ()  [unwired: 1 in, 1 out]
              n613 = local read "Trap_Select"() -> (w1346:bool)
              n614 = local read "Trap_Step"() -> (w1351:dbl)
              n615 = Select(t=u8 4, s=w1346, f=u8 2) -> (s? t:f=w1352:u8)
              n616 = Negate(x=w1351) -> (-x=w1344:dbl)
              n617 = call "RelativeMove.vi"("CmdLib In"=w1357, "DeviceKey In"=w1356, "Device Address In"=w1355, "Motor"=w1352, "Relative Steps"=w1344, "error in (no error)"=w1345) -> ("CmdLib Out"=w1349:refnum<k24>, "DeviceKey Out"=w1348:string, "Device Address Out"=w1347:i32, "error out"=w1350:errorcluster)  [unwired: 10 in]
            }
            event "TrapY-": Value Change {
              n618 = event-data() -> ()  [unwired: 1 in, 1 out]
              n619 = local read "Trap_Select"() -> (w1359:bool)
              n620 = local read "Trap_Step"() -> (w1364:dbl)
              n621 = Select(t=u8 4, s=w1359, f=u8 2) -> (s? t:f=w1365:u8)
              n622 = call "RelativeMove.vi"("CmdLib In"=w1370, "DeviceKey In"=w1369, "Device Address In"=w1368, "Motor"=w1365, "Relative Steps"=w1364, "error in (no error)"=w1358) -> ("CmdLib Out"=w1362:refnum<k24>, "DeviceKey Out"=w1361:string, "Device Address Out"=w1360:i32, "error out"=w1363:errorcluster)  [unwired: 10 in]
            }
            event "Trap1_Home": Value Change {
              n623 = event-data() -> ()  [unwired: 1 in, 1 out]
              n624 = call "AbsoluteMove.vi"("CmdLib In"=w1382, "DeviceKey In"=w1381, "Device Address In"=w1380, "Motor"=1, "Target Pos"=0, "error in (no error)"=w1379) -> ("CmdLib Out"=w1378:refnum<k24>, "DeviceKey Out"=w1377:string, "Device Address Out"=w1376:i32, "error out"=w1375:errorcluster)  [unwired: 10 in]
              n625 = call "AbsoluteMove.vi"("CmdLib In"=w1378, "DeviceKey In"=w1377, "Device Address In"=w1376, "Motor"=2, "Target Pos"=0, "error in (no error)"=w1375) -> ("CmdLib Out"=w1374:refnum<k24>, "DeviceKey Out"=w1373:string, "Device Address Out"=w1372:i32, "error out"=w1371:errorcluster)  [unwired: 10 in]
            }
            event "Trap2_Home": Value Change {
              n626 = event-data() -> ()  [unwired: 1 in, 1 out]
              n627 = call "AbsoluteMove.vi"("CmdLib In"=w1398, "DeviceKey In"=w1397, "Device Address In"=w1396, "Motor"=3, "Target Pos"=0, "error in (no error)"=w1395) -> ("CmdLib Out"=w1394:refnum<k24>, "DeviceKey Out"=w1393:string, "Device Address Out"=w1392:i32, "error out"=w1391:errorcluster)  [unwired: 10 in]
              n628 = call "AbsoluteMove.vi"("CmdLib In"=w1394, "DeviceKey In"=w1393, "Device Address In"=w1392, "Motor"=4, "Target Pos"=0, "error in (no error)"=w1391) -> ("CmdLib Out"=w1390:refnum<k24>, "DeviceKey Out"=w1389:string, "Device Address Out"=w1388:i32, "error out"=w1387:errorcluster)  [unwired: 10 in]
            }
            event "Trap1_Offset": Value Change {
              n629 = event-data() -> ()  [unwired: 1 in, 1 out]
              n630 = call <userlib>:"SetZeroPosition.vi"("CmdLib In"=w1416, "DeviceKey In"=w1415, "Device Address In"=w1414, "Motor"=1, "error in (no error)"=w1413) -> ("CmdLib Out"=w1412:refnum<k24>, "DeviceKey Out"=w1411:string, "Device Address Out"=w1410:i32, "error out"=w1409:errorcluster)  [unwired: 7 in]
              n631 = call <userlib>:"SetZeroPosition.vi"("CmdLib In"=w1412, "DeviceKey In"=w1411, "Device Address In"=w1410, "Motor"=2, "error in (no error)"=w1409) -> ("CmdLib Out"=w1408:refnum<k24>, "DeviceKey Out"=w1407:string, "Device Address Out"=w1406:i32, "error out"=w1405:errorcluster)  [unwired: 7 in]
            }
            event "Trap2_Offset": Value Change {
              n632 = event-data() -> ()  [unwired: 1 in, 1 out]
              n633 = call <userlib>:"SetZeroPosition.vi"("CmdLib In"=w1430, "DeviceKey In"=w1429, "Device Address In"=w1428, "Motor"=3, "error in (no error)"=w1427) -> ("CmdLib Out"=w1426:refnum<k24>, "DeviceKey Out"=w1425:string, "Device Address Out"=w1424:i32, "error out"=w1423:errorcluster)  [unwired: 7 in]
              n634 = call <userlib>:"SetZeroPosition.vi"("CmdLib In"=w1426, "DeviceKey In"=w1425, "Device Address In"=w1424, "Motor"=4, "error in (no error)"=w1423) -> ("CmdLib Out"=w1422:refnum<k24>, "DeviceKey Out"=w1421:string, "Device Address Out"=w1420:i32, "error out"=w1419:errorcluster)  [unwired: 7 in]
            }
            event Key Down {
              n635 = event-data() -> ("ScanCode"=w1440:i16, "Char"=w1439:i16)  [unwired: 1 in]
              n636 = case shown="30" w1440 {
                tunnel: w1439 -> [_ w1453 w1481 w1509 w1535 w1562 w1581]
                tunnel: w1438 -> [w1444 w1452 w1480 w1508 w1534 w1561 w1580]
                tunnel: w1437 -> [w1443 w1451 w1479 w1507 w1533 w1560 w1579]
                tunnel: w1436 -> [w1442 w1450 w1478 w1506 w1532 w1559 w1578]
                tunnel: w1435 -> [w1441 w1449 w1477 w1505 w1531 w1558 w1577]
                tunnel: [w1444 w1448 w1476 w1504 w1530 w1557 w1576] -> w1434
                tunnel: [w1443 w1447 w1475 w1503 w1529 w1556 w1575] -> w1433
                tunnel: [w1442 w1446 w1474 w1502 w1528 w1555 w1574] -> w1432
                tunnel: [w1441 w1445 w1473 w1501 w1527 w1554 w1573] -> w1431
                frame 0, Default {
                }
                frame 30 {
                  n637 = case shown="97" w1453 {
                    tunnel: w1452 -> [w1457 w1468]
                    tunnel: w1451 -> [w1456 w1467]
                    tunnel: w1450 -> [w1455 w1466]
                    tunnel: w1449 -> [w1454 w1465]
                    tunnel: [w1457 w1472] -> w1448
                    tunnel: [w1456 w1471] -> w1447
                    tunnel: [w1455 w1470] -> w1446
                    tunnel: [w1454 w1469] -> w1445
                    frame 0, Default {
                    }
                    frame 97 {
                      n638 = local read "Trap_Select"() -> (w1460:bool)
                      n639 = Select(t=u8 3, s=w1460, f=u8 1) -> (s? t:f=w1462:u8)
                      n640 = local read "Trap_Step"() -> (w1459:dbl)
                      n641 = Negate(x=w1459) -> (-x=w1458:dbl)
                      n642 = Select(t=w1458, s=w1460, f=w1459) -> (s? t:f=w1461:dbl)
                      n643 = call "RelativeMove.vi"("CmdLib In"=w1468, "DeviceKey In"=w1467, "Device Address In"=w1466, "Motor"=w1462, "Relative Steps"=w1461, "error in (no error)"=w1465) -> ("CmdLib Out"=w1472:refnum<k24>, "DeviceKey Out"=w1471:string, "Device Address Out"=w1470:i32, "error out"=w1469:errorcluster)  [unwired: 10 in]
                    }
                  }
                }
                frame 32 {
                  n644 = case shown="100" w1481 {
                    tunnel: w1480 -> [w1485 w1496]
                    tunnel: w1479 -> [w1484 w1495]
                    tunnel: w1478 -> [w1483 w1494]
                    tunnel: w1477 -> [w1482 w1493]
                    tunnel: [w1485 w1500] -> w1476
                    tunnel: [w1484 w1499] -> w1475
                    tunnel: [w1483 w1498] -> w1474
                    tunnel: [w1482 w1497] -> w1473
                    frame 0, Default {
                    }
                    frame 100 {
                      n645 = local read "Trap_Select"() -> (w1489:bool)
                      n646 = Select(t=u8 3, s=w1489, f=u8 1) -> (s? t:f=w1490:u8)
                      n647 = local read "Trap_Step"() -> (w1486:dbl)
                      n648 = Negate(x=w1486) -> (-x=w1487:dbl)
                      n649 = Select(t=w1486, s=w1489, f=w1487) -> (s? t:f=w1488:dbl)
                      n650 = call "RelativeMove.vi"("CmdLib In"=w1496, "DeviceKey In"=w1495, "Device Address In"=w1494, "Motor"=w1490, "Relative Steps"=w1488, "error in (no error)"=w1493) -> ("CmdLib Out"=w1500:refnum<k24>, "DeviceKey Out"=w1499:string, "Device Address Out"=w1498:i32, "error out"=w1497:errorcluster)  [unwired: 10 in]
                    }
                  }
                }
                frame 31 {
                  n651 = case shown="115" w1509 {
                    tunnel: w1508 -> [w1513 w1522]
                    tunnel: w1507 -> [w1512 w1521]
                    tunnel: w1506 -> [w1511 w1520]
                    tunnel: w1505 -> [w1510 w1519]
                    tunnel: [w1513 w1526] -> w1504
                    tunnel: [w1512 w1525] -> w1503
                    tunnel: [w1511 w1524] -> w1502
                    tunnel: [w1510 w1523] -> w1501
                    frame 0, Default {
                    }
                    frame 115 {
                      n652 = local read "Trap_Select"() -> (w1516:bool)
                      n653 = Select(t=u8 4, s=w1516, f=u8 2) -> (s? t:f=w1515:u8)
                      n654 = local read "Trap_Step"() -> (w1514:dbl)
                      n655 = call "RelativeMove.vi"("CmdLib In"=w1522, "DeviceKey In"=w1521, "Device Address In"=w1520, "Motor"=w1515, "Relative Steps"=w1514, "error in (no error)"=w1519) -> ("CmdLib Out"=w1526:refnum<k24>, "DeviceKey Out"=w1525:string, "Device Address Out"=w1524:i32, "error out"=w1523:errorcluster)  [unwired: 10 in]
                    }
                  }
                }
                frame 17 {
                  n656 = case shown="119" w1535 {
                    tunnel: w1534 -> [w1539 w1549]
                    tunnel: w1533 -> [w1538 w1548]
                    tunnel: w1532 -> [w1537 w1547]
                    tunnel: w1531 -> [w1536 w1546]
                    tunnel: [w1539 w1553] -> w1530
                    tunnel: [w1538 w1552] -> w1529
                    tunnel: [w1537 w1551] -> w1528
                    tunnel: [w1536 w1550] -> w1527
                    frame 0, Default {
                    }
                    frame 119 {
                      n657 = local read "Trap_Select"() -> (w1543:bool)
                      n658 = Select(t=u8 4, s=w1543, f=u8 2) -> (s? t:f=w1542:u8)
                      n659 = local read "Trap_Step"() -> (w1541:dbl)
                      n660 = Negate(x=w1541) -> (-x=w1540:dbl)
                      n661 = call "RelativeMove.vi"("CmdLib In"=w1549, "DeviceKey In"=w1548, "Device Address In"=w1547, "Motor"=w1542, "Relative Steps"=w1540, "error in (no error)"=w1546) -> ("CmdLib Out"=w1553:refnum<k24>, "DeviceKey Out"=w1552:string, "Device Address Out"=w1551:i32, "error out"=w1550:errorcluster)  [unwired: 10 in]
                    }
                  }
                }
                frame 18 {
                  n662 = case shown="101" w1562 {
                    tunnel: w1561 -> [w1566 w1572]
                    tunnel: w1560 -> [w1565 w1571]
                    tunnel: w1559 -> [w1564 w1570]
                    tunnel: w1558 -> [w1563 w1569]
                    tunnel: [w1566 w1572] -> w1557
                    tunnel: [w1565 w1571] -> w1556
                    tunnel: [w1564 w1570] -> w1555
                    tunnel: [w1563 w1569] -> w1554
                    frame 0, Default {
                    }
                    frame 101 {
                      n663 = local read "Trap_Step_Select"() -> (w1568:bool)
                      n664 = Not(x=w1568) -> (.not. x?=w1567:bool)
                      n665 = local write "Trap_Step_Select"(w1567) -> ()
                    }
                  }
                }
                frame 16 {
                  n666 = case shown="113" w1581 {
                    tunnel: w1580 -> [w1585 w1591]
                    tunnel: w1579 -> [w1584 w1590]
                    tunnel: w1578 -> [w1583 w1589]
                    tunnel: w1577 -> [w1582 w1588]
                    tunnel: [w1585 w1591] -> w1576
                    tunnel: [w1584 w1590] -> w1575
                    tunnel: [w1583 w1589] -> w1574
                    tunnel: [w1582 w1588] -> w1573
                    frame 0, Default {
                    }
                    frame 113 {
                      n667 = local read "Trap_Select"() -> (w1587:bool)
                      n668 = Not(x=w1587) -> (.not. x?=w1586:bool)
                      n669 = local write "Trap_Select"(w1586) -> ()
                    }
                  }
                }
              }
            }
            event Key Repeat {
              n670 = event-data() -> ("ScanCode"=w1601:i16, "Char"=w1600:i16)  [unwired: 1 in]
              n671 = case shown="30" w1601 {
                tunnel: w1600 -> [_ w1614 w1642 w1670 w1696]
                tunnel: w1599 -> [w1605 w1613 w1641 w1669 w1695]
                tunnel: w1598 -> [w1604 w1612 w1640 w1668 w1694]
                tunnel: w1597 -> [w1603 w1611 w1639 w1667 w1693]
                tunnel: w1596 -> [w1602 w1610 w1638 w1666 w1692]
                tunnel: [w1605 w1609 w1637 w1665 w1691] -> w1595
                tunnel: [w1604 w1608 w1636 w1664 w1690] -> w1594
                tunnel: [w1603 w1607 w1635 w1663 w1689] -> w1593
                tunnel: [w1602 w1606 w1634 w1662 w1688] -> w1592
                frame 0, Default {
                }
                frame 30 {
                  n672 = case shown="97" w1614 {
                    tunnel: w1613 -> [w1618 w1629]
                    tunnel: w1612 -> [w1617 w1628]
                    tunnel: w1611 -> [w1616 w1627]
                    tunnel: w1610 -> [w1615 w1626]
                    tunnel: [w1618 w1633] -> w1609
                    tunnel: [w1617 w1632] -> w1608
                    tunnel: [w1616 w1631] -> w1607
                    tunnel: [w1615 w1630] -> w1606
                    frame 0, Default {
                    }
                    frame 97 {
                      n673 = local read "Trap_Select"() -> (w1621:bool)
                      n674 = Select(t=u8 3, s=w1621, f=u8 1) -> (s? t:f=w1623:u8)
                      n675 = local read "Trap_Step"() -> (w1619:dbl)
                      n676 = Negate(x=w1619) -> (-x=w1620:dbl)
                      n677 = Select(t=w1620, s=w1621, f=w1619) -> (s? t:f=w1622:dbl)
                      n678 = call "RelativeMove.vi"("CmdLib In"=w1629, "DeviceKey In"=w1628, "Device Address In"=w1627, "Motor"=w1623, "Relative Steps"=w1622, "error in (no error)"=w1626) -> ("CmdLib Out"=w1633:refnum<k24>, "DeviceKey Out"=w1632:string, "Device Address Out"=w1631:i32, "error out"=w1630:errorcluster)  [unwired: 10 in]
                    }
                  }
                }
                frame 32 {
                  n679 = case shown="100" w1642 {
                    tunnel: w1641 -> [w1646 w1657]
                    tunnel: w1640 -> [w1645 w1656]
                    tunnel: w1639 -> [w1644 w1655]
                    tunnel: w1638 -> [w1643 w1654]
                    tunnel: [w1646 w1661] -> w1637
                    tunnel: [w1645 w1660] -> w1636
                    tunnel: [w1644 w1659] -> w1635
                    tunnel: [w1643 w1658] -> w1634
                    frame 0, Default {
                    }
                    frame 100 {
                      n680 = local read "Trap_Select"() -> (w1649:bool)
                      n681 = Select(t=u8 3, s=w1649, f=u8 1) -> (s? t:f=w1651:u8)
                      n682 = local read "Trap_Step"() -> (w1648:dbl)
                      n683 = Negate(x=w1648) -> (-x=w1647:dbl)
                      n684 = Select(t=w1648, s=w1649, f=w1647) -> (s? t:f=w1650:dbl)
                      n685 = call "RelativeMove.vi"("CmdLib In"=w1657, "DeviceKey In"=w1656, "Device Address In"=w1655, "Motor"=w1651, "Relative Steps"=w1650, "error in (no error)"=w1654) -> ("CmdLib Out"=w1661:refnum<k24>, "DeviceKey Out"=w1660:string, "Device Address Out"=w1659:i32, "error out"=w1658:errorcluster)  [unwired: 10 in]
                    }
                  }
                }
                frame 31 {
                  n686 = case shown="115" w1670 {
                    tunnel: w1669 -> [w1674 w1683]
                    tunnel: w1668 -> [w1673 w1682]
                    tunnel: w1667 -> [w1672 w1681]
                    tunnel: w1666 -> [w1671 w1680]
                    tunnel: [w1674 w1687] -> w1665
                    tunnel: [w1673 w1686] -> w1664
                    tunnel: [w1672 w1685] -> w1663
                    tunnel: [w1671 w1684] -> w1662
                    frame 0, Default {
                    }
                    frame 115 {
                      n687 = local read "Trap_Select"() -> (w1677:bool)
                      n688 = Select(t=u8 4, s=w1677, f=u8 2) -> (s? t:f=w1676:u8)
                      n689 = local read "Trap_Step"() -> (w1675:dbl)
                      n690 = call "RelativeMove.vi"("CmdLib In"=w1683, "DeviceKey In"=w1682, "Device Address In"=w1681, "Motor"=w1676, "Relative Steps"=w1675, "error in (no error)"=w1680) -> ("CmdLib Out"=w1687:refnum<k24>, "DeviceKey Out"=w1686:string, "Device Address Out"=w1685:i32, "error out"=w1684:errorcluster)  [unwired: 10 in]
                    }
                  }
                }
                frame 17 {
                  n691 = case shown="119" w1696 {
                    tunnel: w1695 -> [w1700 w1710]
                    tunnel: w1694 -> [w1699 w1709]
                    tunnel: w1693 -> [w1698 w1708]
                    tunnel: w1692 -> [w1697 w1707]
                    tunnel: [w1700 w1714] -> w1691
                    tunnel: [w1699 w1713] -> w1690
                    tunnel: [w1698 w1712] -> w1689
                    tunnel: [w1697 w1711] -> w1688
                    frame 0, Default {
                    }
                    frame 119 {
                      n692 = local read "Trap_Select"() -> (w1704:bool)
                      n693 = Select(t=u8 4, s=w1704, f=u8 2) -> (s? t:f=w1703:u8)
                      n694 = local read "Trap_Step"() -> (w1702:dbl)
                      n695 = Negate(x=w1702) -> (-x=w1701:dbl)
                      n696 = call "RelativeMove.vi"("CmdLib In"=w1710, "DeviceKey In"=w1709, "Device Address In"=w1708, "Motor"=w1703, "Relative Steps"=w1701, "error in (no error)"=w1707) -> ("CmdLib Out"=w1714:refnum<k24>, "DeviceKey Out"=w1713:string, "Device Address Out"=w1712:i32, "error out"=w1711:errorcluster)  [unwired: 10 in]
                    }
                  }
                }
              }
            }
          }
          n697 = case shown="True" "Trap_Step_Select" {
            frame False {
              n698 = local write "Trap_Step"("Trap_Step1") -> ()
            }
            frame True {
              "Trap_Step" <- "Trap_Step2"
            }
          }
          n699 = Or(x=w1282, y="Trap_Position_STOP") -> (x .or. y?=w1304:bool)
          n700 = Not(x=w1304) -> (.not. x?=→"Trap_Position_ON":bool)
          "Trap_Position_Num" <- w1305
        }
        n701 = call "DeviceClose.vi"("error in (no error)"=w1267, "DeviceKey In"=w1263, "CmdLib In"=w1264) -> ("error out"=w1261:errorcluster)  [unwired: 2 in, 2 out]
        n702 = Merge Errors(w1261, w1265) -> (w1260:errorcluster)
      }
    }
    n703 = local read "STOP"() -> (w1254:bool)
    n704 = Or(x=w1254, y=w1256) -> (x .or. y?=w1255:bool)
    n705 = Wait (ms)(milliseconds to wait=u32 100) -> ()  [unwired: 1 out]
  }
  n706 = while {
    shift-right: [w1728] -> w31
    shift-left: w2 -> [w1727]
    stop <- w1729 stop-if-true
    # "Position\nKey     Scan  Char\n(X+, L)    38   108\n(X-,  J)     36   106\n(Y+, I)     37   107\n(Y-,  K)    23   105\n(Det, U) 22   117\n(Step, O)  24   111"
    # "DetectionLaser-Position"
    n707 = case shown="True" "Det_Position_START" {
      tunnel: [w1732 w1735] -> w1728
      tunnel: w1727 -> [w1732 w1733]
      frame False {
      }
      frame True {
        n708 = local read "PicomotorCmdLib"() -> (w1746:refnum<k24>)
        n709 = local read "PicomotorDevice2"() -> (w1747:string)
        n710 = local read "PicomotorError"() -> (w1748:errorcluster)
        n711 = call "DeviceOpen.vi"("error in (no error)"=w1748, "DeviceKey In"=w1747, "CmdLib In"=w1746) -> ("error out"=w1743:errorcluster, "DeviceKey Out"=w1744:string, "CmdLib Out"=w1745:refnum<k24>)  [unwired: 2 in]
        n712 = call "GetMasterDeviceAddress.vi"("error in (no error)"=w1743, "DeviceKey In"=w1744, "CmdLib In"=w1745) -> ("error out"=w1739:errorcluster, "Device Address"=w1740:i32, "DeviceKey Out"=w1741:string, "CmdLib Out"=w1742:refnum<k24>)  [unwired: 1 in]
        n713 = while {
          shift-right: [w1754] -> w1736
          shift-left: w1739 -> [w1768]
          tunnel: w1742 -> [w1771]
          tunnel: [w1758] -> w1738
          tunnel: w1741 -> [w1770]
          tunnel: [w1757] -> w1737
          tunnel: w1740 -> [w1769]
          tunnel: [w1756] -> _
          i -> [w1778]
          stop <- w1753 stop-if-true
          n714 = for {
            N: 4 -> [_]
            shift-right: [w2184] -> w1759
            shift-left: w1768 -> [w2187]
            tunnel: [w2183] -> w1762
            tunnel: [w2182] -> w1761
            tunnel: [w2181] -> w1760
            tunnel: [w2180] -> w1776 mode=indexing
            tunnel: w1771 -> [w2179]
            tunnel: w1770 -> [w2178]
            tunnel: w1769 -> [w2177]
            i -> [w2186]
            n715 = Increment(x=w2186) -> (x+1=w2185:i32)
            n716 = call "GetPosition.vi"("CmdLib In"=w2179, "DeviceKey In"=w2178, "Device Address In"=w2177, "Motor"=w2185, "error in (no error)"=w2187) -> ("CmdLib Out"=w2183:refnum<k24>, "DeviceKey Out"=w2182:string, "Device Address Out"=w2181:i32, "Position"=w2180:i32, "error out"=w2184:errorcluster)  [unwired: 6 in]
          }
          n717 = Index Array(array=w1776, index #1=0 ("index"), index #2=1 ("index"), index #3=2 ("index"), index #4=3 ("index")) -> (element #1=→"Detection1X_Position":i32, element #2=w1766:i32, element #3=→"Detection2X_Position":i32, element #4=w1764:i32)
          n718 = Wait (ms)(milliseconds to wait=u32 100) -> ()  [unwired: 1 out]
          n719 = Negate(x=w1766) -> (-x=→"Detection1Y_Position":i32)
          n720 = Negate(x=w1764) -> (-x=→"Detection2Y_Position":i32)
          n721 = event shown="[0] Timeout" {
            selector: _ -> [_ _ _ _ _ _ _ _ _ _ _]
            dyn-events: _ -> [_ _ _ _ _ _ _ _ _ _ _]
            timeout: 100 -> [_ _ _ _ _ _ _ _ _ _ _]
            tunnel: [w1785 w1795 w1808 w1821 w1835 w1847 w1863 w1881 w1895 w1907 w2064] -> w1758
            tunnel: [w1784 w1794 w1807 w1820 w1834 w1846 w1862 w1880 w1894 w1906 w2063] -> w1757
            tunnel: [w1783 w1793 w1806 w1819 w1833 w1845 w1861 w1879 w1893 w1905 w2062] -> w1756
            tunnel: [w1782 w1796 w1809 w1822 w1836 w1844 w1860 w1878 w1892 w1904 w2061] -> w1754
            tunnel: w1762 -> [w1785 w1791 w1804 w1816 w1830 w1843 w1859 w1875 w1889 w1903 w2060]
            tunnel: w1761 -> [w1784 w1790 w1803 w1815 w1829 w1842 w1858 w1874 w1888 w1902 w2059]
            tunnel: w1760 -> [w1783 w1789 w1802 w1814 w1828 w1841 w1857 w1873 w1887 w1901 w2058]
            tunnel: w1759 -> [w1782 w1787 w1801 w1813 w1827 w1840 w1856 w1872 w1886 w1900 w2057]
            event Timeout {
              n722 = event-data() -> ()  [unwired: 1 in, 1 out]
            }
            event "DetX+": Value Change {
              n723 = event-data() -> ()  [unwired: 1 in, 1 out]
              n724 = local read "Det_Step"() -> (w1788:dbl)
              n725 = Select(t=u8 3, s="Det_Select", f=u8 1) -> (s? t:f=w1797:u8)
              n726 = Negate(x=w1788) -> (-x=w1786:dbl)
              n727 = call "RelativeMove.vi"("CmdLib In"=w1791, "DeviceKey In"=w1790, "Device Address In"=w1789, "Motor"=w1797, "Relative Steps"=w1786, "error in (no error)"=w1787) -> ("CmdLib Out"=w1795:refnum<k24>, "DeviceKey Out"=w1794:string, "Device Address Out"=w1793:i32, "error out"=w1796:errorcluster)  [unwired: 10 in]
            }
            event "DetX-": Value Change {
              n728 = event-data() -> ()  [unwired: 1 in, 1 out]
              n729 = local read "Det_Select"() -> (w1805:bool)
              n730 = local read "Det_Step"() -> (w1800:dbl)
              n731 = Select(t=u8 3, s=w1805, f=u8 1) -> (s? t:f=w1810:u8)
              n732 = call "RelativeMove.vi"("CmdLib In"=w1804, "DeviceKey In"=w1803, "Device Address In"=w1802, "Motor"=w1810, "Relative Steps"=w1800, "error in (no error)"=w1801) -> ("CmdLib Out"=w1808:refnum<k24>, "DeviceKey Out"=w1807:string, "Device Address Out"=w1806:i32, "error out"=w1809:errorcluster)  [unwired: 10 in]
            }
            event "DetY+": Value Change {
              n733 = event-data() -> ()  [unwired: 1 in, 4 out]
              n734 = local read "Det_Select"() -> (w1818:bool)
              n735 = local read "Det_Step"() -> (w1817:dbl)
              n736 = Select(t=u8 4, s=w1818, f=u8 2) -> (s? t:f=w1823:u8)
              n737 = call "RelativeMove.vi"("CmdLib In"=w1816, "DeviceKey In"=w1815, "Device Address In"=w1814, "Motor"=w1823, "Relative Steps"=w1817, "error in (no error)"=w1813) -> ("CmdLib Out"=w1821:refnum<k24>, "DeviceKey Out"=w1820:string, "Device Address Out"=w1819:i32, "error out"=w1822:errorcluster)  [unwired: 10 in]
            }
            event "DetY-": Value Change {
              n738 = event-data() -> ()  [unwired: 1 in, 1 out]
              n739 = local read "Det_Select"() -> (w1832:bool)
              n740 = local read "Det_Step"() -> (w1831:dbl)
              n741 = Select(t=u8 4, s=w1832, f=u8 2) -> (s? t:f=w1837:u8)
              n742 = Negate(x=w1831) -> (-x=w1826:dbl)
              n743 = call "RelativeMove.vi"("CmdLib In"=w1830, "DeviceKey In"=w1829, "Device Address In"=w1828, "Motor"=w1837, "Relative Steps"=w1826, "error in (no error)"=w1827) -> ("CmdLib Out"=w1835:refnum<k24>, "DeviceKey Out"=w1834:string, "Device Address Out"=w1833:i32, "error out"=w1836:errorcluster)  [unwired: 10 in]
            }
            event "Det1_Home": Value Change {
              n744 = event-data() -> ()  [unwired: 1 in, 1 out]
              n745 = call "AbsoluteMove.vi"("CmdLib In"=w1843, "DeviceKey In"=w1842, "Device Address In"=w1841, "Motor"=1, "Target Pos"=0, "error in (no error)"=w1840) -> ("CmdLib Out"=w1851:refnum<k24>, "DeviceKey Out"=w1850:string, "Device Address Out"=w1849:i32, "error out"=w1848:errorcluster)  [unwired: 10 in]
              n746 = call "AbsoluteMove.vi"("CmdLib In"=w1851, "DeviceKey In"=w1850, "Device Address In"=w1849, "Motor"=2, "Target Pos"=0, "error in (no error)"=w1848) -> ("CmdLib Out"=w1847:refnum<k24>, "DeviceKey Out"=w1846:string, "Device Address Out"=w1845:i32, "error out"=w1844:errorcluster)  [unwired: 10 in]
            }
            event "Det2_Home": Value Change {
              n747 = event-data() -> ()  [unwired: 1 in, 1 out]
              n748 = call "AbsoluteMove.vi"("CmdLib In"=w1859, "DeviceKey In"=w1858, "Device Address In"=w1857, "Motor"=3, "Target Pos"=0, "error in (no error)"=w1856) -> ("CmdLib Out"=w1867:refnum<k24>, "DeviceKey Out"=w1866:string, "Device Address Out"=w1865:i32, "error out"=w1864:errorcluster)  [unwired: 10 in]
              n749 = call "AbsoluteMove.vi"("CmdLib In"=w1867, "DeviceKey In"=w1866, "Device Address In"=w1865, "Motor"=4, "Target Pos"=0, "error in (no error)"=w1864) -> ("CmdLib Out"=w1863:refnum<k24>, "DeviceKey Out"=w1862:string, "Device Address Out"=w1861:i32, "error out"=w1860:errorcluster)  [unwired: 10 in]
            }
            event "Det1_Offset": Value Change {
              n750 = event-data() -> ()  [unwired: 1 in, 1 out]
              n751 = call <userlib>:"SetZeroPosition.vi"("CmdLib In"=w1875, "DeviceKey In"=w1874, "Device Address In"=w1873, "Motor"=1, "error in (no error)"=w1872) -> ("CmdLib Out"=w1885:refnum<k24>, "DeviceKey Out"=w1884:string, "Device Address Out"=w1883:i32, "error out"=w1882:errorcluster)  [unwired: 7 in]
              n752 = call <userlib>:"SetZeroPosition.vi"("CmdLib In"=w1885, "DeviceKey In"=w1884, "Device Address In"=w1883, "Motor"=2, "error in (no error)"=w1882) -> ("CmdLib Out"=w1881:refnum<k24>, "DeviceKey Out"=w1880:string, "Device Address Out"=w1879:i32, "error out"=w1878:errorcluster)  [unwired: 7 in]
            }
            event "Det2_Offset": Value Change {
              n753 = event-data() -> ()  [unwired: 1 in, 1 out]
              n754 = call <userlib>:"SetZeroPosition.vi"("CmdLib In"=w1889, "DeviceKey In"=w1888, "Device Address In"=w1887, "Motor"=3, "error in (no error)"=w1886) -> ("CmdLib Out"=w1899:refnum<k24>, "DeviceKey Out"=w1898:string, "Device Address Out"=w1897:i32, "error out"=w1896:errorcluster)  [unwired: 7 in]
              n755 = call <userlib>:"SetZeroPosition.vi"("CmdLib In"=w1899, "DeviceKey In"=w1898, "Device Address In"=w1897, "Motor"=4, "error in (no error)"=w1896) -> ("CmdLib Out"=w1895:refnum<k24>, "DeviceKey Out"=w1894:string, "Device Address Out"=w1893:i32, "error out"=w1892:errorcluster)  [unwired: 7 in]
            }
            event Key Down {
              n756 = event-data() -> ("ScanCode"=w1909:i16, "Char"=w1908:i16)  [unwired: 1 in]
              n757 = case shown="0, Default" w1909 {
                tunnel: w1908 -> [_ w1922 w1949 w1975 w2002 w2027 w2046]
                tunnel: [w1913 w1921 w1948 w1974 w2001 w2022 w2041] -> w1907
                tunnel: [w1912 w1920 w1947 w1973 w2000 w2021 w2040] -> w1906
                tunnel: [w1911 w1919 w1946 w1972 w1999 w2020 w2039] -> w1905
                tunnel: [w1910 w1918 w1945 w1971 w1998 w2019 w2038] -> w1904
                tunnel: w1903 -> [w1913 w1917 w1944 w1970 w1996 w2026 w2045]
                tunnel: w1902 -> [w1912 w1916 w1943 w1969 w1995 w2025 w2044]
                tunnel: w1901 -> [w1911 w1915 w1942 w1968 w1994 w2024 w2043]
                tunnel: w1900 -> [w1910 w1914 w1941 w1967 w1997 w2023 w2042]
                frame 0, Default {
                }
                frame 38 {
                  n758 = case shown="108" w1922 {
                    tunnel: [w1926 w1940] -> w1921
                    tunnel: [w1925 w1939] -> w1920
                    tunnel: [w1924 w1938] -> w1919
                    tunnel: [w1923 w1937] -> w1918
                    tunnel: w1917 -> [w1926 w1930]
                    tunnel: w1916 -> [w1925 w1929]
                    tunnel: w1915 -> [w1924 w1928]
                    tunnel: w1914 -> [w1923 w1931]
                    frame 0, Default {
                    }
                    frame 108 {
                      n759 = local read "Det_Select"() -> (w1934:bool)
                      n760 = Select(t=u8 3, s=w1934, f=u8 1) -> (s? t:f=w1933:u8)
                      n761 = local read "Det_Step"() -> (w1932:dbl)
                      n762 = Negate(x=w1932) -> (-x=w1927:dbl)
                      n763 = call "RelativeMove.vi"("CmdLib In"=w1930, "DeviceKey In"=w1929, "Device Address In"=w1928, "Motor"=w1933, "Relative Steps"=w1927, "error in (no error)"=w1931) -> ("CmdLib Out"=w1940:refnum<k24>, "DeviceKey Out"=w1939:string, "Device Address Out"=w1938:i32, "error out"=w1937:errorcluster)  [unwired: 10 in]
                    }
                  }
                }
                frame 36 {
                  n764 = case shown="106" w1949 {
                    tunnel: [w1953 w1966] -> w1948
                    tunnel: [w1952 w1965] -> w1947
                    tunnel: [w1951 w1964] -> w1946
                    tunnel: [w1950 w1963] -> w1945
                    tunnel: w1944 -> [w1953 w1954]
                    tunnel: w1943 -> [w1952 w1955]
                    tunnel: w1942 -> [w1951 w1956]
                    tunnel: w1941 -> [w1950 w1957]
                    frame 0, Default {
                    }
                    frame 106 {
                      n765 = local read "Det_Select"() -> (w1960:bool)
                      n766 = Select(t=u8 3, s=w1960, f=u8 1) -> (s? t:f=w1959:u8)
                      n767 = local read "Det_Step"() -> (w1958:dbl)
                      n768 = call "RelativeMove.vi"("CmdLib In"=w1954, "DeviceKey In"=w1955, "Device Address In"=w1956, "Motor"=w1959, "Relative Steps"=w1958, "error in (no error)"=w1957) -> ("CmdLib Out"=w1966:refnum<k24>, "DeviceKey Out"=w1965:string, "Device Address Out"=w1964:i32, "error out"=w1963:errorcluster)  [unwired: 10 in]
                    }
                  }
                }
                frame 37 {
                  n769 = case shown="107" w1975 {
                    tunnel: [w1979 w1993] -> w1974
                    tunnel: [w1978 w1992] -> w1973
                    tunnel: [w1977 w1991] -> w1972
                    tunnel: [w1976 w1990] -> w1971
                    tunnel: w1970 -> [w1979 w1984]
                    tunnel: w1969 -> [w1978 w1983]
                    tunnel: w1968 -> [w1977 w1982]
                    tunnel: w1967 -> [w1976 w1981]
                    frame 0, Default {
                    }
                    frame 107 {
                      n770 = local read "Det_Select"() -> (w1987:bool)
                      n771 = Select(t=u8 4, s=w1987, f=u8 2) -> (s? t:f=w1986:u8)
                      n772 = local read "Det_Step"() -> (w1985:dbl)
                      n773 = Negate(x=w1985) -> (-x=w1980:dbl)
                      n774 = call "RelativeMove.vi"("CmdLib In"=w1984, "DeviceKey In"=w1983, "Device Address In"=w1982, "Motor"=w1986, "Relative Steps"=w1980, "error in (no error)"=w1981) -> ("CmdLib Out"=w1993:refnum<k24>, "DeviceKey Out"=w1992:string, "Device Address Out"=w1991:i32, "error out"=w1990:errorcluster)  [unwired: 10 in]
                    }
                  }
                }
                frame 23 {
                  n775 = case shown="105" w2002 {
                    tunnel: [w2006 w2018] -> w2001
                    tunnel: [w2005 w2017] -> w2000
                    tunnel: [w2004 w2016] -> w1999
                    tunnel: [w2003 w2015] -> w1998
                    tunnel: w1997 -> [w2003 _]
                    tunnel: w1996 -> [w2006 w2009]
                    tunnel: w1995 -> [w2005 w2008]
                    tunnel: w1994 -> [w2004 w2007]
                    frame 0, Default {
                    }
                    frame 105 {
                      n776 = local read "Det_Select"() -> (w2012:bool)
                      n777 = Select(t=u8 4, s=w2012, f=u8 2) -> (s? t:f=w2011:u8)
                      n778 = local read "Det_Step"() -> (w2010:dbl)
                      n779 = call "RelativeMove.vi"("CmdLib In"=w2009, "DeviceKey In"=w2008, "Device Address In"=w2007, "Motor"=w2011, "Relative Steps"=w2010) -> ("CmdLib Out"=w2018:refnum<k24>, "DeviceKey Out"=w2017:string, "Device Address Out"=w2016:i32, "error out"=w2015:errorcluster)  [unwired: 11 in]
                    }
                  }
                }
                frame 24 {
                  n780 = case shown="111" w2027 {
                    tunnel: w2026 -> [w2031 w2032]
                    tunnel: w2025 -> [w2030 w2033]
                    tunnel: w2024 -> [w2029 w2034]
                    tunnel: w2023 -> [w2028 w2035]
                    tunnel: [w2028 w2035] -> w2019
                    tunnel: [w2029 w2034] -> w2020
                    tunnel: [w2030 w2033] -> w2021
                    tunnel: [w2031 w2032] -> w2022
                    frame 0, Default {
                    }
                    frame 111 {
                      n781 = local read "Detection_Step_Select"() -> (w2037:bool)
                      n782 = Not(x=w2037) -> (.not. x?=w2036:bool)
                      n783 = local write "Detection_Step_Select"(w2036) -> ()
                    }
                  }
                }
                frame 22 {
                  n784 = case shown="117" w2046 {
                    tunnel: w2045 -> [w2050 w2054]
                    tunnel: w2044 -> [w2049 w2053]
                    tunnel: w2043 -> [w2048 w2052]
                    tunnel: w2042 -> [w2047 w2051]
                    tunnel: [w2050 w2054] -> w2041
                    tunnel: [w2049 w2053] -> w2040
                    tunnel: [w2048 w2052] -> w2039
                    tunnel: [w2047 w2051] -> w2038
                    frame 0, Default {
                    }
                    frame 117 {
                      n785 = local read "Det_Select"() -> (w2056:bool)
                      n786 = Not(x=w2056) -> (.not. x?=w2055:bool)
                      n787 = local write "Det_Select"(w2055) -> ()
                    }
                  }
                }
              }
            }
            event Key Repeat {
              n788 = event-data() -> ("ScanCode"=w2066:i16, "Char"=w2065:i16)  [unwired: 1 in]
              n789 = case shown="0, Default" w2066 {
                tunnel: w2065 -> [_ w2079 w2106 w2132 w2159]
                tunnel: [w2070 w2078 w2105 w2131 w2158] -> w2064
                tunnel: [w2069 w2077 w2104 w2130 w2157] -> w2063
                tunnel: [w2068 w2076 w2103 w2129 w2156] -> w2062
                tunnel: [w2067 w2075 w2102 w2128 w2155] -> w2061
                tunnel: w2060 -> [w2070 w2074 w2101 w2124 w2151]
                tunnel: w2059 -> [w2069 w2073 w2100 w2125 w2152]
                tunnel: w2058 -> [w2068 w2071 w2099 w2126 w2153]
                tunnel: w2057 -> [w2067 w2072 w2098 w2127 w2154]
                frame 0, Default {
                }
                frame 38 {
                  n790 = case shown="108" w2079 {
                    tunnel: [w2083 w2097] -> w2078
                    tunnel: [w2082 w2096] -> w2077
                    tunnel: [w2081 w2095] -> w2076
                    tunnel: [w2080 w2094] -> w2075
                    tunnel: w2074 -> [w2083 w2088]
                    tunnel: w2073 -> [w2082 w2087]
                    tunnel: w2072 -> [w2080 w2085]
                    tunnel: w2071 -> [w2081 w2086]
                    frame 0, Default {
                    }
                    frame 108 {
                      n791 = local read "Det_Select"() -> (w2091:bool)
                      n792 = Select(t=u8 3, s=w2091, f=u8 1) -> (s? t:f=w2090:u8)
                      n793 = local read "Det_Step"() -> (w2089:dbl)
                      n794 = Negate(x=w2089) -> (-x=w2084:dbl)
                      n795 = call "RelativeMove.vi"("CmdLib In"=w2088, "DeviceKey In"=w2087, "Device Address In"=w2086, "Motor"=w2090, "Relative Steps"=w2084, "error in (no error)"=w2085) -> ("CmdLib Out"=w2097:refnum<k24>, "DeviceKey Out"=w2096:string, "Device Address Out"=w2095:i32, "error out"=w2094:errorcluster)  [unwired: 10 in]
                    }
                  }
                }
                frame 36 {
                  n796 = case shown="106" w2106 {
                    tunnel: [w2110 w2123] -> w2105
                    tunnel: [w2109 w2122] -> w2104
                    tunnel: [w2108 w2121] -> w2103
                    tunnel: [w2107 w2120] -> w2102
                    tunnel: w2101 -> [w2110 w2114]
                    tunnel: w2100 -> [w2109 w2113]
                    tunnel: w2099 -> [w2108 w2112]
                    tunnel: w2098 -> [w2107 w2111]
                    frame 0, Default {
                    }
                    frame 106 {
                      n797 = local read "Det_Select"() -> (w2117:bool)
                      n798 = Select(t=u8 3, s=w2117, f=u8 1) -> (s? t:f=w2116:u8)
                      n799 = local read "Det_Step"() -> (w2115:dbl)
                      n800 = call "RelativeMove.vi"("CmdLib In"=w2114, "DeviceKey In"=w2113, "Device Address In"=w2112, "Motor"=w2116, "Relative Steps"=w2115, "error in (no error)"=w2111) -> ("CmdLib Out"=w2123:refnum<k24>, "DeviceKey Out"=w2122:string, "Device Address Out"=w2121:i32, "error out"=w2120:errorcluster)  [unwired: 10 in]
                    }
                  }
                }
                frame 37 {
                  n801 = case shown="107" w2132 {
                    tunnel: [w2136 w2150] -> w2131
                    tunnel: [w2135 w2149] -> w2130
                    tunnel: [w2134 w2148] -> w2129
                    tunnel: [w2133 w2147] -> w2128
                    tunnel: w2127 -> [w2133 w2141]
                    tunnel: w2126 -> [w2134 w2140]
                    tunnel: w2125 -> [w2135 w2139]
                    tunnel: w2124 -> [w2136 w2138]
                    frame 0, Default {
                    }
                    frame 107 {
                      n802 = local read "Det_Select"() -> (w2144:bool)
                      n803 = Select(t=u8 4, s=w2144, f=u8 2) -> (s? t:f=w2143:u8)
                      n804 = local read "Det_Step"() -> (w2142:dbl)
                      n805 = Negate(x=w2142) -> (-x=w2137:dbl)
                      n806 = call "RelativeMove.vi"("CmdLib In"=w2138, "DeviceKey In"=w2139, "Device Address In"=w2140, "Motor"=w2143, "Relative Steps"=w2137, "error in (no error)"=w2141) -> ("CmdLib Out"=w2150:refnum<k24>, "DeviceKey Out"=w2149:string, "Device Address Out"=w2148:i32, "error out"=w2147:errorcluster)  [unwired: 10 in]
                    }
                  }
                }
                frame 23 {
                  n807 = case shown="105" w2159 {
                    tunnel: [w2163 w2176] -> w2158
                    tunnel: [w2162 w2175] -> w2157
                    tunnel: [w2161 w2174] -> w2156
                    tunnel: [w2160 w2173] -> w2155
                    tunnel: w2154 -> [w2160 w2167]
                    tunnel: w2153 -> [w2161 w2164]
                    tunnel: w2152 -> [w2162 w2165]
                    tunnel: w2151 -> [w2163 w2166]
                    frame 0, Default {
                    }
                    frame 105 {
                      n808 = local read "Det_Select"() -> (w2170:bool)
                      n809 = Select(t=u8 4, s=w2170, f=u8 2) -> (s? t:f=w2169:u8)
                      n810 = local read "Det_Step"() -> (w2168:dbl)
                      n811 = call "RelativeMove.vi"("CmdLib In"=w2166, "DeviceKey In"=w2165, "Device Address In"=w2164, "Motor"=w2169, "Relative Steps"=w2168, "error in (no error)"=w2167) -> ("CmdLib Out"=w2176:refnum<k24>, "DeviceKey Out"=w2175:string, "Device Address Out"=w2174:i32, "error out"=w2173:errorcluster)  [unwired: 10 in]
                    }
                  }
                }
              }
            }
          }
          n812 = case shown="True" "Detection_Step_Select" {
            frame False {
              n813 = local write "Det_Step"("Det_Step1") -> ()
            }
            frame True {
              "Det_Step" <- "Det_Step2"
            }
          }
          n814 = Or(x="Det_Position_STOP", y=w1754) -> (x .or. y?=w1753:bool)
          n815 = Not(x=w1753) -> (.not. x?=→"Detection_Position_ON":bool)
          "Det_Position_Num" <- w1778
        }
        n816 = call "DeviceClose.vi"("error in (no error)"=w1736, "DeviceKey In"=w1737, "CmdLib In"=w1738) -> ("error out"=w1734:errorcluster)  [unwired: 2 in, 2 out]
        n817 = Merge Errors(w1734, w1733) -> (w1735:errorcluster)
      }
    }
    n818 = local read "STOP"() -> (w1730:bool)
    n819 = Or(x=w1730, y=w1728) -> (x .or. y?=w1729:bool)
    n820 = Wait (ms)(milliseconds to wait=u32 100) -> ()  [unwired: 1 out]
  }
  n821 = while {
    shift-right: [w2191] -> w22
    shift-left: w2 -> [w2192]
    shift-right: [w2188] -> w4
    shift-left: w10 -> [w2189]
    stop <- w2194 stop-if-true
    # "MTA"
    n822 = case shown="True" "MTA_START" {
      tunnel: w2192 -> [w2196 w2200]
      tunnel: [w2196 w2199] -> w2191
      tunnel: w2189 -> [w2195 w2198]
      tunnel: [w2195 w2197] -> w2188
      frame False {
      }
      frame True {
        n823 = while "Event Handle Loop" {
          shift-right: [w2219] -> w2199
          shift-left: w2200 -> [w2218]
          shift-right: [w2202] -> w2197
          shift-left: w2198 -> [w2215]
          i -> [w2223]
          stop <- w2221 stop-if-true
          # "Template"
          n824 = Select(t="MTA_Step2", s="MTA_Step_Select", f="MTA_Step1") -> (s? t:f=w2207:dbl)
          "MTA_Step" <- w2207
          n825 = event shown="[3] \"MTAX+\": Value Change" {
            selector: _ -> [_ _ _ _ _ _ _ _ _]
            dyn-events: _ -> [_ _ _ _ _ _ _ _ _]
            timeout: 10 -> [_ _ _ _ _ _ _ _ _]
            tunnel: [FALSE w2326 w2328 TRUE TRUE TRUE TRUE TRUE TRUE] -> w2216
            tunnel: w2215 -> [w2324 _ _ w2338 w2364 w2390 w2416 w2440 w2605]
            tunnel: [w2324 T2 {"MTA1X"=0.0, "MTA1Y"=0.0, "MTA2X"=0.0, "MTA2Y"=0.0} ("output cluster") T2 {"MTA1X"=5.0, "MTA1Y"=5.0, "MTA2X"=5.0, "MTA2Y"=5.0} ("output cluster") w2339 w2365 w2391 w2417 w2441 w2606] -> w2201
            tunnel: w2207 -> [_ _ _ w2332 w2358 w2384 w2410 w2438 w2603]
            tunnel: "MTA_Select" -> [_ _ _ w2333 w2359 w2385 w2411 w2439 w2604]
            tunnel: [TRUE w2326 w2328 w2331 w2357 w2383 w2409 w2437 w2602] -> w2206
            event Timeout {
              n826 = event-data() -> ()  [unwired: 1 in, 2 out]
            }
            event "MTA_Zero": Value Change {
              w2326 = TRUE
              n827 = event-data() -> ()  [unwired: 1 in, 6 out]
            }
            event "MTA_Home": Value Change {
              w2328 = TRUE
              n828 = event-data() -> ()  [unwired: 1 in, 1 out]
            }
            event "MTAX+": Value Change {
              n829 = event-data() -> ()  [unwired: 1 in, 1 out]
              n830 = Unbundle By Name(w2338) -> ("MTA1X"=w2337:dbl, "MTA2X"=w2336:dbl)
              n831 = case shown="True" w2333 {
                tunnel: w2337 -> [w2341 w2355]
                tunnel: [w2340 w2355] -> w2335
                tunnel: w2336 -> [w2347 w2354]
                tunnel: [w2347 w2348] -> w2334
                tunnel: w2332 -> [w2342 w2353]
                tunnel: [w2343 w2349] -> w2331
                frame False {
                  n832 = Subtract(x=w2341, y=w2342) -> (x-y=w2346:dbl)
                  n833 = In Range and Coerce(upper limit=10.0, x=w2346, lower limit=0.0) -> (coerced(x)=w2340:dbl, In Range?=w2343:bool)
                }
                frame True {
                  n834 = Subtract(x=w2354, y=w2353) -> (x-y=w2352:dbl)
                  n835 = In Range and Coerce(upper limit=10.0, x=w2352, lower limit=0.0) -> (coerced(x)=w2348:dbl, In Range?=w2349:bool)
                }
              }
              n836 = Bundle By Name(cluster=w2338, "MTA1X"=w2335, "MTA2X"=w2334) -> (w2339:T2)
            }
            event "MTAX-": Value Change {
              n837 = event-data() -> ()  [unwired: 1 in, 1 out]
              n838 = Unbundle By Name(w2364) -> ("MTA1X"=w2363:dbl, "MTA2X"=w2362:dbl)
              n839 = case shown="False" w2359 {
                tunnel: w2363 -> [w2367 w2381]
                tunnel: [w2366 w2381] -> w2361
                tunnel: w2362 -> [w2373 w2380]
                tunnel: [w2373 w2374] -> w2360
                tunnel: w2358 -> [w2368 w2379]
                tunnel: [w2369 w2375] -> w2357
                frame False {
                  n840 = Add(x=w2367, y=w2368) -> (x+y=w2372:dbl)
                  n841 = In Range and Coerce(upper limit=10.0, x=w2372, lower limit=0.0) -> (coerced(x)=w2366:dbl, In Range?=w2369:bool)
                }
                frame True {
                  n842 = Add(x=w2380, y=w2379) -> (x+y=w2378:dbl)
                  n843 = In Range and Coerce(upper limit=10.0, x=w2378, lower limit=0.0) -> (coerced(x)=w2374:dbl, In Range?=w2375:bool)
                }
              }
              n844 = Bundle By Name(cluster=w2364, "MTA1X"=w2361, "MTA2X"=w2360) -> (w2365:T2)
            }
            event "MTAY+": Value Change {
              n845 = event-data() -> ()  [unwired: 1 in, 1 out]
              n846 = Unbundle By Name(w2390) -> ("MTA1Y"=w2389:dbl, "MTA2Y"=w2388:dbl)
              n847 = case shown="False" w2385 {
                tunnel: w2389 -> [w2393 w2407]
                tunnel: [w2392 w2407] -> w2387
                tunnel: w2388 -> [w2399 w2406]
                tunnel: [w2399 w2400] -> w2386
                tunnel: w2384 -> [w2394 w2405]
                tunnel: [w2395 w2401] -> w2383
                frame False {
                  n848 = Add(x=w2393, y=w2394) -> (x+y=w2398:dbl)
                  n849 = In Range and Coerce(upper limit=10.0, x=w2398, lower limit=0.0) -> (coerced(x)=w2392:dbl, In Range?=w2395:bool)
                }
                frame True {
                  n850 = Add(x=w2406, y=w2405) -> (x+y=w2404:dbl)
                  n851 = In Range and Coerce(upper limit=10.0, x=w2404, lower limit=0.0) -> (coerced(x)=w2400:dbl, In Range?=w2401:bool)
                }
              }
              n852 = Bundle By Name(cluster=w2390, "MTA1Y"=w2387, "MTA2Y"=w2386) -> (w2391:T2)
            }
            event "MTAY-": Value Change {
              n853 = event-data() -> ()  [unwired: 1 in, 1 out]
              n854 = Unbundle By Name(w2416) -> ("MTA1Y"=w2415:dbl, "MTA2Y"=w2414:dbl)
              n855 = case shown="False" w2411 {
                tunnel: w2415 -> [w2419 w2433]
                tunnel: [w2418 w2433] -> w2413
                tunnel: w2414 -> [w2425 w2432]
                tunnel: [w2425 w2426] -> w2412
                tunnel: w2410 -> [w2420 w2431]
                tunnel: [w2421 w2427] -> w2409
                frame False {
                  n856 = Subtract(x=w2419, y=w2420) -> (x-y=w2424:dbl)
                  n857 = In Range and Coerce(upper limit=10.0, x=w2424, lower limit=0.0) -> (coerced(x)=w2418:dbl, In Range?=w2421:bool)
                }
                frame True {
                  n858 = Subtract(x=w2432, y=w2431) -> (x-y=w2430:dbl)
                  n859 = In Range and Coerce(upper limit=10.0, x=w2430, lower limit=0.0) -> (coerced(x)=w2426:dbl, In Range?=w2427:bool)
                }
              }
              n860 = Bundle By Name(cluster=w2416, "MTA1Y"=w2413, "MTA2Y"=w2412) -> (w2417:T2)
            }
            event Key Down {
              n861 = event-data() -> ("Char"=w2435:i16, "ScanCode"=w2434:i16)  [unwired: 1 in]
              n862 = case shown="33" w2434 {
                tunnel: [w2442 w2449 w2482 w2515 w2548 w2576 w2586] -> w2441
                tunnel: w2440 -> [w2442 w2448 w2481 w2514 w2547 w2581 w2591]
                tunnel: w2439 -> [_ w2447 w2480 w2513 w2546 w2580 w2590]
                tunnel: w2438 -> [_ w2446 w2479 w2512 w2545 w2579 w2589]
                tunnel: [TRUE w2445 w2478 w2511 w2544 TRUE TRUE] -> w2437
                tunnel: w2435 -> [_ w2444 w2477 w2510 w2543 w2578 w2588]
                frame 0, Default {
                }
                frame 35 {
                  # "X+ (H)"
                  n863 = case shown="104" w2444 {
                    tunnel: [w2451 w2460] -> w2449
                    tunnel: w2448 -> [w2451 w2459]
                    tunnel: w2447 -> [_ w2454]
                    tunnel: w2446 -> [_ w2453]
                    tunnel: [TRUE w2452] -> w2445
                    frame 0, Default {
                    }
                    frame 104 {
                      n864 = Unbundle By Name(w2459) -> ("MTA1X"=w2458:dbl, "MTA2X"=w2457:dbl)
                      n865 = case shown="True" w2454 {
                        tunnel: w2458 -> [w2462 w2476]
                        tunnel: [w2461 w2476] -> w2456
                        tunnel: w2457 -> [w2468 w2475]
                        tunnel: [w2468 w2469] -> w2455
                        tunnel: w2453 -> [w2463 w2474]
                        tunnel: [w2464 w2470] -> w2452
                        frame False {
                          n866 = Add(x=w2462, y=w2463) -> (x+y=w2467:dbl)
                          n867 = In Range and Coerce(upper limit=10.0, x=w2467, lower limit=0.0) -> (coerced(x)=w2461:dbl, In Range?=w2464:bool)
                        }
                        frame True {
                          n868 = Subtract(x=w2475, y=w2474) -> (x-y=w2473:dbl)
                          n869 = In Range and Coerce(upper limit=10.0, x=w2473, lower limit=0.0) -> (coerced(x)=w2469:dbl, In Range?=w2470:bool)
                        }
                      }
                      n870 = Bundle By Name(cluster=w2459, "MTA1X"=w2456, "MTA2X"=w2455) -> (w2460:T2)
                    }
                  }
                }
                frame 33 {
                  # "X- (F)"
                  n871 = case shown="102" w2477 {
                    tunnel: [w2484 w2493] -> w2482
                    tunnel: w2481 -> [w2484 w2492]
                    tunnel: w2480 -> [_ w2487]
                    tunnel: w2479 -> [_ w2486]
                    tunnel: [TRUE w2485] -> w2478
                    frame 0, Default {
                    }
                    frame 102 {
                      n872 = Unbundle By Name(w2492) -> ("MTA1X"=w2491:dbl, "MTA2X"=w2490:dbl)
                      n873 = case shown="True" w2487 {
                        tunnel: w2491 -> [w2495 w2509]
                        tunnel: [w2494 w2509] -> w2489
                        tunnel: w2490 -> [w2501 w2508]
                        tunnel: [w2501 w2502] -> w2488
                        tunnel: w2486 -> [w2496 w2507]
                        tunnel: [w2497 w2503] -> w2485
                        frame False {
                          n874 = Subtract(x=w2495, y=w2496) -> (x-y=w2500:dbl)
                          n875 = In Range and Coerce(upper limit=10.0, x=w2500, lower limit=0.0) -> (coerced(x)=w2494:dbl, In Range?=w2497:bool)
                        }
                        frame True {
                          n876 = Add(x=w2508, y=w2507) -> (x+y=w2506:dbl)
                          n877 = In Range and Coerce(upper limit=10.0, x=w2506, lower limit=0.0) -> (coerced(x)=w2502:dbl, In Range?=w2503:bool)
                        }
                      }
                      n878 = Bundle By Name(cluster=w2492, "MTA1X"=w2489, "MTA2X"=w2488) -> (w2493:T2)
                    }
                  }
                }
                frame 20 {
                  # "Y+ (T)"
                  n879 = case shown="116" w2510 {
                    tunnel: [w2516 w2526] -> w2515
                    tunnel: w2514 -> [w2516 w2525]
                    tunnel: w2513 -> [_ w2520]
                    tunnel: w2512 -> [_ w2519]
                    tunnel: [TRUE w2518] -> w2511
                    frame 0, Default {
                    }
                    frame 116 {
                      n880 = Unbundle By Name(w2525) -> ("MTA1Y"=w2524:dbl, "MTA2Y"=w2523:dbl)
                      n881 = case shown="False" w2520 {
                        tunnel: w2524 -> [w2528 w2542]
                        tunnel: [w2527 w2542] -> w2522
                        tunnel: w2523 -> [w2534 w2541]
                        tunnel: [w2534 w2535] -> w2521
                        tunnel: w2519 -> [w2529 w2540]
                        tunnel: [w2530 w2536] -> w2518
                        frame False {
                          n882 = Add(x=w2528, y=w2529) -> (x+y=w2533:dbl)
                          n883 = In Range and Coerce(upper limit=10.0, x=w2533, lower limit=0.0) -> (coerced(x)=w2527:dbl, In Range?=w2530:bool)
                        }
                        frame True {
                          n884 = Add(x=w2541, y=w2540) -> (x+y=w2539:dbl)
                          n885 = In Range and Coerce(upper limit=10.0, x=w2539, lower limit=0.0) -> (coerced(x)=w2535:dbl, In Range?=w2536:bool)
                        }
                      }
                      n886 = Bundle By Name(cluster=w2525, "MTA1Y"=w2522, "MTA2Y"=w2521) -> (w2526:T2)
                    }
                  }
                }
                frame 34 {
                  # "Y- (G)"
                  n887 = case shown="0, Default" w2543 {
                    tunnel: [w2549 w2559] -> w2548
                    tunnel: w2547 -> [w2549 w2558]
                    tunnel: w2546 -> [_ w2553]
                    tunnel: w2545 -> [_ w2552]
                    tunnel: [TRUE w2551] -> w2544
                    frame 0, Default {
                    }
                    frame 103 {
                      n888 = Unbundle By Name(w2558) -> ("MTA1Y"=w2557:dbl, "MTA2Y"=w2556:dbl)
                      n889 = case shown="True" w2553 {
                        tunnel: w2557 -> [w2561 w2575]
                        tunnel: [w2560 w2575] -> w2555
                        tunnel: w2556 -> [w2567 w2574]
                        tunnel: [w2567 w2568] -> w2554
                        tunnel: w2552 -> [w2562 w2573]
                        tunnel: [w2563 w2569] -> w2551
                        frame False {
                          n890 = Subtract(x=w2561, y=w2562) -> (x-y=w2566:dbl)
                          n891 = In Range and Coerce(upper limit=10.0, x=w2566, lower limit=0.0) -> (coerced(x)=w2560:dbl, In Range?=w2563:bool)
                        }
                        frame True {
                          n892 = Subtract(x=w2574, y=w2573) -> (x-y=w2572:dbl)
                          n893 = In Range and Coerce(upper limit=10.0, x=w2572, lower limit=0.0) -> (coerced(x)=w2568:dbl, In Range?=w2569:bool)
                        }
                      }
                      n894 = Bundle By Name(cluster=w2558, "MTA1Y"=w2555, "MTA2Y"=w2554) -> (w2559:T2)
                    }
                  }
                }
                frame 19 {
                  # "MTA switch (R)"
                  n895 = case shown="114" w2578 {
                    tunnel: w2581 -> [w2582 w2585]
                    tunnel: w2580 -> [_ w2584]
                    tunnel: w2579 -> [_ _]
                    tunnel: [w2582 w2585] -> w2576
                    frame 0, Default {
                    }
                    frame 114 {
                      n896 = Not(x=w2584) -> (.not. x?=w2583:bool)
                      n897 = local write "MTA_Select"(w2583) -> ()
                    }
                  }
                }
                frame 21 {
                  # "MTA step (Y)"
                  n898 = case shown="121" w2588 {
                    tunnel: w2591 -> [w2592 w2595]
                    tunnel: w2590 -> [_ _]
                    tunnel: w2589 -> [_ _]
                    tunnel: [w2592 w2595] -> w2586
                    frame 0, Default {
                    }
                    frame 121 {
                      n899 = local read "MTA_Step_Select"() -> (w2594:bool)
                      n900 = Not(x=w2594) -> (.not. x?=w2593:bool)
                      n901 = local write "MTA_Step_Select"(w2593) -> ()
                    }
                  }
                }
              }
            }
            event Key Repeat {
              n902 = event-data() -> ("Char"=w2600:i16, "ScanCode"=w2599:i16)  [unwired: 1 in]
              n903 = Divide(x=1000.0, y="PZT_Speed 2") -> (x/y=w2598:dbl)
              n904 = Wait (ms)(milliseconds to wait=w2598) -> ()  [unwired: 1 out]
              n905 = case shown="35" w2599 {
                tunnel: [w2607 w2614 w2647 w2680 w2713] -> w2606
                tunnel: w2605 -> [w2607 w2613 w2646 w2679 w2712]
                tunnel: w2604 -> [_ w2612 w2645 w2678 w2711]
                tunnel: w2603 -> [_ w2611 w2644 w2677 w2710]
                tunnel: [TRUE w2610 w2643 w2676 w2709] -> w2602
                tunnel: w2600 -> [_ w2609 w2642 w2675 w2708]
                frame 0, Default {
                }
                frame 35 {
                  # "X+ (H)"
                  n906 = case shown="104" w2609 {
                    tunnel: [w2616 w2625] -> w2614
                    tunnel: w2613 -> [w2616 w2624]
                    tunnel: w2612 -> [_ w2619]
                    tunnel: w2611 -> [_ w2618]
                    tunnel: [TRUE w2617] -> w2610
                    frame 0, Default {
                    }
                    frame 104 {
                      n907 = Unbundle By Name(w2624) -> ("MTA1X"=w2623:dbl, "MTA2X"=w2622:dbl)
                      n908 = case shown="True" w2619 {
                        tunnel: w2623 -> [w2627 w2641]
                        tunnel: [w2626 w2641] -> w2621
                        tunnel: w2622 -> [w2633 w2640]
                        tunnel: [w2633 w2634] -> w2620
                        tunnel: w2618 -> [w2628 w2639]
                        tunnel: [w2629 w2635] -> w2617
                        frame False {
                          n909 = Add(x=w2627, y=w2628) -> (x+y=w2632:dbl)
                          n910 = In Range and Coerce(upper limit=10.0, x=w2632, lower limit=0.0) -> (coerced(x)=w2626:dbl, In Range?=w2629:bool)
                        }
                        frame True {
                          n911 = Subtract(x=w2640, y=w2639) -> (x-y=w2638:dbl)
                          n912 = In Range and Coerce(upper limit=10.0, x=w2638, lower limit=0.0) -> (coerced(x)=w2634:dbl, In Range?=w2635:bool)
                        }
                      }
                      n913 = Bundle By Name(cluster=w2624, "MTA1X"=w2621, "MTA2X"=w2620) -> (w2625:T2)
                    }
                  }
                }
                frame 33 {
                  # "X- (F)"
                  n914 = case shown="102" w2642 {
                    tunnel: [w2649 w2658] -> w2647
                    tunnel: w2646 -> [w2649 w2657]
                    tunnel: w2645 -> [_ w2652]
                    tunnel: w2644 -> [_ w2651]
                    tunnel: [TRUE w2650] -> w2643
                    frame 0, Default {
                    }
                    frame 102 {
                      n915 = Unbundle By Name(w2657) -> ("MTA1X"=w2656:dbl, "MTA2X"=w2655:dbl)
                      n916 = case shown="True" w2652 {
                        tunnel: w2656 -> [w2660 w2674]
                        tunnel: [w2659 w2674] -> w2654
                        tunnel: w2655 -> [w2666 w2673]
                        tunnel: [w2666 w2667] -> w2653
                        tunnel: w2651 -> [w2661 w2672]
                        tunnel: [w2662 w2668] -> w2650
                        frame False {
                          n917 = Subtract(x=w2660, y=w2661) -> (x-y=w2665:dbl)
                          n918 = In Range and Coerce(upper limit=10.0, x=w2665, lower limit=0.0) -> (coerced(x)=w2659:dbl, In Range?=w2662:bool)
                        }
                        frame True {
                          n919 = Add(x=w2673, y=w2672) -> (x+y=w2671:dbl)
                          n920 = In Range and Coerce(upper limit=10.0, x=w2671, lower limit=0.0) -> (coerced(x)=w2667:dbl, In Range?=w2668:bool)
                        }
                      }
                      n921 = Bundle By Name(cluster=w2657, "MTA1X"=w2654, "MTA2X"=w2653) -> (w2658:T2)
                    }
                  }
                }
                frame 20 {
                  # "Y+ (T)"
                  n922 = case shown="116" w2675 {
                    tunnel: [w2681 w2691] -> w2680
                    tunnel: w2679 -> [w2681 w2690]
                    tunnel: w2678 -> [_ w2685]
                    tunnel: w2677 -> [_ w2684]
                    tunnel: [TRUE w2683] -> w2676
                    frame 0, Default {
                    }
                    frame 116 {
                      n923 = Unbundle By Name(w2690) -> ("MTA1Y"=w2689:dbl, "MTA2Y"=w2688:dbl)
                      n924 = case shown="False" w2685 {
                        tunnel: w2689 -> [w2693 w2707]
                        tunnel: [w2692 w2707] -> w2687
                        tunnel: w2688 -> [w2699 w2706]
                        tunnel: [w2699 w2700] -> w2686
                        tunnel: w2684 -> [w2694 w2705]
                        tunnel: [w2695 w2701] -> w2683
                        frame False {
                          n925 = Add(x=w2693, y=w2694) -> (x+y=w2698:dbl)
                          n926 = In Range and Coerce(upper limit=10.0, x=w2698, lower limit=0.0) -> (coerced(x)=w2692:dbl, In Range?=w2695:bool)
                        }
                        frame True {
                          n927 = Add(x=w2706, y=w2705) -> (x+y=w2704:dbl)
                          n928 = In Range and Coerce(upper limit=10.0, x=w2704, lower limit=0.0) -> (coerced(x)=w2700:dbl, In Range?=w2701:bool)
                        }
                      }
                      n929 = Bundle By Name(cluster=w2690, "MTA1Y"=w2687, "MTA2Y"=w2686) -> (w2691:T2)
                    }
                  }
                }
                frame 34 {
                  # "Y- (G)"
                  n930 = case shown="0, Default" w2708 {
                    tunnel: [w2714 w2724] -> w2713
                    tunnel: w2712 -> [w2714 w2723]
                    tunnel: w2711 -> [_ w2718]
                    tunnel: w2710 -> [_ w2717]
                    tunnel: [TRUE w2716] -> w2709
                    frame 0, Default {
                    }
                    frame 103 {
                      n931 = Unbundle By Name(w2723) -> ("MTA1Y"=w2722:dbl, "MTA2Y"=w2721:dbl)
                      n932 = case shown="True" w2718 {
                        tunnel: w2722 -> [w2726 w2740]
                        tunnel: [w2725 w2740] -> w2720
                        tunnel: w2721 -> [w2732 w2739]
                        tunnel: [w2732 w2733] -> w2719
                        tunnel: w2717 -> [w2727 w2738]
                        tunnel: [w2728 w2734] -> w2716
                        frame False {
                          n933 = Subtract(x=w2726, y=w2727) -> (x-y=w2731:dbl)
                          n934 = In Range and Coerce(upper limit=10.0, x=w2731, lower limit=0.0) -> (coerced(x)=w2725:dbl, In Range?=w2728:bool)
                        }
                        frame True {
                          n935 = Subtract(x=w2739, y=w2738) -> (x-y=w2737:dbl)
                          n936 = In Range and Coerce(upper limit=10.0, x=w2737, lower limit=0.0) -> (coerced(x)=w2733:dbl, In Range?=w2734:bool)
                        }
                      }
                      n937 = Bundle By Name(cluster=w2723, "MTA1Y"=w2720, "MTA2Y"=w2719) -> (w2724:T2)
                    }
                  }
                }
              }
            }
          }
          n938 = Not(x=w2206) -> (.not. x?=→"MTA_Limit":bool)
          n939 = Unbundle By Name(w2201) -> ("MTA1X"=w2214:dbl, "MTA1Y"=w2213:dbl, "MTA2X"=w2212:dbl, "MTA2Y"=w2211:dbl)
          "MTA1Y" <- w2213
          "MTA1X" <- w2214
          "MTA2X" <- w2212
          "MTA2Y" <- w2211
          n940 = case shown="True" "PM_Feedback" {
            tunnel: [w2231 w2251] -> w2217
            tunnel: w2216 -> [w2227 _]
            tunnel: w2214 -> [w2230 w2246]
            tunnel: w2213 -> [w2229 w2245]
            tunnel: w2212 -> [_ _]
            tunnel: w2211 -> [_ _]
            tunnel: w2201 -> [w2226 w2250]
            tunnel: [w2226 w2247] -> w2202
            frame False {
              # "Manual mode"
              n941 = Build Array(w2230, w2229) -> (w2228:dbl[])
              n942 = case shown="True" w2227 {
                tunnel: [errorcluster {"status"=FALSE, "code"=0, "source"=""} ("error out") w2234] -> w2231
                tunnel: w2228 -> [_ w2235]
                frame False {
                }
                frame True {
                  n943 = call-poly <vilib>:"DAQmx Create Virtual Channel.vi"("maximum value"=10.0, "minimum value"=0.0, "physical channels"=tag "Dev2/ao0:1") -> ("task out"=w2244:refnum<k21>, "error out"=w2243:errorcluster)  [unwired: 11 in]
                  n944 = call <vilib>:"DAQmx Start Task.vi"("task/channels in"=w2244, "error in"=w2243) -> ("task out"=w2237:refnum<k21>, "error out"=w2236:errorcluster)  [unwired: 12 in]
                  n945 = call-poly <vilib>:"DAQmx Write.vi"("task/channels in"=w2237, "data"=w2235, "error in"=w2236) -> ("task out"=w2239:refnum<k21>, "error out"=w2238:errorcluster)  [unwired: 10 in, 1 out]
                  n946 = call <vilib>:"DAQmx Clear Task.vi"("task in"=w2239, "error in"=w2238) -> ("error out"=w2233:errorcluster)  [unwired: 13 in]
                  n947 = Merge Errors(w2233) -> (w2234:errorcluster)
                }
              }
            }
            frame True {
              # "Force feedback mode"
              n948 = call-poly <vilib>:"DAQmx Create Virtual Channel.vi"("maximum value"=10.0, "minimum value"=0.0, "physical channels"=tag "Dev2/ao0:1") -> ("task out"=w2259:refnum<k21>, "error out"=w2260:errorcluster)  [unwired: 11 in]
              n949 = call <vilib>:"DAQmx Start Task.vi"("task/channels in"=w2259, "error in"=w2260) -> ("task out"=w2255:refnum<k21>, "error out"=w2254:errorcluster)  [unwired: 12 in]
              n950 = while {
                tunnel: w2255 -> [w2271]
                tunnel: w2254 -> [w2270]
                tunnel: [w2269] -> w2252
                tunnel: [w2268] -> w2253
                shift-right: [w2262] -> w2248
                shift-left: w2245 -> [w2264]
                shift-right: [w2263] -> w2249
                shift-left: w2246 -> [w2265]
                i -> [w2272]
                stop <- w2267 continue-if-true
                n951 = stacked-sequence {
                  tunnel: w2265 -> [w2281 w2306]
                  tunnel: w2264 -> [w2280 w2305]
                  tunnel: [w2279 _] -> w2263
                  tunnel: [_ w2304] -> w2262
                  frame #0 {
                    n952 = global read "Feedback.vi" "Fx"() -> (w2278:dbl)
                    n953 = Absolute Value(x=w2278) -> (abs(x)=w2277:dbl)
                    n954 = Greater?(x=w2277, y="MTAx_Feedback_Min") -> (0:w2273:bool)
                    n955 = And(x=w2273, y="MTAx_Feedback_ON") -> (x .and. y?=w2274:bool)
                    n956 = case shown="True" w2274 {
                      tunnel: w2281 -> [w2282 _]
                      tunnel: w2280 -> [_ _]
                      tunnel: [w2282 w2286] -> w2279
                      frame False {
                      }
                      frame True {
                        w2290 = 5.0 ("output low")
                        n957 = Divide(x="MTAx_Feedback_Max", y=1.4) -> (x/y=w2294:dbl)
                        n958 = Divide(x="?", y=cluster{dbl, dbl, dbl} {1000.0, 60.0, 60.0}) -> (x/y=w2284:cluster{dbl, dbl, dbl})
                        n959 = Subtract(x=w2290, y=w2294) -> (x-y=w2296:dbl)
                        n960 = Add(x=w2290, y=w2294) -> (x+y=w2295:dbl)
                        n961 = global read "Feedback.vi" "Fx"() -> (w2292:dbl)
                        n962 = Bundle(w2295, w2296) -> (w2297:cluster{dbl, dbl})  [unwired: 1 in]
                        n963 = call-poly <vilib>:"PID.vi"("reinitialize? (F)"="MTAx_Feedback_Reset", "output range"=w2297, "dt (s)"="MTAx_Feedback_dt", "PID gains"=w2284, "process variable"=w2292, "setpoint"="MTAx_Feedback_Force") -> ("output"=w2286:dbl)  [unwired: 4 in, 1 out]
                      }
                    }
                  }
                  frame #1 {
                    n964 = global read "Feedback.vi" "Fx"() -> (w2300:dbl)
                    n965 = Absolute Value(x=w2300) -> (abs(x)=w2301:dbl)
                    n966 = Greater?(x=w2301, y="MTAy_Feedback_Min") -> (0:w2298:bool)
                    n967 = And(x=w2298, y="MTAy_Feedback_ON") -> (x .and. y?=w2303:bool)
                    n968 = case shown="True" w2303 {
                      tunnel: w2306 -> [_ _]
                      tunnel: w2305 -> [w2307 _]
                      tunnel: [w2307 w2311] -> w2304
                      frame False {
                      }
                      frame True {
                        w2315 = 5.0 ("output low")
                        n969 = Divide(x="MTAy_Feedback_Max", y=1.0) -> (x/y=w2319:dbl)
                        n970 = Divide(x="?", y=cluster{dbl, dbl, dbl} {-1000.0, 60.0, 60.0}) -> (x/y=w2308:cluster{dbl, dbl, dbl})
                        n971 = Add(x=w2315, y=w2319) -> (x+y=w2320:dbl)
                        n972 = Subtract(x=w2315, y=w2319) -> (x-y=w2321:dbl)
                        n973 = global read "Feedback.vi" "Fy"() -> (w2318:dbl)
                        n974 = Bundle(w2320, w2321) -> (w2322:cluster{dbl, dbl})  [unwired: 1 in]
                        n975 = call-poly <vilib>:"PID.vi"("reinitialize? (F)"="MTAy_Feedback_Reset", "output range"=w2322, "dt (s)"="MTAy_Feedback_dt", "PID gains"=w2308, "process variable"=w2318, "setpoint"="MTAy_Feedback_Force") -> ("output"=w2311:dbl)  [unwired: 4 in, 1 out]
                      }
                    }
                  }
                }
                n976 = local read "PM_Feedback"() -> (w2267:bool)
                n977 = Build Array(w2263, w2262) -> (w2261:dbl[])
                n978 = Wait (ms)(milliseconds to wait=u32 1) -> ()  [unwired: 1 out]
                n979 = call-poly <vilib>:"DAQmx Write.vi"("task/channels in"=w2271, "data"=w2261, "error in"=w2270) -> ("task out"=w2269:refnum<k21>, "error out"=w2268:errorcluster)  [unwired: 10 in, 1 out]
                "MTA_Os_Num" <- w2272
              }
              n980 = Bundle By Name(cluster=w2250, "MTA1X"=w2249, "MTA1Y"=w2248) -> (w2247:T2)
              n981 = call <vilib>:"DAQmx Clear Task.vi"("task in"=w2252, "error in"=w2253) -> ("error out"=w2251:errorcluster)  [unwired: 13 in]
            }
          }
          n982 = Merge Errors(w2217, w2218) -> (w2219:errorcluster)
          n983 = Or(x="MTA_STOP", y=w2219) -> (x .or. y?=w2221:bool)
          n984 = Not(x=w2221) -> (.not. x?=→"MTA_ON":bool)
          n985 = Wait (ms)(milliseconds to wait=u32 100) -> ()  [unwired: 1 out]
          "MTA_Man_Num" <- w2223
        }
      }
    }
    n986 = local read "STOP"() -> (w2194:bool)
    n987 = Wait (ms)(milliseconds to wait=u32 100) -> ()  [unwired: 1 out]
    "MTA_Manual_ON" <- "MTA_START"
  }
  n988 = while {
    shift-right: [w2742] -> w36
    shift-left: w2 -> [w2745]
    stop <- w2744 stop-if-true
    # "DetectionLaser-Power"
    n989 = case shown="True" "Detection_Power_START" {
      tunnel: w2745 -> [w2747 w2750]
      tunnel: [w2747 w2748] -> w2742
      frame False {
      }
      frame True {
        n990 = call-poly <vilib>:"DAQmx Create Virtual Channel.vi"("maximum value"=0.4, "minimum value"=0.0, "physical channels"=tag "Dev1/ao1") -> ("task out"=w2755:refnum<k21>, "error out"=w2759:errorcluster)  [unwired: 11 in]
        n991 = call <vilib>:"DAQmx Start Task.vi"("task/channels in"=w2755, "error in"=w2759) -> ("task out"=w2754:refnum<k21>, "error out"=w2753:errorcluster)  [unwired: 12 in]
        n992 = while "Event Handle Loop" {
          shift-right: [w2762] -> w2752
          shift-left: w2754 -> [w2764]
          shift-right: [w2760] -> w2751
          shift-left: w2753 -> [w2763]
          i -> [w2770]
          stop <- w2768 stop-if-true
          # "Detection Laser"
          n993 = case shown="True" "Detection_Power_Run" {
            tunnel: [0.0 ("y") w2777] -> w2765
            frame False {
            }
            frame True {
              n994 = Multiply(x="Detection_Power", y=4.0) -> (x*y=w2773:dbl)
              n995 = Add(x=w2773, y=150.0) -> (x+y=w2776:dbl)
              n996 = Divide(x=w2776, y=3000.0) -> (x/y=w2777:dbl)
            }
          }
          n997 = call-poly <vilib>:"DAQmx Write.vi"("task/channels in"=w2764, "data"=w2765, "error in"=w2763) -> ("task out"=w2762:refnum<k21>, "error out"=w2760:errorcluster)  [unwired: 10 in, 1 out]
          n998 = Wait (ms)(milliseconds to wait=u32 100) -> ()  [unwired: 1 out]
          n999 = Or(x=w2760, y="Detection_Power_STOP") -> (x .or. y?=w2768:bool)
          n1000 = Not(x=w2768) -> (.not. x?=→"Detection_Power_ON":bool)
          "Det_Power_Num" <- w2770
        }
        n1001 = call <vilib>:"DAQmx Clear Task.vi"("task in"=w2752, "error in"=w2751) -> ("error out"=w2749:errorcluster)  [unwired: 13 in]
        n1002 = Merge Errors(w2749, w2750) -> (w2748:errorcluster)
      }
    }
    n1003 = local read "STOP"() -> (w2743:bool)
    n1004 = Or(x=w2743, y=w2742) -> (x .or. y?=w2744:bool)
    n1005 = Wait (ms)(milliseconds to wait=u32 100) -> ()  [unwired: 1 out]
  }
  n1006 = Merge Errors(w32, w31, w23, w1) -> (w30:errorcluster)
  n1007 = Unbundle By Name(w46) -> ("PZT_X"=w49:dbl, "PZT_Y"=w48:dbl, "PZT_Z"=w47:dbl)
  n1008 = Build Array(w49, w48, w47) -> (w45:dbl[])
  n1009 = call "Convert to Dynamic Data"("Array"=w45) -> ("Dynamic Data Type"=w58:dynamicdata)  [unwired: 3 in]
  n1010 = call "Write To Measurement File"("Signals"=w58) -> ()  [unwired: 16 in, 3 out]
  n1011 = Merge Errors(w34, w33, w30) -> (w35:errorcluster)
  n1012 = Merge Errors(w42, w40, w35) -> (w38:errorcluster)
  n1013 = Unbundle By Name(w4) -> ("MTA1X"=w8:dbl, "MTA1Y"=w7:dbl, "MTA2X"=w6:dbl, "MTA2Y"=w3:dbl)
  n1014 = Merge Errors(w22, w60, w59, w41, w36) -> (w39:errorcluster)
  n1015 = Merge Errors(w39, w38) -> (w37:errorcluster)
  n1016 = Build Array(w8, w7, w6, w3) -> (w5:dbl[])
  n1017 = call <vilib>:"Simple Error Handler.vi"("error in (no error)"=w37) -> ("error out"=w25:errorcluster)  [unwired: 4 in, 4 out]
  n1018 = call "Convert to Dynamic Data4"("Array"=w5) -> ("Dynamic Data Type"=w9:dynamicdata)  [unwired: 3 in]
  n1019 = call "Write To Measurement File4"("Signals"=w9) -> ()  [unwired: 16 in, 3 out]
  n1020 = Unbundle By Name(w25) -> ("status"=w24:bool)
  n1021 = local write "Controllers_ON"(w24) -> ()
